vi "AlliGator Settings Window.vi"() -> ()   [LabVIEW 2021, in "AlliGator Settings.lvlib"]
doc: "GUI providing access to settings parameters for all aspect of AlliGator's functions."
uses:
  AlliGator Settings.lvlib
  AlliGator Phasor Plot Size.ctl
  AlliGator Gates to Skip.ctl
  Graphs/XY Graph/XY Graph Plot Shift Parameters.ctl
  Graphs/XY Graph/XY Graph Plot Shift Method.ctl
  Image/Image Save File Format.ctl
  AlliGator Low Count Pixels Rejection Options.ctl
  Phasor/Phasor Ratio Type.ctl
  AlliGator Baseline Subtraction Method.ctl
  Fits/IRF(X)PSED/Decay Fit Options v2.ctl
  Fits/Decay Convolution/Decay Model.ctl
  Fits/Residual Type.ctl
  Fits/IRF(X)PSED/Fit Weights Type.ctl
  Fits/Non-linear Fitting Method v2.ctl
  Fits/Fit Calculation Method.ctl
  Fits/Non-linear Fitting Algorithm.ctl
  Fits/IRF(X)PSED/Decay Fit Parameters & Derived Quantities List.ctl
  AlliGator Decay Fit Parameter Constraints 2.ctl
  Fits/IRF(X)PSED/Decay Fit Parameters In List.ctl
  AlliGator IRF Optimization Controls.ctl
  AlliGator IRF Deconvolution Metrics.ctl
  Math/Advanced Signal Processing Toolkit/Wavelet Analysis Options.ctl
  AlliGator High Count Pixels Rejection Options.ctl
  AlliGator Image Smoothing Options.ctl
  Arrays/Kernel Type.ctl
  Arrays/Smoothing Algorithm.ctl
  Fits/Square Pulse/Square Pulse Options.ctl
  Fits/Square Pulse/Square Pulse Levels Type.ctl
  AlliGator Image Binning Options.ctl
  AlliGator Phasor Plot Smoothing Options.ctl
  AlliGator Phasor Plot Graphics Options.ctl
  AlliGator Exported Image Settings.ctl
  Fits/IRF(X)PSED/IRF(X)PSED Extraction Options.ctl
  Fits/IRF(X)PSED/Fourier Series Smoothing Option.ctl
  Fits/IRF(X)PSED/Fourier Series Truncation.ctl
  Fits/IRF(X)PSED/IRF Extraction Method.ctl
  Phasor/Phasor Explorer Display Parameters.ctl
  Phasor/Phasor Type of Series.ctl
  Phasor/Phasor Explorer Decay Parameters.ctl
  Phasor/Phasor IRF Model.ctl
  Phasor/Phasor Explorer Phasor Parameters.ctl
  Phasor/Phasor Calculation Type.ctl
  Phasor/Phasor SEPL Type.ctl
  Phasor/Phasor Explorer Gate Parameters.ctl
  Phasor/Phasor Gate Type.ctl
  Phasor/Phasor Type of User-defined Function.ctl
  Phasor/Phasor Explorer Gate Parameter to Adjust.ctl
  AlliGator Define Gates to.ctl
  AlliGator Gates to Keep.ctl
  AlliGator Phasor Ratio Color-Coded Quantity.ctl
  Phasor/Phasor Calibration Type.ctl
  Histograms/Linear Histogram Options.ctl
  Histograms/Histogram Bin Option.ctl
  Histograms/Histogram Bin Position.ctl
  AlliGator Gate Arithmetic.ctl
  AlliGator Phasor Reference Associated with Shortest Lifetime.ctl
  AlliGator Python Settings.ctl
  SwissSPAD/SwissSPAD Live_Image Display Options.ctl
  AlliGator Average Lifetime Options.ctl
  AlliGator Calibration Map Algorithm.ctl
  AlliGator Guess Parameters Options.ctl
  Phasor/Phasor Standard Deviation Options.ctl
  AlliGator Source Image Scale Bar Options.ctl
  Fits/IRF(X)PSED/MLE Baseline Offset Type.ctl
  Image/Flatfield Correction Options.ctl
  AlliGator Settings Q Element.ctl
  AlliGator Settings Q Action.ctl
  AlliGator Refnums List.ctl
  AlliGator Settings List.ctl
  AlliGator Variables List.ctl
  Image/Image Hot Pixel Map Target.ctl
  AlliGator Q Element.ctl
  AlliGator Q Event.ctl
  Palette/Image Palette Information.ctl
  Image/Image Display Palette Type.ctl
  Notebook/Notebook Parameters List.ctl
  AlliGator Skippable Windows Status.ctl
  AlliGator Quantities.ctl
  f3e5a785-d283-42c9-a630-fb32b7f70655.vi
  c46dad3f-f40e-47bf-8043-7fc63249f95d.vi
  Variant/Variant to Data/Variant to [String].vi
  Variant/Variant to Data/Variant to I32.vi
  Variant/Variant to Data/Variant to Boolean.vi
  Formula/Aliases Definition Window.vi
  Variant/Variant to Data/Variant to U16.vi
  Variant/Variant to Data/Variant to String.vi
  Variant/Variant to Data/Variant to Path.vi
  AlliGator Action Engine.lvlib
  AlliGator Globals, Variables & Constants.lvlib
  Variant/Variant to Data/Variant to Data.lvlib
  Palette/Palette.lvlib
  Image/Image.lvlib
  AlliGator GUI.lvlib
  AlliGator Phasor Plot.lvlib
  AlliGator Phasor Graph.lvlib
  Error/Error.lvlib
  Graphs/Plot Editor/Plot Editor.lvlib
  Phasor/Phasor Explorer.lvlib
  AlliGator Phasor Ratio.lvlib
  Utilities/Utilities.lvlib
  <vilib>/vision/NI_Vision_Development_Module.lvlib
  AlliGator Python Plugins.lvlib
  Notebook/Notebook.lvlib
  SwissSPAD/SwissSPAD Live.lvlib
  Formula/Formula.lvlib
  Fits/Fits.lvlib
  Phasor/Phasor.lvlib
  AlliGator Decay Analysis.lvlib
  Graphs/XY Graph/XY Graph Add-Ons.lvlib
  AlliGator Decay Fit.lvlib
  AlliGator IRF.lvlib
  Math/Math.lvlib
  Arrays/Arrays.lvlib
  AlliGator Source Image.lvlib
  Histograms/Histogram Window.lvlib
  AlliGator Phasor Calibration.lvlib
  AlliGator Decay Preprocessing.lvlib
panel:
  in  "Flatfield Correction":T1={"Flatfield Estimation Options"={"Sampling Grid Size X"=256, "Sampling Grid Size Y"=256, "Polynomial Degree"=5}, "Background Options"={"Estimate Background"=TRUE, "Background Estimation Size"=32, "Niblack Deviation Factor [0. 1]"=0.2}, "Correction Factor"=1.1} {"Background Options"."Niblack Deviation Factor [0. 1]" min=0.0 max=1.0}
  in  "Settings Tabs":T2(tab)
  in  "Source Image Tabs":T3(tab)
  in  "Hot Pixel Removal":T4 caption="Hot Pixel Removal (*)" {"Percentile" min=0 max=100}
  in  "Use Image Histogram for Contrast":bool=TRUE
  in  "Low Count Pixels Rejection Options":T5={"Background Low Threshold Factor"=0.0, "Fixed Low Background Threshold"=20000.0, "Reject Low Count Pixels"=FALSE, "Low Percentile"=0.0} {"Low Percentile" min=0.0 max=100.0}
  in  "High Count Pixels Rejection Options":T6={"Background High Threshold Factor"=0.0, "Fixed High Background Threshold"=1.0, "Reject High Count Pixels"=FALSE, "High Percentile"=100.0} {"High Percentile" min=0.0 max=100.0}
  in  "ROI Creation":string="ROI Creation"
  in  "Image Pre-Processing Operations Order":u16(ring) items=["Remove Screamers", "Pile-up Correction", "Binning", "Smoothing", "Rescaling"]
  in  "Dead Left Columns Correction":bool
  in  "ROI Diameter":i32=12
  in  "Use Fixed ROI Diameter":bool
  in  "ROI Center Color":u32(colorbox)=16711680
  in  "Peak Threshold":dbl=500.0
  in  "Image Smoothing Options":T7={"Use Image Smoothing"=FALSE, "Kernel Type"=enum."Bilinear", "Bin"=1, "Algorithm"=enum."Rapid"} caption="Image Smoothing Options (*)" {"Bin" min=1}
  in  "Image Binning Options":T10={"Use Image Binning"=FALSE, "X Bin"=1, "Y Bin"=1} caption="Image Binning Options (*)" {"Y Bin" min=1; "X Bin" min=1}
  in  "Invert Binary Mask":bool
  in  "Intensity Threshold":dbl=500.0
  in  "Overlay Analyzed ROI Center":bool
  in  "Save Source Image":bool caption="Save Image"
  in  "Use Image Brightness":bool=TRUE
  in  "Blend Overlay with Image Background":bool=TRUE
  in  "Scale Bar Options":T11 caption="Scale Bar Options (*)"
  in  "Image Resolution (Pixel Size)":dbl[unit]
  in  "Dataset Scaling Factor":dbl=1.0 caption="Scaling Factor" min=0.0
  in  "Gate Image Integration":dbl[unit]=3e-10 min=0.0 format="%#.3g"
  in  "Gate Image Exposure":dbl[unit]=3e-10 min=0.0 format="%#.3g"
  in  "Available Channel Names":string[](array[string])
  in  "Background File Subtraction":bool
  in  "Background Scaling Factor":dbl=1.0 caption="Scaling Factor" min=0.0
  in  "Background File":path caption="Background Dataset"
  in  "Background Pile-up Correction":bool caption="Pile-up Correction"
  in  "Background Pixel Well Capacity":u32=1 caption="Max Value" min=1 step=1
  in  "Pixel Well Capacity":u32=1 caption="Max Value" min=1 step=1
  in  "Pile-up Correction":bool
  in  "Channel Arithmetic":T12 caption="Channel Arithmetic (*)"
  in  "Channel Name":u16(ring) items=["Gate"]
  in  "Gates to Keep":T13={"First"=0, "Last"=4294967295} caption="Gates to Keep (*)"
  in  "Define Gates to":T14 caption="Define Gates to (*)"
  in  "SYNC Period":dbl[unit] min=0.0 format="%#.3g"
  out "Natural Frequency":dbl[unit] min=0.0 format="%#.3g"
  in  "# Gates":u32=1 min=1 step=1
  in  "Gate Step":u32=1 caption="Gate Step (*)" min=1 step=1
  in  "Gate Width":dbl[unit]=3e-10 min=0.0 format="%#.3g"
  in  "Nanotime Gate Separation":dbl[unit]=4e-11 caption="Gate Separation" min=0.0 format="%#.3g"
  in  "Gates to Skip":T15 caption="Gates to Skip (*)"
  in  "Laser Period":dbl[unit] min=0.0 format="%#.3g"
  in  "Fluorescence Decay Tabs":T16(tab) caption="Fluorescence Decay Tab"
  in  "[0-1]-Normalize Decay":bool caption="1- Normalize Decay"
  in  "# Folds":u32=1 min=1
  in  "Fold Decay":bool caption="Straighten Decay"
  in  "Use Decay Pre-Processing":bool=TRUE
  in  "Head Fraction":dbl min=0.0 max=1.0 format="%.4g"
  in  "Use Cursors":bool
  in  "Use Periodicity":bool
  in  "Pixel-Normalize Decay":bool
  in  "Constant Background":dbl=1.0
  in  "Verbose Decay Pre-Processing":bool=TRUE
  in  "Decay Pre-Processing Operations Order":u16(ring) items=["Background subtraction", "Revert", "Smoothen", "Straighten", "Shift", "Extrapolate", "Normalize", "Fold"]
  in  "Straighten Decay":bool
  in  "Background Subtraction":bool=TRUE
  in  "Baseline Subtraction Method":T17=enum."Min"
  in  "Background Definition Range":T18={"Min Gate"=0.0, "Max Gate"=8e-10} {"Max Gate" min=0.0 format="%#_5g"; "Min Gate" min=0.0 format="%#_5g"}
  in  "Additional Points":u32
  in  "Tail Fraction":dbl min=0.0 max=1.0 format="%.4g"
  in  "Extrapolate Decay":bool
  in  "Shift Decay":bool
  in  "Smoothen Decay":bool
  in  "Smoothing Parameter":dbl=-1.0 min=0.0 max=1.0
  in  "1-Normalize Decay":bool caption="1- Normalize Decay"
  in  "Decay Shift Parameters":T19
  in  "Reverse Gates":bool
  in  "Average Lifetime Options":T21={"Use Local IRF "=TRUE, "Use IRF Offset"=TRUE, "Use Fixed Offset"=TRUE, "Fixed Offset"=0.0, "Baseline %"=0.0} caption="Use Local IRF" {"Baseline %" min=0.0 max=100.0}
  in  "IRF Extraction Options":T22={"Time Constant for IRF Extraction"=1e-18, "IRF Order"=1, "Fourier Series Smoothing"=enum."None", "Noise Threshold"=0.0, "Smoothing Width"=0.0, "Fourier Series Truncation"=enum."Automatic", "Truncation Order"=0, "Save Power Spectrum"=FALSE, "Smoothing"=FALSE, "Smoothing Parameter"=0.0, "Smoothing Order"=1, "Method"=enum."Direct"} {"Smoothing Order" min=1 max=100; "Smoothing Parameter" min=-1.0 max=1.0; "Time Constant for IRF Extraction" min=0.0 format="%#_5g"}
  in  "IRF Optimization Options":T26={"Search Range"=1e-18, "Search Step"=1e-09, "Tail Threshold (%)"=1e-09, "Regularized IRF"=FALSE, "Export Plot"=FALSE, "Export Data"=FALSE, "Smooth Metrics"=FALSE, "S-G Side Points"=1, "S-G Polynomial Order"=3, "Metrics"=enum."Average"} {"S-G Polynomial Order" min=3 max=10; "S-G Side Points" min=1; "Tail Threshold (%)" min=0.0 max=100.0; "Search Step" min=0.0; "Search Range" min=0.0}
  in  "Square Pulse Options":T28={"Method"=enum."Mode", "# Bins"=0, "Threshold %"=10.0, "Center on Midpoint"=FALSE, "Smoothen Plot"=FALSE} {"Threshold %" min=0.0 max=100.0}
  in  "Wavelet Analysis Options":T30={"Wavelet"=enum."db02", "Option for Approximate Coefficients"=enum."None", "# Levels"=1, "Threshold Settings"={"Thresholding Rule"=enum."Universal", "Rescaling Method"=enum."Single level", "Soft Threshold?"=TRUE}, "Wavelet Transform Type"=enum."Discrete"}
  in  "Extract IRF instead of Decay":bool
  in  "Use Data Information Laser Period":bool
  in  "Use Legacy Fitting Approach":bool
  in  "Fit Options":T31={"Show Fit Residuals"=TRUE, "Fit Model"=enum."1-Exponential", "Residual Type"=enum."Standard", "Max Decay Percentile"=1.0, "Min Decay Percentile"=0.0, "Show Full Decay"=TRUE, "Weights"=enum."1/Variance", "Fitting Method"=enum."Least Square", "Compute Parameter Uncertainties"=TRUE, "Periodic Boundaries"=FALSE, "Model Calculation"=enum."Simulation", "Period"=1.2500000000000001e-08, "Termination Criteria"={"Max Iterations"=1000, "Max Function Calls"=0, "Max Time"=1000.0, "Function Tolerance"=1e-06, "Parameter Tolerance"=1e-06, "Gradient Tolerance"=0.0, "Min Lambda"=1e-06, "Max Lambda"=1e-06, "Initial Tick Count"=0}, "Offset Resolution"=4e-11, "Use Local IRF"=TRUE, "Fitting Algorithm"=enum."Levenberg-Marquardt"} {"Offset Resolution" min=0.0; "Period" min=0.0; "Min Decay Percentile" min=0.0 max=100.0; "Max Decay Percentile" min=0.0 max=100.0}
  in  "MLE Baseline Offset Type":T38
  in  "MLE Baseline Offset":dbl
  in  "Guess Parameters Options":T39 caption="Options"
  in  "Use Last Fitted Parameters":bool
  in  "Guess Parameter Names":T40[](array[typedef]) caption="Names"
  in  "Use Guess Parameters":bool
  in  "Guess Parameter Values":dbl[](array[numeric]) caption="Values"
  in  "Fit Parameter Constraints":T41[](array[typedef]) {"Max Value" format="%#.3g"; "Min Value" format="%#.3g"}
  in  "Displayed Fit Parameters":T42[](array[typedef])
  in  "Export Tabulated Results":bool=TRUE
  in  "Fluorescence Decay Graph Default Plot Style":cluster{"X":dbl, "Y":dbl}[](graph) caption="Phasor Graph Default Plot Style"
  in  "Decay Graph Color Array":u32[](array[colorbox])
  in  "Show Last Decay Only":bool caption="Show Last Decay only"
  in  "Max Peak Value":dbl
  in  "Reject High Decay Peak Pixels":bool
  in  "Min Peak Value":dbl
  in  "Reject Low Decay Peak Pixels":bool
  in  "Intensity Correction File":path
  in  "Use Intensity Correction File":bool
  in  "Use File Timestamp":bool
  in  "Time Step":dbl[unit]=1.0
  in  "Phasor Plot Tabs":T43(tab)
  in  "Phasor Plot Smoothing Options":T44={"Use Phasor Plot Smoothing"=FALSE, "Kernel Type"=enum."Uniform", "Bin"=1, "Algorithm"=enum."Rapid"} {"Bin" min=1 step=2}
  in  "Phasor Plot Frequency":dbl[unit]=80000000.0 caption="Phasor Frequency"
  in  "Selected Image ROI(s)":bool
  in  "All Image ROIs":bool
  in  "Selected Phasor Plot ROI(s)":bool
  in  "All Phasor Plot ROIs":bool
  in  "Cumulative Phasor Plot":bool
  in  "Store Phasor Harmonics":bool
  in  "Phasor Ratio Decay Range":dbl=1.0 caption="Decay Range"
  in  "Phasor Ratio Reference Colors":T45={"Reference 1"=3381759, "Reference 2"=3381759, "Boundary"=3381759} caption="Reference Colors"
  in  "Exponential Fading":bool
  in  "Phasor Ratio Color Map Type":T46(radio) caption="Color Map Type"
  out "Phasor Ratio Color Map":string caption="Average Lifetime Color Map"
  in  "Phasor Ratio Color Scale":dbl(ramp) caption="Average Lifetime Color Scale"
  out "Ref 2 Label":string="Ref 1"
  out "Ref 1 Label":string="Ref 2"
  in  "Phasor Ratio Display Range":cluster{dbl, dbl}(slide)={0.0, 454.0} caption="Average Lifetime Display Range" scale=0.5..1.5 scale format="%#.3g"
  in  "Reference Radius":i32=512 min=1
  in  "Phasor Ratio Color-Coded Quantity":T47 caption="Displayed Quantity"
  in  "Draw Reference Segment":bool
  in  "User-Defined Quantity":string
  in  "Blend Overlay with Phasor Background":bool=TRUE
  in  "Use Phasor Brightness":bool
  in  "Phasor Plot Size":T48={"H"=512, "V"=512, "Margin"=0.2} {"Margin" min=0.0}
  in  "Phasor Plot Graphics Options":T49={"UC Color"=3381759, "Show UC Tau Ticks"=FALSE, "SEPL Color"=3381759, "Show SEPL Tau Ticks"=FALSE, "Axes Color"=16776960, "Show (g,s) Ticks"=FALSE, "Show UC"=FALSE, "Show SEPL"=FALSE, "Show Axes"=FALSE, "Show UC Tau Labels"=FALSE, "Show SEPL Tau Labels"=FALSE, "Show (g,s) Labels"=FALSE, "UC Label Size"=18, "UC Label Distance"=0.0, "SEPL Label Size"=18, "SEPL Label Distance"=0.0, "Axes Label Size"=18, "Axes Label Distance"=0.0}
  in  "Define Shortest Lifetime as":T50
  in  "Save Phasor Graph Image":bool
  in  "Phasor Graph Frequency":dbl[unit]=80000000.0 caption="Phasor Frequency"
  in  "Phasor Ratio Type":T51
  in  "Pixel-level Phasor Computation":bool
  in  "Phasor SDV Options":T52={"Compute Estimated SDV"=FALSE, "# Replicas"=100, "Use Estimated Average Phasor"=FALSE}
  in  "SEPL Tabs":enum32{"Display", "Phasor", "IRF", "Gates"}(tab)
  in  "Display Parameters":T53={"# Points"=1000, "Ramp Type"=enum."Logarithmic", "Type of Series"=enum."1-Exp Decays", "Min tau"=1.0000000000000002e-12, "Max tau"=1.0000000000000001e-07, "Include 0"=FALSE, "Include Infinity"=FALSE} {"Min tau" min=0.0; "Max tau" min=0.0; "# Points" min=1 step=1}
  in  "Phasor Parameters":T55={"Harmonic Frequency"=0.0, "Use f* = 1/D Frequency"=FALSE, "Calibrated Phasor"=FALSE, "Calibration Lifetime"=1e-09, "Phasor Calculation"=enum."Direct Sum", "SEPL Type"=enum."UC", "# Gates"=1.0, "Square Gate Width"=1e-09, "Show Ticks"=FALSE} {"Square Gate Width" min=0.0; "# Gates" min=0.0; "Calibration Lifetime" min=0.0; "Harmonic Frequency" min=0.0}
  in  "Decay & IRF Parameters":T58={"Lifetime"=3.0000000000000004e-09, "IRF Offset"=0.0, "IRF Period"=1.2500000000000001e-08, "Normalized Decays"=FALSE, "IRF Model"=enum."Dirac", "IRF Parameter 1"=0.0} caption="IRF Parameters" {"Lifetime" min=0.0; "IRF Period" min=0.0}
  in  "Edit User-defined Function":bool caption="Edit User-defined Gate"
  in  "Gate Parameter to Adjust":T60 caption="Adjust"
  in  "Match Laser Period":bool=TRUE
  in  "Gate Parameters":T61={"First Gate Start"=0.0, "Use Gate Center"=FALSE, "Gate Width"=0.0, "Gate Step"=0.0, "# Gates"=1.0, "Gate Type"=enum."Square", "Edge Width"=0.0, "Top Slope"=0.0, "Reversed Sawtooth?"=FALSE, "Analytical Computation"=FALSE, "Integration"=enum."Item 0", "Tolerance"=1.0, "# Steps"=1.0, "Type of User-defined Function"=enum."Gate", "Use Gate Step"=FALSE} {"# Steps" min=0.0; "Tolerance" min=0.0; "Top Slope" min=0.0; "Edge Width" min=0.0; "Gate Step" min=0.0; "# Gates" min=1.0 step=1.0; "Gate Width" min=0.0}
  in  "Use Current Dataset Parameters":bool
  in  "Calibration Map Algorithm":T64
  in  "Calibration Type":T65=enum."Single Phasor"
  in  "Backup Calibration Type":T66(ring) caption="Backup Calibration"
  in  "Use Backup Calibration if needed":bool=TRUE
  in  "Calibration Lifetime":dbl[unit]=1e-09
  in  "Lifetime Analysis Graph Default Plot Style":cluster{"X":dbl, "Y":dbl}[](graph) caption="Phasor Graph Default Plot Style"
  in  "Decay Analysis Parameters":T19
  in  "Plugins Folder":bool
  in  "Parameter Names only":bool
  in  "Send JSON to Clipboard":bool
  in  "Reset Python Session":bool
  out "Valid Python Session":bool
  in  "Python Settings":T67
  in  "Transparent Mask Color":u32(colorbox)
  in  "ROI Description Max Characters":i32=256
  in  "Beep on Error":bool caption="Verbose Error Mode"
  in  "# Logical Processors Used":i32 caption="Used" min=1 max=16
  out "# Logical Processors":i32
  in  "Histogram Options":T68={"Bin Size"=0.0, "Bin Number"=0, "Bin Option"=enum."Bin Number", "Min Value"=-inf, "Max Value"=inf, "Filter NaN & Infinite Values"=TRUE, "Frequency Plot"=FALSE, "Align Bins"=FALSE, "Bin Location"=enum."Left", "Project Outside Values"=FALSE, "Max Histogram Size"=100000} {"Max Histogram Size" format="%.0e"}
  in  "Exported Gate Image Settings":T71
  in  "Restore Skipped Dialogs":bool
  in  "Verbose Error Mode":bool
  in  "Verbose Settings Mode":bool
  in  "Beep after Script":bool
  in  "Include Loading in Timing":bool
  in  "Verbose Mode":bool
  in  "Saved Displayed Image File Format":T72
  # "Image ROI"
  # "Gates Characteristics"
  # "Dataset Pile-up Correction (*)"
  # "Background File Subtraction (*)"
  # "Guess Parameters"
  # "Limit Phasor Plot Calculation  to:"
  # "Limit Phasor Plot Analysis  to:"
  # "Phasor Ratio/Average Lifetime Style Options"
  # "Phasor Plot Size & Style"
  # "Calibration Options"
  # "Image Saving Options"
  # "UI Options"
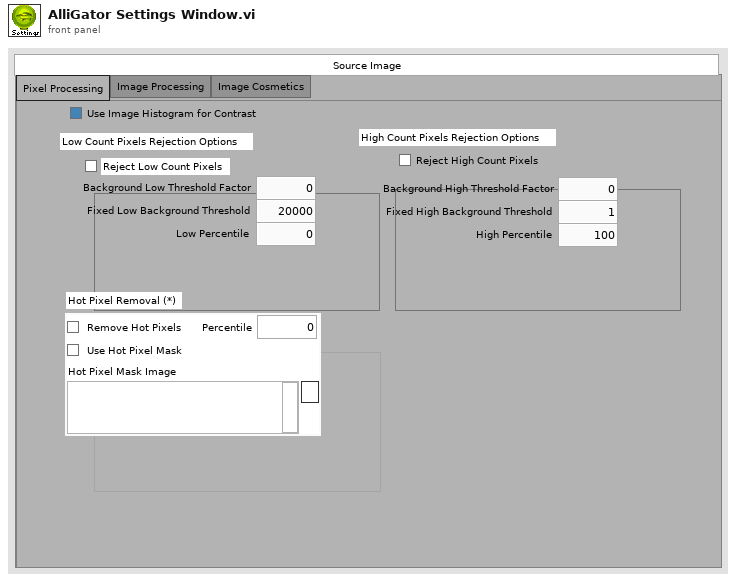
[diagram p1: front panel]
types:
  T1 = typedef "Image.lvlib/Flatfield Correction Options.ctl" = cluster{"Flatfield Estimation Options":cluster{"Sampling Grid Size X":i32, "Sampling Grid Size Y":i32, "Polynomial Degree":i32}, "Background Options":cluster{"Estimate Background":bool, "Background Estimation Size":i32, "Niblack Deviation Factor [0. 1]":dbl}, "Correction Factor":sgl}
  T2 = enum32{"Source Image", "Data Information", "Fluorescence Decay", "Fluorescence Decay Statistics", "Intensity Time Trace", "Phasor Plot", "Phasor Graph", "Single-Exponential Phasor Locus (SEPL)", "Phasor Calibration", "Lifetime Analysis", "Plugins", "Miscellaneous"}
  T3 = enum32{"Pixel Processing", "Image Processing", "Image Cosmetics"}
  T4 = typedef "SwissSPAD Live.lvlib/SwissSPAD Live_Image Display Options.ctl" = cluster{"Remove Screamers":bool, "Delta":sgl, "Equalize Histogram":bool, "Percentile":sgl, "Hot Pixel Mask Image":path, "Use Hot Pixel Mask":bool}
  T5 = typedef "AlliGator Settings.lvlib/AlliGator Low Count Pixels Rejection Options.ctl" = cluster{"Background Low Threshold Factor":dbl, "Fixed Low Background Threshold":dbl, "Reject Low Count Pixels":bool, "Low Percentile":dbl}
  T6 = typedef "AlliGator Settings.lvlib/AlliGator High Count Pixels Rejection Options.ctl" = cluster{"Background High Threshold Factor":dbl, "Fixed High Background Threshold":dbl, "Reject High Count Pixels":bool, "High Percentile":dbl}
  T7 = typedef "AlliGator Settings.lvlib/AlliGator Image Smoothing Options.ctl" = cluster{"Use Image Smoothing":bool, "Kernel Type":T8, "Bin":i32, "Algorithm":T9}
  T8 = typedef "Arrays.lvlib/Kernel Type.ctl" = enum16{"Uniform", "Bilinear", "Gaussian"}
  T9 = typedef "Arrays.lvlib/Smoothing Algorithm.ctl" = enum16{"Rapid", "Thorough"}
  T10 = typedef "AlliGator Source Image.lvlib/AlliGator Image Binning Options.ctl" = cluster{"Use Image Binning":bool, "X Bin":i32, "Y Bin":i32}
  T11 = typedef "AlliGator Source Image.lvlib/AlliGator Source Image Scale Bar Options.ctl" = cluster{"Show Scale Bar Overlay":bool, "Scale Bar Length":dbl[unit], "Scale Bar Color":u32, "Scale Bar X":u32, "Scale Bar Y":u32, "Scale Bar Height":dbl[unit]}
  T12 = typedef "AlliGator Settings.lvlib/AlliGator Gate Arithmetic.ctl" = enum16{"None", "INT-G2", "G2/INT*<INT>", "(1 - G2/INT)*<INT>"}
  T13 = typedef "AlliGator Settings.lvlib/AlliGator Gates to Keep.ctl" = cluster{"First":u32, "Last":u32}
  T14 = typedef "AlliGator Settings.lvlib/AlliGator Define Gates to.ctl" = enum32{"Skip", "Keep"}
  T15 = typedef "AlliGator Decay Analysis.lvlib/AlliGator Gates to Skip.ctl" = cluster{"Start":u32, "End":u32}
  T16 = enum32{"Decay Pre-Processing", "Advanced Analysis", "Fit Options", "Fit Parameters", "Styles"}
  T17 = typedef "AlliGator Decay Analysis.lvlib/AlliGator Decay Preprocessing.lvlib/AlliGator Baseline Subtraction Method.ctl" = enum16{"Mean", "Min", "Square Gated Single-Exponential", "File", "Constant"}
  T18 = cluster{"Min Gate":dbl[unit], "Max Gate":dbl[unit]}
  T19 = typedef "XY Graph Add-Ons.lvlib/XY Graph Plot Shift Parameters.ctl" = cluster{"Type":T20, "Shift":dbl[unit], "Threshold":dbl, "Rotate":bool}
  T20 = typedef "XY Graph Add-Ons.lvlib/XY Graph Plot Shift Method.ctl" = enum16{"Default", "CFD", "Threshold", "Cross-Correlation"}
  T21 = typedef "AlliGator Settings.lvlib/AlliGator Average Lifetime Options.ctl" = cluster{"Use Local IRF ":bool, "Use IRF Offset":bool, "Use Fixed Offset":bool, "Fixed Offset":dbl[unit], "Baseline %":dbl}
  T22 = typedef "Fits.lvlib/IRF(X)PSED Extraction Options.ctl" = cluster{"Time Constant for IRF Extraction":dbl[unit], "IRF Order":i32, "Fourier Series Smoothing":T23, "Noise Threshold":dbl, "Smoothing Width":dbl, "Fourier Series Truncation":T24, "Truncation Order":i32, "Save Power Spectrum":bool, "Smoothing":bool, "Smoothing Parameter":dbl, "Smoothing Order":u32, "Method":T25}
  T23 = typedef "Fits.lvlib/Fourier Series Smoothing Option.ctl" = enum16{"None", "Lanczos Factors", "Fejer Summation"}
  T24 = typedef "Fits.lvlib/Fourier Series Truncation.ctl" = enum16{"Automatic", "Fixed"}
  T25 = typedef "Fits.lvlib/IRF Extraction Method.ctl" = enum16{"Direct", "Topless", "Toeplitz"}
  T26 = typedef "AlliGator Decay Analysis.lvlib/AlliGator IRF.lvlib/AlliGator IRF Optimization Controls.ctl" = cluster{"Search Range":dbl[unit], "Search Step":dbl[unit], "Tail Threshold (%)":dbl, "Regularized IRF":bool, "Export Plot":bool, "Export Data":bool, "Smooth Metrics":bool, "S-G Side Points":i32, "S-G Polynomial Order":i32, "Metrics":T27}
  T27 = typedef "AlliGator Decay Analysis.lvlib/AlliGator IRF.lvlib/AlliGator IRF Deconvolution Metrics.ctl" = enum16{"Average", "SDV", "Max", "Average * SDV", "Slope"}
  T28 = typedef "Fits.lvlib/Square Pulse Options.ctl" = cluster{"Method":T29, "# Bins":i32, "Threshold %":dbl, "Center on Midpoint":bool, "Smoothen Plot":bool}
  T29 = typedef "Fits.lvlib/Square Pulse Levels Type.ctl" = enum16{"Mode", "Mean"}
  T30 = typedef "Math.lvlib/Wavelet Analysis Options.ctl" = cluster{"Wavelet":enum16{"db02", "db03", "db04", "db05", "db06", "db07", "db08", "db09", "db10", "db11", "db12", "db13", "db14", "Haar", "bior1_3", "bior1_5", "bior2_2", "bior2_4", "bior2_6", "bior2_8", "bior3_1", "bior3_3", "bior3_5", "bior3_7", "bior3_9", "bior4_4 (FBI)", "bior5_5", "bior6_8", "coif1", "coif2", "coif3", "coif4", "coif5", "sym2", "sym3", "sym4", "sym5", "sym6", "sym7", "sym8"}, "Option for Approximate Coefficients":enum16{"None", "Threshold", "Detrend"}, "# Levels":i32, "Threshold Settings":cluster{"Thresholding Rule":enum16{"SURE", "Hybrid", "Universal", "Minimax"}, "Rescaling Method":enum16{"One", "Single level", "Multiple levels"}, "Soft Threshold?":bool}, "Wavelet Transform Type":enum16{"Discrete", "Undecimated"}}
  T31 = typedef "Fits.lvlib/Decay Fit Options v2.ctl" = cluster{"Show Fit Residuals":bool, "Fit Model":T32, "Residual Type":T33, "Max Decay Percentile":dbl, "Min Decay Percentile":dbl, "Show Full Decay":bool, "Weights":T34, "Fitting Method":T35, "Compute Parameter Uncertainties":bool, "Periodic Boundaries":bool, "Model Calculation":T36, "Period":dbl[unit], "Termination Criteria":cluster{"Max Iterations":i32, "Max Function Calls":i32, "Max Time":dbl[unit], "Function Tolerance":dbl, "Parameter Tolerance":dbl, "Gradient Tolerance":dbl, "Min Lambda":dbl, "Max Lambda":dbl, "Initial Tick Count":u32}, "Offset Resolution":dbl[unit], "Use Local IRF":bool, "Fitting Algorithm":T37}
  T32 = typedef "Fits.lvlib/Decay Model.ctl" = enum16{"1-Exponential", "2-Exponentials"}
  T33 = typedef "Fits.lvlib/Residual Type.ctl" = enum16{"Standard", "Normalized", "Reduced"}
  T34 = typedef "Fits.lvlib/Fit Weights Type.ctl" = enum16{"Unweighted", "1/Variance", "Best of All"}
  T35 = typedef "Fits.lvlib/Non-linear Fitting Method v2.ctl" = enum16{"Least Square", "Least Absolute Residual", "Bisquare", "MLE", "-", "Best of All"}
  T36 = typedef "Fits.lvlib/Fit Calculation Method.ctl" = enum16{"Simulation", "Convolution", "Integration"}
  T37 = typedef "Fits.lvlib/Non-linear Fitting Algorithm.ctl" = enum16{"Levenberg-Marquardt", "Trust-Region Dogleg"}
  T38 = typedef "Fits.lvlib/MLE Baseline Offset Type.ctl" = enum32{"Absolute", "Percentage"}
  T39 = typedef "AlliGator Decay Analysis.lvlib/AlliGator Decay Fit.lvlib/AlliGator Guess Parameters Options.ctl" = enum16{"Numerically estimated", "User-provided", "User-provided (normalized)", "Last valid fitted parameters"}
  T40 = typedef "Fits.lvlib/Decay Fit Parameters In List.ctl" = enum16{"Offset", "Baseline", "A_1", "tau_1", "A_2", "tau_2"}
  T41 = typedef "AlliGator Decay Analysis.lvlib/AlliGator Decay Fit.lvlib/AlliGator Decay Fit Parameter Constraints 2.ctl" = cluster{"Fit Parameter":T40, "Min Value":dbl, "Max Value":dbl, "Global":bool, "Used":bool}
  T42 = typedef "Fits.lvlib/Decay Fit Parameters & Derived Quantities List.ctl" = enum16{"Offset", "Baseline", "A_1", "tau_1", "A_2", "tau_2", "<tau>_a", "f1_a", "f2_a", "<tau>_i", "f1_i", "f2_i", "-", "R^2", "Chi^2"}
  T43 = enum32{"Phasor Plot Calculation", "Phasor Plot Information Overlay", "Phasor Plot Appearance"}
  T44 = typedef "AlliGator Phasor Plot.lvlib/AlliGator Phasor Plot Smoothing Options.ctl" = cluster{"Use Phasor Plot Smoothing":bool, "Kernel Type":T8, "Bin":i32, "Algorithm":T9}
  T45 = cluster{"Reference 1":u32, "Reference 2":u32, "Boundary":u32}
  T46 = enum32{"Interpolate Reference Colors", "Use Custom Map"}
  T47 = typedef "AlliGator Phasor Ratio.lvlib/AlliGator Phasor Ratio Color-Coded Quantity.ctl" = enum16{"Phasor Ratio (f1 or a1)", "Average Lifetime (<tau>_i or <tau>_a))", "User-Defined Quantity"}
  T48 = typedef "AlliGator Phasor Plot.lvlib/AlliGator Phasor Plot Size.ctl" = cluster{"H":i32, "V":i32, "Margin":dbl}
  T49 = typedef "AlliGator Settings.lvlib/AlliGator Phasor Plot Graphics Options.ctl" = cluster{"UC Color":u32, "Show UC Tau Ticks":bool, "SEPL Color":u32, "Show SEPL Tau Ticks":bool, "Axes Color":u32, "Show (g,s) Ticks":bool, "Show UC":bool, "Show SEPL":bool, "Show Axes":bool, "Show UC Tau Labels":bool, "Show SEPL Tau Labels":bool, "Show (g,s) Labels":bool, "UC Label Size":i16, "UC Label Distance":dbl, "SEPL Label Size":i16, "SEPL Label Distance":dbl, "Axes Label Size":i16, "Axes Label Distance":dbl}
  T50 = typedef "AlliGator Phasor Ratio.lvlib/AlliGator Phasor Reference Associated with Shortest Lifetime.ctl" = enum32{"Reference 1", "Reference 2"}
  T51 = typedef "Phasor.lvlib/Phasor Ratio Type.ctl" = enum32{"Intensity-weighted", "Amplitude-weighted"}
  T52 = typedef "Phasor.lvlib/Phasor Standard Deviation Options.ctl" = cluster{"Compute Estimated SDV":bool, "# Replicas":u32, "Use Estimated Average Phasor":bool}
  T53 = typedef "Phasor Explorer.lvlib/Phasor Explorer Display Parameters.ctl" = cluster{"# Points":i32, "Ramp Type":enum16{"Linear", "Logarithmic"}, "Type of Series":T54, "Min tau":dbl[unit], "Max tau":dbl[unit], "Include 0":bool, "Include Infinity":bool}
  T54 = typedef "Phasor.lvlib/Phasor Type of Series.ctl" = enum16{"1-Exp Decays", "Linear Combination of 1-Exp"}
  T55 = typedef "Phasor Explorer.lvlib/Phasor Explorer Phasor Parameters.ctl" = cluster{"Harmonic Frequency":dbl[unit], "Use f* = 1/D Frequency":bool, "Calibrated Phasor":bool, "Calibration Lifetime":dbl[unit], "Phasor Calculation":T56, "SEPL Type":T57, "# Gates":dbl, "Square Gate Width":dbl[unit], "Show Ticks":bool}
  T56 = typedef "Phasor.lvlib/Phasor Calculation Type.ctl" = enum16{"Direct Sum", "Analytical Formula"}
  T57 = typedef "Phasor.lvlib/Phasor SEPL Type.ctl" = enum16{"UC", "L_N", "L_N[W]", "L_X"}
  T58 = typedef "Phasor Explorer.lvlib/Phasor Explorer Decay Parameters.ctl" = cluster{"Lifetime":dbl[unit], "IRF Offset":dbl[unit], "IRF Period":dbl[unit], "Normalized Decays":bool, "IRF Model":T59, "IRF Parameter 1":dbl[unit]}
  T59 = typedef "Phasor.lvlib/Phasor IRF Model.ctl" = enum16{"Dirac", "Exponential"}
  T60 = typedef "Phasor Explorer.lvlib/Phasor Explorer Gate Parameter to Adjust.ctl" = enum16{"Gate Step", "# Gates"}
  T61 = typedef "Phasor Explorer.lvlib/Phasor Explorer Gate Parameters.ctl" = cluster{"First Gate Start":dbl[unit], "Use Gate Center":bool, "Gate Width":dbl[unit], "Gate Step":dbl[unit], "# Gates":dbl, "Gate Type":T62, "Edge Width":dbl[unit], "Top Slope":dbl[unit], "Reversed Sawtooth?":bool, "Analytical Computation":bool, "Integration":enum32{"Item 0", "Item 1"}, "Tolerance":dbl, "# Steps":dbl, "Type of User-defined Function":T63, "Use Gate Step":bool}
  T62 = typedef "Phasor.lvlib/Phasor Gate Type.ctl" = enum16{"Square", "Finite Edge Square", "Finite Edge, Tilted Top Square", "Triangle", "Sawtooth", "User-defined"}
  T63 = typedef "Phasor.lvlib/Phasor Type of User-defined Function.ctl" = enum16{"Gate", "IRF"}
  T64 = typedef "AlliGator Phasor Calibration.lvlib/AlliGator Calibration Map Algorithm.ctl" = enum16{"Simple Search", "Min Distance"}
  T65 = typedef "Phasor.lvlib/Phasor Calibration Type.ctl" = enum16{"None", "Single Phasor", "Phasor Series", "Phasor Map"}
  T66 = enum16{"Single Calibration", "Nearest Valid Calibration"}
  T67 = typedef "AlliGator Settings.lvlib/AlliGator Python Settings.ctl" = cluster{"Python Version":string, "Use PATH definition":bool, "Python.exe Path":path, "Include Example Plugins":bool}
  T68 = typedef "Histogram Window.lvlib/Linear Histogram Options.ctl" = cluster{"Bin Size":dbl, "Bin Number":i32, "Bin Option":T69, "Min Value":dbl, "Max Value":dbl, "Filter NaN & Infinite Values":bool, "Frequency Plot":bool, "Align Bins":bool, "Bin Location":T70, "Project Outside Values":bool, "Max Histogram Size":i32}
  T69 = typedef "Histogram Window.lvlib/Histogram Bin Option.ctl" = enum32{"Bin Number", "Bin Size"}
  T70 = typedef "Histogram Window.lvlib/Histogram Bin Position.ctl" = enum16{"Left", "Center", "Right"}
  T71 = typedef "AlliGator Settings.lvlib/AlliGator Exported Image Settings.ctl" = cluster{"bitness":bool, " Min Value":sgl, " Max Value":sgl}
  T72 = typedef "Image.lvlib/Image Save File Format.ctl" = enum16{"PNG", "JPEG", "BMP"}
  T73 = typedef "AlliGator Settings.lvlib/AlliGator Settings List.ctl" = enum16{"GUI:Visible Settings Tab", "GUI:Last Run Version", "Source Image:Use Image Histogram for Contrast", "Source Image:Low Count Pixels Rejection Options", "Source Image:High Count Pixels Rejection Options", "Source Image:Use Image Brightness", "Source Image:Blend Overlay with Image Background", "Source Image:Use Fixed ROI Diameter", "Source Image:ROI Diameter", "Source Image:ROI Center Color", "Source Image:Peak Threshold", "Source Image:Intensity Threshold", "Source Image:Image Binning Options", "Source Image:Image Smoothing Options", "Source Image:Image Histogram Active", "Source Image:Invert Binary Mask", "Source Image:Hot Pixel Removal", "Source Image:Overlay Analyzed ROI Center", "Source Image:Auto-Adjust Contrast", "Source Image:Histogram Lower Percentile", "Source Image:Histogram Upper Percentile", "Source Image:Save Source Image", "Source Image:Scale Bar Options", "Source Image:Image Resolution (Pixel Size)", "Source Image:Flatfield Correction", "Source Image:Show Dead Left Columns Correction", "Source Image:Dead Left Columns Correction", "Source Image:Image Pre-Processing Operations Order", "Data Information:Gate Width", "Data Information:Nanotime Gate Separation", "Data Information:Macrotime Gate Separation", "Data Information:Gate Step", "Data Information:# Gates", "Data Information:Gate Image Exposure", "Data Information:Gate Image Integration", "Data Information:Gates to Skip", "Data Information:Gates to Keep", "Data Information:Define Gates to", "Data Information:Channel Name", "Data Information:Available Channel Names", "Data Information:Channel Arithmetic", "Data Information:Background File Subtraction", "Data Information:Background File", "Data Information:Background Scaling Factor", "Data Information:Background Pile-up Correction", "Data Information:Background Pixel Well Capacity", "Data Information:Laser Period", "Data Information:SYNC Period", "Data Information:Pile-up Correction", "Data Information:Pixel Well Capacity", "Data Information:Dataset Scaling Factor", "Fluorescence Decay_Decay Pre-Processing:Reverse Gates", "Fluorescence Decay_Decay Pre-Processing:Verbose Decay Pre-Processing", "Fluorescence Decay_Decay Pre-Processing:Use Decay Pre-Processing", "Fluorescence Decay_Decay Pre-Processing:Background Subtraction", "Fluorescence Decay_Decay Pre-Processing:Background Definition Range", "Fluorescence Decay_Decay Pre-Processing:Baseline Subtraction Method", "Fluorescence Decay_Decay Pre-Processing:Decay Pre-Processing Operations Order", "Fluorescence Decay_Decay Pre-Processing:Smoothing Parameter", "Fluorescence Decay_Decay Pre-Processing:Shift Decay", "Fluorescence Decay_Decay Pre-Processing:Decay Shift Parameters", "Fluorescence Decay_Decay Pre-Processing:Fold Decay", "Fluorescence Decay_Decay Pre-Processing:# Folds", "Fluorescence Decay_Decay Pre-Processing:1-Normalize Decay", "Fluorescence Decay_Decay Pre-Processing:[0-1]-Normalize Decay", "Fluorescence Decay_Decay Pre-Processing:Smoothen Decay", "Fluorescence Decay_Decay Pre-Processing:Extrapolate Decay", "Fluorescence Decay_Decay Pre-Processing:Use Periodicity", "Fluorescence Decay_Decay Pre-Processing:Use Cursors", "Fluorescence Decay_Decay Pre-Processing:Tail Fraction", "Fluorescence Decay_Decay Pre-Processing:Head Fraction", "Fluorescence Decay_Decay Pre-Processing:Additional Points", "Fluorescence Decay_Decay Pre-Processing:Straighten Decay", "Fluorescence Decay_Decay Pre-Processing:Constant Background", "Fluorescence Decay_Decay Pre-Processing:Pixel-Normalize Decay", "Fluorescence Decay_Advanced Analysis:Extract IRF instead of Decay", "Fluorescence Decay_Advanced Analysis:IRF Extraction Options", "Fluorescence Decay_Advanced Analysis:IRF Optimization Options", "Fluorescence Decay_Advanced Analysis:Square Pulse Options", "Fluorescence Decay_Advanced Analysis:IRF Order", "Fluorescence Decay_Advanced Analysis:IRF Time Constants", "Fluorescence Decay_Advanced Analysis:Wavelet Analysis Options", "Fluorescence Decay_Advanced Analysis:Average Lifetime Options", "Fluorescence Decay_Fit Options:Fit Options", "Fluorescence Decay_Fit Options:Use Legacy Fitting Approach", "Fluorescence Decay_Fit Options:Use Data Information Laser Period", "Fluorescence Decay_Fit Parameters:Displayed Fit Parameters", "Fluorescence Decay_Fit Parameters:Fit Parameter Constraints", "Fluorescence Decay_Fit Parameters:Export Tabulated Results", "Fluorescence Decay_Fit Parameters:MLE Baseline Offset Type", "Fluorescence Decay_Fit Parameters:MLE Baseline Offset", "Fluorescence Decay_Fit Parameters:Guess Parameter Names", "Fluorescence Decay_Fit Parameters:Guess Parameter Values", "Fluorescence Decay_Fit Parameters:Guess Parameters Options", "Fluorescence Decay_Styles:Show Last Decay Only", "Fluorescence Decay_Styles:Decay Graph Color Array", "Fluorescence Decay:Decay Graph Active", "Fluorescence Decay Statistics:Min Peak Value", "Fluorescence Decay Statistics:Reject Low Decay Peak Pixels", "Fluorescence Decay Statistics:Reject High Decay Peak Pixels", "Fluorescence Decay Statistics:Max Peak Value", "Time Traces:Use File Timestamp", "Time Traces:Time Step", "Time Traces:Use Intensity Correction File", "Time Traces:Intensity Correction File", "Phasor Plot:Phasor Plot Smoothing Options", "Phasor Plot:Phasor Plot Size", "Phasor Plot:Phasor Plot Graphics Options", "Phasor Plot:Cumulative Phasor Plot", "Phasor Plot:Use Phasor Brightness", "Phasor Plot:Blend Overlay with Phasor Background", "Phasor Plot:Save Phasor Plot", "Phasor Plot:Show References", "Phasor Plot:Phasor Ratio Decay Range", "Phasor Plot:Exponential Fading", "Phasor Plot:Phasor Ratio Reference Colors", "Phasor Plot:Reference Radius", "Phasor Plot:Show Color Map Vertices", "Phasor Plot:Phasor Plot Active", "Phasor Plot:Phasor Ratio Color Map Type", "Phasor Plot:Phasor Ratio Color Map", "Phasor Plot:Phasor Ratio Display Range", "Phasor Plot:Selected Image ROI(s)", "Phasor Plot:All Image ROIs", "Phasor Plot:Selected Phasor Plot ROI(s)", "Phasor Plot:All Phasor Plot ROIs", "Phasor Plot:Phasor Ratio Color-Coded Quantity", "Phasor Plot:Store Phasor Harmonics", "Phasor Plot:Draw Reference Segment", "Phasor Plot:User-Defined Quantity", "Phasor Graph:Phasor Frequency", "Phasor Graph:Phasor Ratio Type", "Phasor Graph:Pixel-level Phasor Computation", "Phasor Graph:Save Phasor Graph", "Phasor Graph:Phasor Graph Active", "Phasor Graph:Phasor SDV Options", "Phasor Calibration:Use Backup Calibration if needed", "Phasor Graph:Define Shortest Lifetime as", "Phasor Calibration:Backup Calibration Type", "Phasor Calibration:Calibration Type", "Phasor Calibration:Calibration Lifetime", "Phasor Calibration:Calibration Map Algorithm", "Single-Exponential Phasor Locus (SEPL):Gate Parameters", "Single-Exponential Phasor Locus (SEPL):User-defined Gate", "Single-Exponential Phasor Locus (SEPL):User-defined IRF", "Single-Exponential Phasor Locus (SEPL):Phasor Parameters", "Single-Exponential Phasor Locus (SEPL):Decay & IRF Parameters", "Single-Exponential Phasor Locus (SEPL):Display Parameters", "Lifetime Analysis:Decay Analysis Parameters", "Lifetime Analysis:Lifetime Map Active", "Plugins:Python Settings", "Miscellaneous:Verbose Mode", "Miscellaneous:Beep after Script", "Miscellaneous:Saved Image File Format", "Miscellaneous:Exported Gate Image Settings", "Miscellaneous:Include Loading in Timing", "Miscellaneous:Verbose Settings Mode", "Miscellaneous:Histogram Options", "Miscellaneous:Beep on Error", "Miscellaneous:# Logical Processors Used", "Miscellaneous:ROI Description Max Characters", "Miscellaneous:Verbose Error Mode", "Miscellaneous:Transparent Mask Color"}
  T74 = typedef "AlliGator Globals, Variables & Constants.lvlib/AlliGator Refnums List.ctl" = enum16{"---------- AlliGator Controls ----------", "AlliGator Tab Control Refnum", "---------- AlliGator Indicators ----------", "Source Image Display Refnum", "Phasor Plot Display Refnum", "Decay Fit Parameter Map Refnum", "---------- AlliGator VIs ----------", "AlliGator Settings Refnum", "AlliGator Launcher Refnum"}
  T75 = enum32{"Invalid", "Standard", "Closed", "Hidden", "Minimized", "Maximized"}
  T76 = typedef "AlliGator Settings.lvlib/AlliGator Settings Q Action.ctl" = enum16{"Idle", "Initialization", "End Initialization", "Refresh All Parameters", "Show Window", "Cumulative Phasor Plot Checkbox", "Shift Decay Checkbox", "Use Cursor (Extrapolate) Checkbox", "Use Periodicity (Extrapolate) Checkbox", "Baseline Subtraction Method", "Extrapolate Decay Checkbox", "Use Fixed ROI Diameter Checkbox", "Use File Timestamp Checkbox", "Use Calibration Phasor Curve Checkbox (deprecated)", "Use Single Phasor Calibration Checkbox (deprecated)", "Use Calibration Phasor Map Checkbox (deprecated)", "Smooth Decay Checkbox", "Phasor Ratio Color Map Type Radio Button", "Set Phasor Ratio Color Map", "Update SEPL Parameters", "Update SEPL Plot", "Define IRF Time Constants", "Set SEPL Parameters to Dataset Ones", "Define Gates to Use", "Fit Options Changed", "Phasor Ratio Color-Coded Quantity Changed", "Update Natural Frequency", "Channel Name Changed", "Send Parameters JSON Strings to Clipboard", "Load Hot Pixel Mask Image", "Quit"}
  T77 = typedef "AlliGator Settings.lvlib/AlliGator Settings Q Element.ctl" = cluster{"Action":T76, "Data":variant}
  T78 = typedef "AlliGator Globals, Variables & Constants.lvlib/AlliGator Variables List.ctl" = enum16{"---- GUI ----", "Initialization Status", "State Indicators Refnum", "Original AlliGator Menu Items", "Current Action Loop State", "Script in progress", "Playback", "Loop Playback", "Search ROI Used", "Search ROI", "Decay Graph Max Legend Size", "Intensity Graph Max Legend Size", "Decay Statistics Graph Max Legend Size", "Phasor Graph Max Legend Size", "Phasor Ratio Graph Max Legend Size", "Lifetime Graph Max Legend Size", "---- Files ----", "Export Dataset Frames as Individual Files", "Show Batch Export Help Balloons", "Frames in Dataset", "ptu File Frame Start Indices", "Current Frame in Dataset", "Current Frame Timestamp", "------ Python Plugins ------", "Python Plugins Information", "Python Session", "Valid Python Session?", "---- Source Image ----", "Dataset Loaded", "Dataset Metadata", "Dataset Channel", "Dataset Data Description", "Background Dataset Metadata", "Background Dataset Channel", "Background Dataset Data Description", "Background File Subtraction", "Background File Path", "Background File Pile-up Correction", "Background File Pixel Well Capacity", "Background File Scaling Factor", "Source Image ROIs", "Current Source Image ROI", "Source Image ROI Event Refnum", "X_Source Image Display Range", "X_Source Image Palette Information", "Source Image Palette List", "Source Image Scale", "Current Dataset Load Settings", "Source Image:ROI Overlay Color", "---- Image Profile Window ----", "Image Profile:Overlay ROI in Source Image", "Image Profile Window Event Refnum", "Image Profile:IntensityType", "Image Profile:Intensity Average Type", "Image Profile:Intensity-weighted SDV", "Image Profile:Box Profile Type", "Image Profile Window Open", "Image Profile:Plotted Fit Parameter", "X_Type of Displayed Image", "X_Time Gate Slider", "Dataset Path", "Source Image Overlay to Erase", "Is Displayed Image Accumulated", "White Light Image Modified", "Mask Image Modified", "Macrotime Gate Separation", "------ Phasor Graph -------", "Phasor Graph:Show Line", "---- Phasor Plot ---", "Phasor Plot Parameters Changed", "FLI Dataset Modified since last Phasor Plot Calculation", "Phasor Harmonics Data", "Selected Phasor Harmonics", "Phasor Harmonic Manager Event Refnum", "Phasor Plot ROIs", "Current Phasor Plot ROI", "Phasor Plot ROI Event Refnum", "Phasor Plot Image Reference Points", "Phasor Plot Computed", "Phasor Plot Palette Information", "Phasor Plot Palette List", "Phasor Ratio Palette Information", "Phasor Ratio Palette List", "Phasor Image Scale", "Phasor Plot Image Overlay to Erase", "Phasor Plot Image Elements to Update", "Current Phasor Plot Calculation Parameters", "Current Phasor Calibration Options", "Reset Cumulated Phasor Plot", "Phasor Ratio Reference 1", "Phasor Ratio Lifetime Reference 1", "Phasor Ratio Reference 1 Frequency", "Phasor Ratio Reference 2", "Phasor Ratio Lifetime Reference 2", "Phasor Ratio Reference 2 Frequency", "---- Decay Analysis ----", "Number of Selected Decays to Fit", "LS Fit Results", "LAR Fit Results", "BS Fit Results", "Last Decay Max - Min", "Best Fit Parameters", "Best Fit Parameter Names", "Actual Size X", "Actual Size Y", "Binning X", "Binning Y", "Actual # Gates", "Dataset Number", "Gates to...", "Gates Skipped", "Gates to keep", "Gate Step", "Gate Separation", "Reversed Gates", "Pile-up Correction", "Pixel Well Capacity", "Background Subtracted", "Background Subtraction Method", "Background Definition Range", "Background File (deprecated)", "Number of Dataset Accumulated", "Array of Accumulated Dataset Paths", "Do Averaged Datasets", "Destination File Path", "Process Plot Target", "Use 1/D as Phasor Frequency", "---- Decay Fit Parameter Map -----", "Decay Fit Parameter Map Palette Information", "Decay Fit Parameter Map Palette List", "Local Decay Graph Window Event Refnum", "------- Local Decay Window ---------", "Use normalized IRF for convolution", "----- Miscellaneous ----", "Skippable Dialog Windows Status"}
  T79 = typedef "Image.lvlib/Image Hot Pixel Map Target.ctl" = enum16{"U8", "U16", "SGL"}
  T80 = typedef "AlliGator Action Engine.lvlib/AlliGator Q Element.ctl" = cluster{"AlliGator Q Event":T81, "Data":variant}
  T81 = typedef "AlliGator Action Engine.lvlib/AlliGator Q Event.ctl" = enum16{"---- Files ----", "Files:Set Batch Export Files To Save", "Files:Set Dataset Loading & Pre-processing Options", "Files:Check #Frames in Dataset", "Files:Increment Frame Index", "Files:Open Mask Image", "Files:Open White Light Image", "Files:Open Single Dataset", "Files:New Folder of Folders Selected", "Files:Load File (all Types)_Scriptable", "Files:Move Flattened Series to Folders Series", "Files:Select Folder", "Files:Load FLI Dataset", "Files:Load Swiss SPAD 1 Dataset", "Files:Load Swiss SPAD 2 Dataset", "Files:Load .sdt FLI Dataset", "Files:Load .ptu FLI Dataset", "Files:Load .bin FLI Dataset", "Files:Load Single Gate Image Folder", "Files:Load I/m/phi Dataset (deprecated)", "Files:Load Single Image", "Files:Subtract Background File", "Files:Export FLI Dataset", "Files:Load HDF5 FLI Dataset", "Files:Set Destination File Path", "Files:Save Mask Image", "Files:Batch Conversion", "Files:New Folder Selected", "Files:Close FLI Dataset", "Files:Close FLI Dataset Series", "Files:Close White Light Image", "Files:Close Mask Image", "---- FLI Dataset ----", "FLI Dataset:Channel Arithmetic", "FLI Dataset:Export Average Lifetime Map as ASCII", "FLI Dataset:Export User-Defined Quantity Map as ASCII", "FLI Dataset:Python Function FLI Dataset Event", "FLI Dataset:ROI Analysis", "FLI Dataset:Tilted Logistic Square Gated IRF Characteristics Map", "FLI Dataset:Logistic Square Gated IRF Characteristics Map", "FLI Dataset:Square Gated IRF Characteristics Map", "FLI Dataset:Multi-ROI Single-Pixel Phasor Analysis", "FLI Dataset:Multi-ROI Single-Pixel NLSF Analysis", "FLI Dataset:All ROIs IRF Extraction", "FLI Dataset:All ROIs Decay Fit Non-Interactive (Fast + Individual IRF)", "FLI Dataset:All ROIs Phasor Analysis", "FLI Dataset:All ROIs Decay Fit", "FLI Dataset:Fluorescence Decay Statistics", "FLI Dataset:Update Decay Statistics Graph", "FLI Dataset:Get Decay from ROI", "FLI Dataset:All ROIs Average Lifetimes", "---- FLI Dataset Series ----", "FLI Dataset Series:Sum All Datasets in Series", "FLI Dataset Series:Add Dataset to Accumulated Dataset", "FLI Dataset Series:Display Accumulated Dataset", "FLI Dataset Series:Clear Dataset Series Sum", "FLI Dataset Series:Time-Series Analysis (NLSF)", "FLI Dataset Series:Time-Series Analysis (Phasor)", "---- Image ----", "Image:Update Image Profile Plots", "Image:Image Histogram Cursor Move", "Image:Image Histogram", "Image:Image Contrast", "Image:Set Image Histogram Cursor Move Flag", "Image:Clear Image Overlay", "Image:Use ROI as Search Area", "Image:Set ROI Diameter", "Image:Save Image Data as TIFF", "Image:Save Displayed Image with Overlay", "Image:Save Image Overlay Only", "Image:Save Image as Hot Pixel Mask", "Image:Change Source Image Color Palette", "Image:Copy Image to Clipboard", "Image:Source Image ROI Selection", "Image:Delete All ROIs", "Image:Delete All Unselected ROIs", "Image:Delete ROI", "Image:Merge All ROIs", "Image:Store ROI", "Image:Source Image ROI Storage", "Image:Export ROI Description to Notebook", "Image:Save ROI", "Image:Load ROI", "Image:Paste ROI Definition", "Image:Clear ROI", "Image:Identify ROIs in Mask Image", "Image:Create Complementary ROI", "Image:Create Contour ROI", "Image:Create ROI(s) from Pixels with Peak above Min_Scriptable", "Image:Create ROI(s) from Pixels with Intensity above Min_Scriptable", "Image:Compute ROI Statistics", "Image:Delete ROI(s) based on ROI Characteristics", "Image:Create ROI Grid", "Image:ROI to Individual Pixel ROIs", "Image:Python Function Source Image Event", "Image:Show Phasor Calibration Map ROI Centers", "Image:Convert ROI to Mask Image", "Image:Mouse Move", "Image:Mouse Up", "Image:Set Source Image Mouse Move Flag", "Image:Add Scale Bar Overlay", "Image:Delete Existing ROIs Option", "---- Decay ----", "Decay:Clear IRF/Reference Plot", "Decay:Clear Local IRFs", "Decay:Add Decay to Graph", "Decay:Smoothen Plot", "Decay:Smoothen Plot Tail", "Decay:Average Selected Plots", "Decay:Extract IRF", "Decay:Optimal IRF Extraction", "Decay:Threshold IRF", "Decay:Fit to Model IRF", "Decay:Fit IRF to Square Gate", "Decay:Fit IRF to Logistic Square Gate", "Decay:Fit IRF to Tilted Logistic Square Gate", "Decay:Create Bounding Cursors Set", "Decay:Export Bounding Cursors Definition to Notebook", "Decay:Denoise Plot", "Decay:Compute Cumulative Function", "Decay:Use as Reference Decay", "Decay:Show Reference Decay/IRF", "Decay:Extrapolate Decay", "Decay:Create Head & Tail Bounding Cursors", "Decay:Store Cursor-defined Head & Tail Fractions", "Decay:Rebin Plot", "Decay:1-Normalize Decay", "Decay:[0-1]-Normalize Plot", "Decay:Straighten Decay", "Decay:Shift Decay", "Decay:Fold Decay", "Decay:Fit Decay", "Decay:Global Fit of Selected Decays", "Decay:Post Global Fit Script", "Decay:Add Global Fit Parameters to Graph", "Decay:Add Decay Parameter(s) to Plot (Graph)", "Decay:Export Decay to Phasor Graph", "Decay:Plot Decay Shifts", "Decay:Compute Average Lifetime", "Decay:Plot Convolution", "Decay:Graph Tip Strip Update", "---- Decay Statistics ----", "Decay Statistics:Tip Strip Update", "---- Intensity Time Trace ----", "Intensity Time Trace:Use File Timestamp", "Intensity Time Trace:Load Intensity Corrections File", "Intensity Time Trace:Clear Intensity Corrections File", "Intensity Time Trace:Tip Strip Update", "---- Phasor Plot ----", "Phasor Plot:Build Phasor Plot", "Phasor Plot:Change Phasor Plot Color Palette", "Phasor Plot:Adjust Phasor Plot Display Range", "Phasor Plot:Highlight Image ROI in Phasor Plot", "Phasor Plot:Save Phasor Plot Image with Overlay", "Phasor Plot:Export Complex Phasor Map", "Phasor Plot:Export Phasor Ratio Map", "Phasor Plot:Export Average Lifetime Map", "Phasor Plot:Compute Phase Lifetime Histogram", "Phasor Plot:Compute Phasor Ratio Histogram", "Phasor Plot:Compute Phase Lifetime vs Intensity Scatter Plot", "Phasor Plot:Weber 2-Component Decomposition", "Phasor Plot:Update Phasor Color Map Vertices", "Phasor Plot:Clear Phasor Overlay", "Phasor Plot:Use Segment Extremities as References", "Phasor Plot:Use UC/Segment Intersections as References", "Phasor Plot:Use UC/Principal Axis Intersections as References", "Phasor Plot:Use UC/Linear Fit Intersections as References", "Phasor Plot:Update Phasor Plot Reference", "Phasor Plot:Show Local Phasor Info in Phasor Plot", "Phasor Plot:Update Phasor Plot State", "Phasor Plot:Phasor Plot ROI Storage", "Phasor Plot:Phasor Plot ROI Selection", "Phasor Plot:Python Function Phasor Plot Event", "Phasor Plot:Overlay Phasor ROI, Ratio or Map in Source Image", "Phasor Plot:Compute Decay of Selected Phasors", "Phasor Plot:Phasor at Image Pixel", "Phasor Plot:Mouse Move", "Phasor Plot:Mouse Up", "Phasor Plot:Display Range Mouse Move", "Phasor Plot:Set Mouse Move Flag", "---- Phasor Graph ----", "Phasor Graph:Calibrated Phasor Map Series", "Phasor Graph:Whole Image Phasor Scatter Plot (Todo)", "Phasor Graph:Get Phasor Value", "Phasor Graph:Create New Phasor Plot Dialog", "Phasor Graph:Update Last Phasor Value", "Phasor Graph:Update Phasor (m, phi)", "Phasor Graph:Remove Single Phasor from Plot", "Phasor Graph:Add Single Phasor to Plot", "Phasor Graph:Remove Phasor Plot", "Phasor Graph:Remove Selected Phasor Plots", "Phasor Graph:Clear Phasor Data", "Phasor Graph:Clear Phasor Graph", "Phasor Graph:Cursor Move", "Phasor Graph:Draw Cursor Connecting Line", "Phasor Graph:Clear Cursor Connecting Line", "Phasor Graph:Find UC Intersection", "Phasor Graph:Use UC/Cursor-Defined Line Intersections", "Phasor Graph:Use Selected Plots Fitted Line/UC Intersections", "Phasor Graph:Use Selected Plots Principal Axis/UC Intersections", "Phasor Graph:Show Single Phasor", "Phasor Graph:Save Single Phasor Plot", "Phasor Graph:Save All Phasor Plots", "Phasor Graph:Load Phasor Plot(s)", "Phasor Graph:Phasor Multiplication", "Phasor Graph:Compute Average Phasor", "Phasor Graph:Compute Multiple Average Phasors (Selected Plots)", "Phasor Graph:Export Single Phasor Plot Phase Lifetimes", "Phasor Graph:Phase Lifetime Trajectory", "Phasor Graph:Phase Lifetime vs Intensity Scatter Plot (deprecated)", "Phasor Graph:Parameter 2 vs Parameter 1 Scatter Plot", "Phasor Graph:Use Cursor n Location", "Phasor Graph:Set Reference n to Current Phase Lifetime Value", "Phasor Graph:Set Reference n to Lifetime Value", "Phasor Graph:Set Cursor n Location", "Phasor Graph:Save Phasor Graph Image", "Phasor Graph:Update SEPL Plot", "Phasor Graph:Export Single Phasor Plot Data", "Phasor Graph:Export Selected Phasor Plots Data", "Phasor Graph:Python Function Phasor Graph Event", "Phasor Graph:Tip Strip Update", "---- Calibration ----", "Calibration:Set Calibration Type", "Calibration:Load/Save Phasor Calibration", "Calibration:Load/Save Phasor Calibration Series", "Calibration:Load/Save Phasor Calibration Map", "Calibration:Use as Calibration", "Calibration:Compute Optimal Calibration from Phasor References", "Calibration:Clear Phasor Calibration", "Calibration:Single Phasor Calibration Information", "Calibration:Use as Calibration Series", "Calibration:Use as Calibration Map", "Calibration:Clear Calibration Series", "Calibration:Phasor Calibration Series Information", "Calibration:Clear Calibration Map", "Calibration:Phasor Calibration Map Information", "Calibration:Apply Phasor Calibration", "Calibration:Update Single Plot Calibration", "Calibration:Update Multiple Plots Calibration", "Calibration:Clear Single Plot Calibration", "Calibration:Clear All Plots Calibrations", "Calibration:Clear Plot(s) Calibration(s)?", "Calibration:Phasor Calibration Maps (# Gates Series)", "---- Phasor Ratio ----", "Phasor Ratio:Clear Reference n", "Phasor Ratio:Toggle Selected Plot(s)  Lock to Reference 1", "Phasor Ratio:Use as Reference n", "Phasor Ratio:Send Reference n to Notebook", "Phasor Ratio:Toggle Selected Plot(s)  Lock to Reference 2", "Phasor Ratio:Compute Phasor Ratio at Mouse Location", "Phasor Ratio:Compute Phasor Plot's Average Phasor Ratio", "Phasor Ratio:Compute Time-Series Phasor Ratios", "Phasor Ratio:Fit Line to Phasor Ratio Plot", "Phasor Ratio:Save References", "Phasor Ratio:Load References", "Phasor Ratio:Update Phasor Reference 1", "Phasor Ratio:Update Phasor Reference 2", "Phasor Ratio:Move Cursor n to Reference n", "Phasor Ratio:Use as Phasor Reference 1 Lifetime", "Phasor Ratio:Use as Phasor Reference 2 Lifetime", "Phasor Ratio:Export Phasor Ratio Map as ASCII", "Phasor Ratio:Tip Strip Update", "---- Lifetime & Other Parameters Graph ----", "Lifetime:Tip Strip Update", "---- Decay Fit Parameter Map ----", "Decay Fit Parameter Map:Export ROI NLSF Data as ASCII", "Decay Fit Parameter Map:Set Decay Fit  Parameter Map Selection", "Decay Fit Parameter Map:Build Decay Fit Parameter Map", "Decay Fit Parameter Map:Change Decay Fit Parameter Map Color Palette", "Decay Fit Parameter Map:Export Decay Fit Parameter Map Data as ASCII", "Decay Fit Parameter Map:Export All Decay Fit Parameter Maps Data as ASCII", "Decay Fit Parameter Map:Send Map Data to Lifetime Graph", "Decay Fit Parameter Map:Save Decay Fit Parameter Map Image", "Decay Fit Parameter Map:Save-Load IRFs & Fit Data", "Decay Fit Parameter Map:Update Local Decay Plots", "Decay Fit Parameter Map:Python Function Decay Fit Parameters Map Event", "Decay Fit Parameter Map:Overlay Decay Fit Parameter Map in Source Image", "Decay Fit Parameter Map:Plot Map Data vs Intensity", "Decay Fit Parameter Map:Mouse Up", "Decay Fit Parameter Map:Display Range Mouse Move", "---- Generic Graph ----", "Generic Graph:Generic XY Graph Event", "Generic Graph:Python Function XY Graph Event", "Generic Graph:New Plot", "Generic Graph:Save Plot", "Generic Graph:XY Plot Histogram", "Generic Graph:Set XY Graph Plot Name", "Generic Graph:Set Last Cursor Style", "Generic Graph:Tip Strip Update", "---- GUI ----", "GUI:Start Script", "GUI:Type of Displayed Image Changed", "GUI:Gate Image Slide Changed", "GUI:Show Busy Icon", "GUI:Show Busy Icon & Abort Button", "GUI:Hide Busy Icon", "GUI:Hide Busy Icon & Abort Button", "GUI:Abort", "GUI:End Script", "GUI:Start Timing", "GUI:End Timing", "GUI:Set State Indicator", "GUI:Send Parameters JSON Strings to Clipboard", "GUI:Set Gate Step", "GUI:Idle", "GUI:Initialization", "GUI:Quit", "GUI:Increment Dataset Index", "GUI:Set Dataset Index to -1", "GUI:Time Series Slider Moved", "GUI:Time Series Slider Changed", "GUI:Toggle Playback or Loop", "GUI:Playback Script", "GUI:Set Phasor Frequency", "GUI:Open Window", "GUI:Start Test Script", "GUI:End Test Script", "DEBUG"}
  T82 = typedef "Palette.lvlib/Image Palette Information.ctl" = cluster{"Palette Name [# Colors,int?,inv?]":string, "Palette Type":T83, "Palette Colors":u32[], "Interpolate?":bool}
  T83 = typedef "Image.lvlib/Image Display Palette Type.ctl" = u32
  T84 = typedef "Palette.lvlib/Interpolated Color Scale Definition.ctl" = cluster{"Color Scale Points":cluster{"Value":dbl, "Color":u32}[], "Color Scale Name":string}
  T85 = typedef "Notebook.lvlib/Notebook Parameters List.ctl" = enum16{"First Opening?", "Saved Notebook?", "Saved Notebook Path", "Beep on Error?"}
  T86 = typedef "AlliGator GUI.lvlib/AlliGator Skippable Windows Status.ctl" = cluster{"Dialog Window Name":string, "Is skipped":bool}
  T87 = typedef "AlliGator Settings.lvlib/AlliGator Quantities.ctl" = string[]
  T88 = typedef "XY Graph Add-Ons.lvlib/XY Plot Data.ctl" = cluster{"X Array":dbl[], "Y Array":dbl[]}
  T89 = typedef "AlliGator Settings Window Messages.ctl" = enum16{"Idle", "Subscribe", "Unsubscribe", "Refresh Parameter", "Refresh All Parameters", "Quit"}
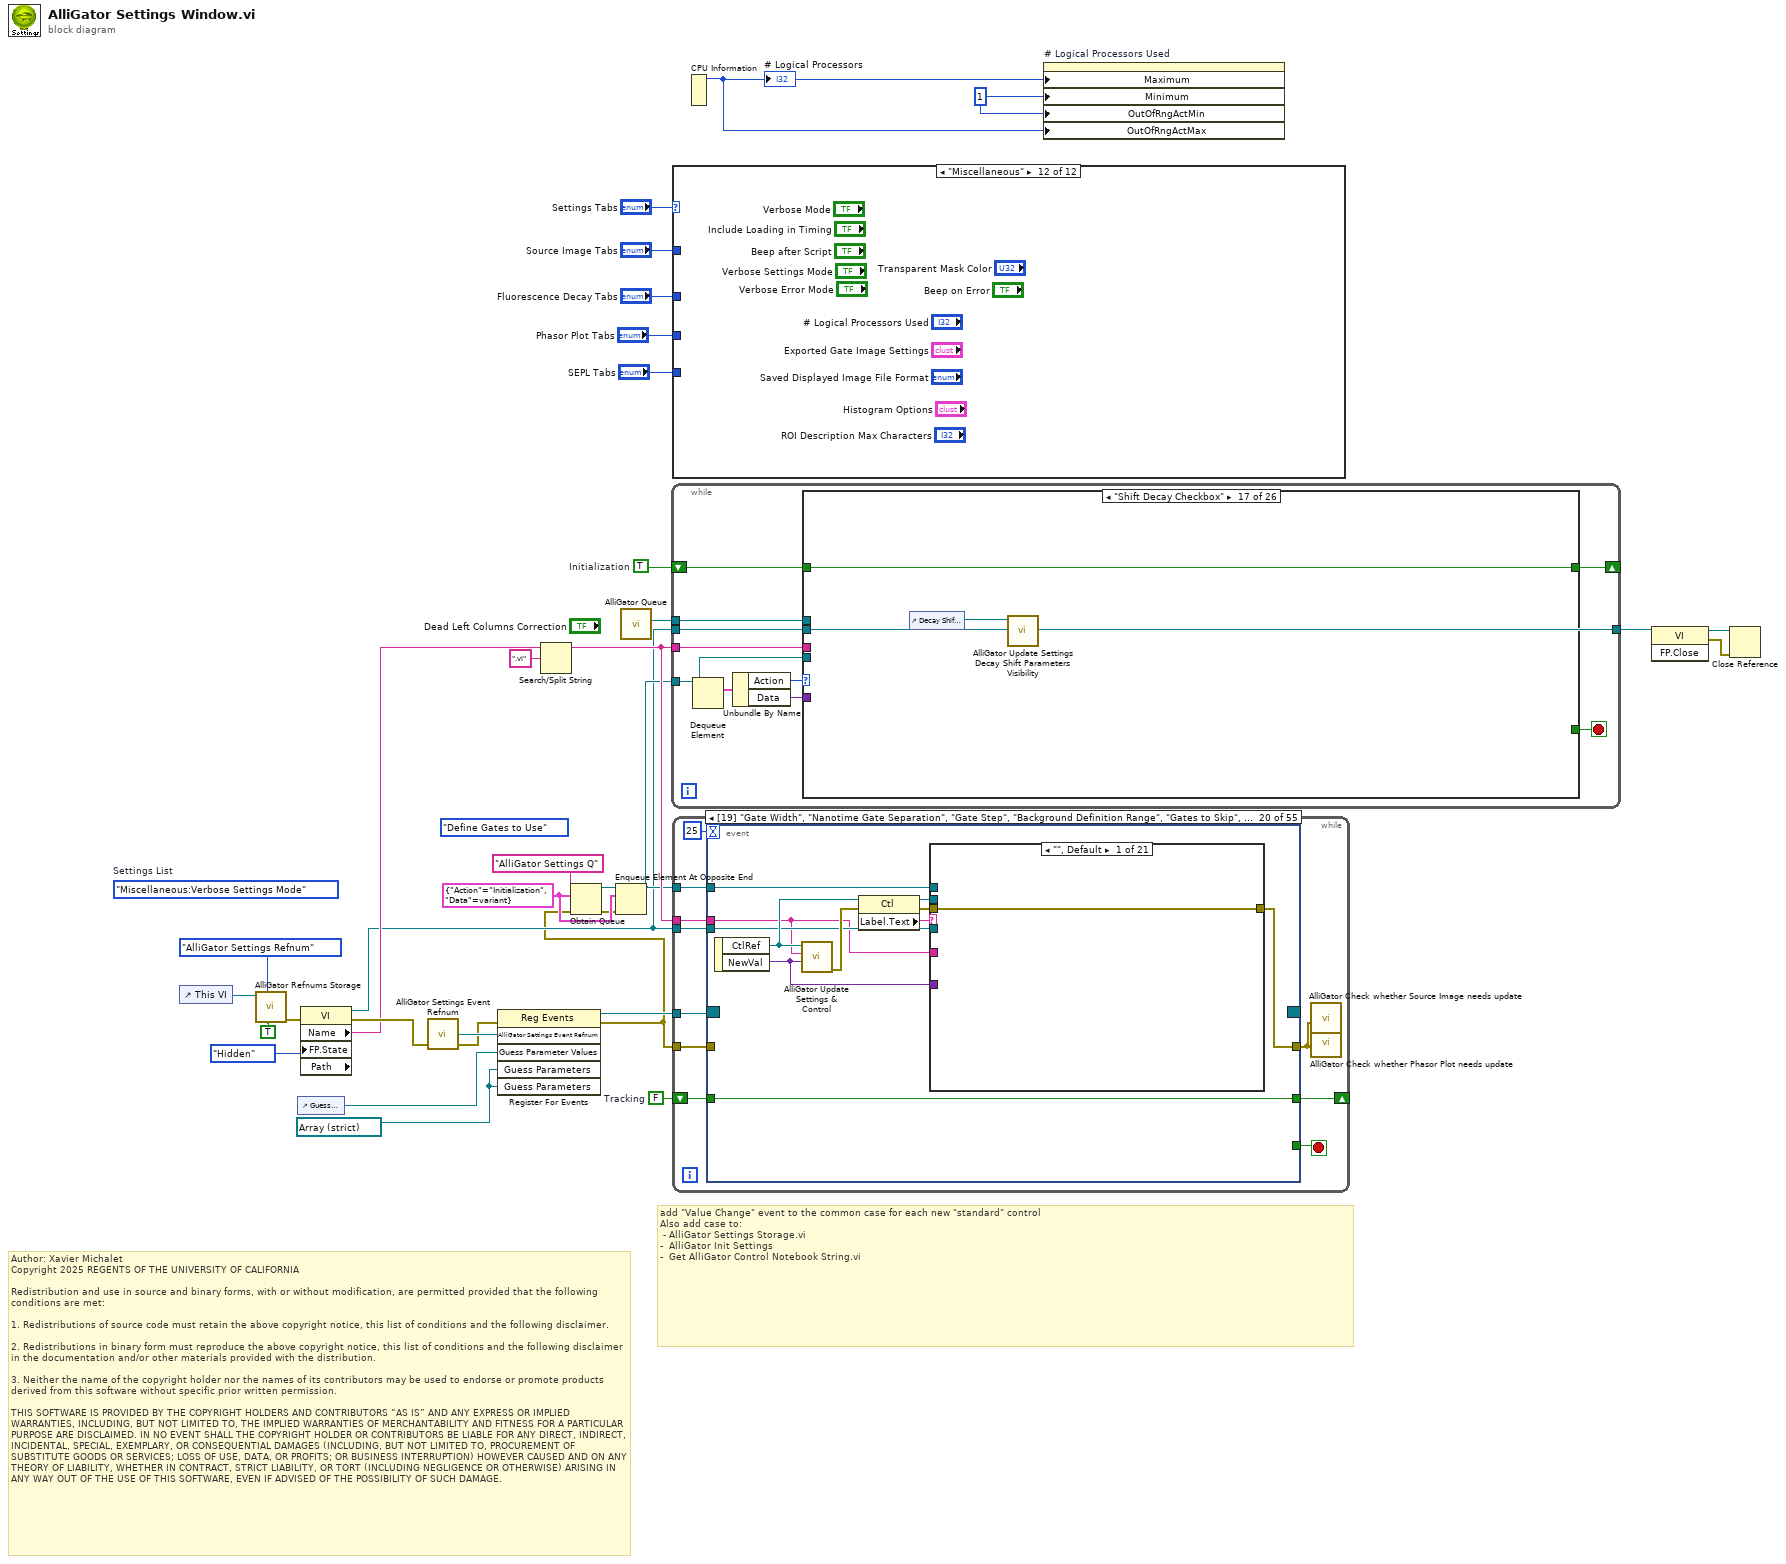
[diagram p0: block diagram]
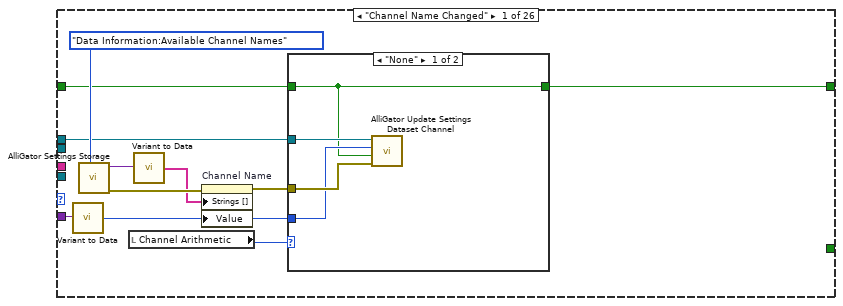
[diagram p2: hidden frame]
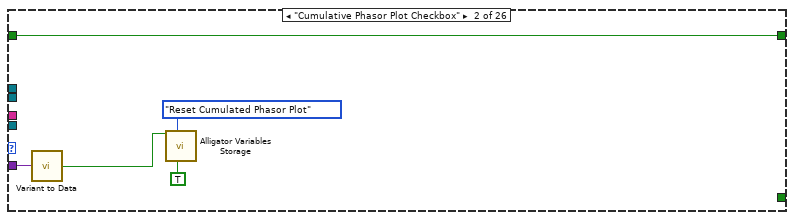
[diagram p4: hidden frame]
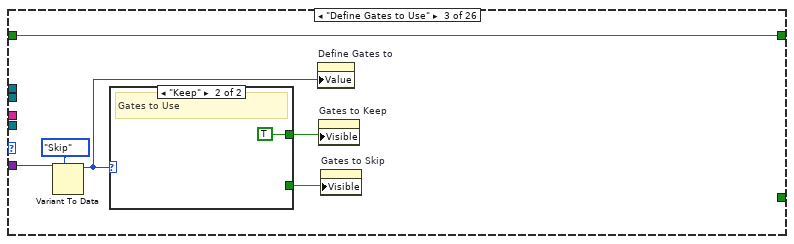
[diagram p5: hidden frame]
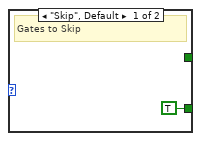
[diagram p6: hidden frame]
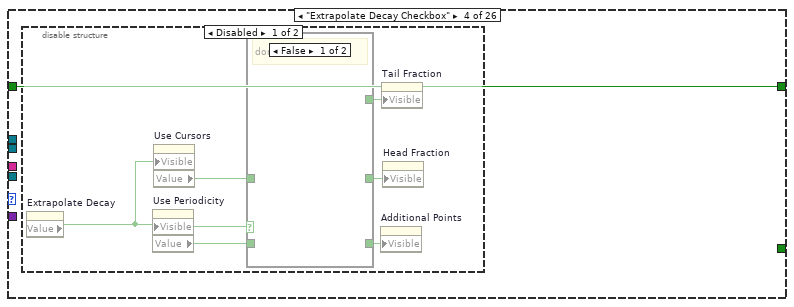
[diagram p7: hidden frame]
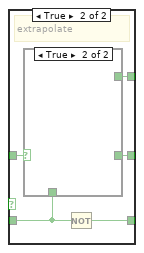
[diagram p8: hidden frame]
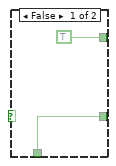
[diagram p9: hidden frame]
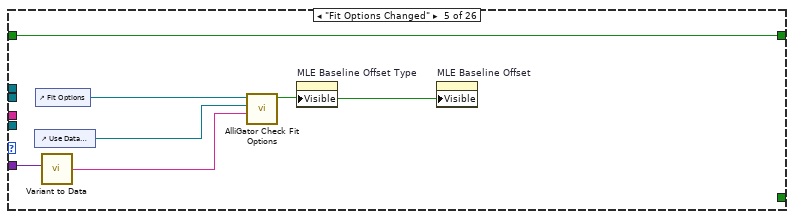
[diagram p11: hidden frame]
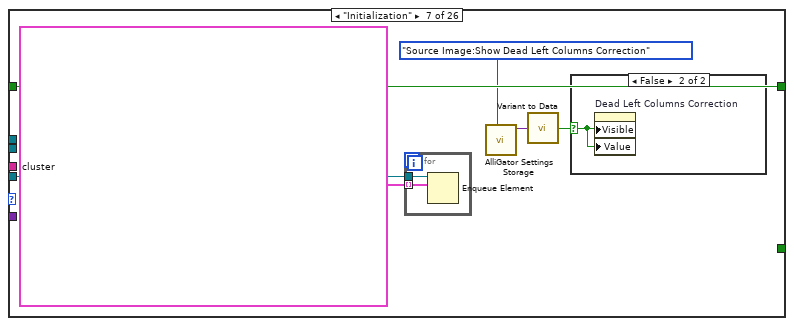
[diagram p13: hidden frame]
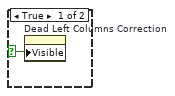
[diagram p14: hidden frame]
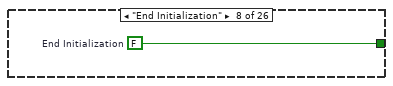
[diagram p15: hidden frame]
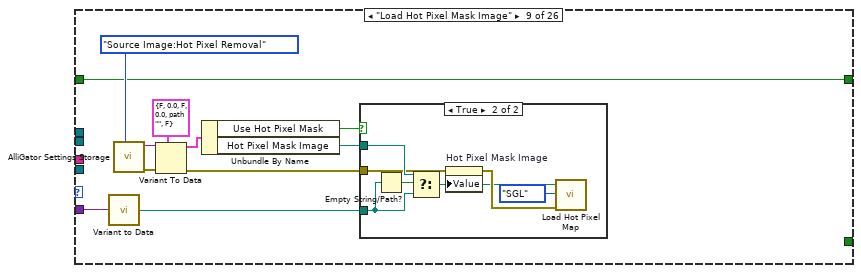
[diagram p16: hidden frame]
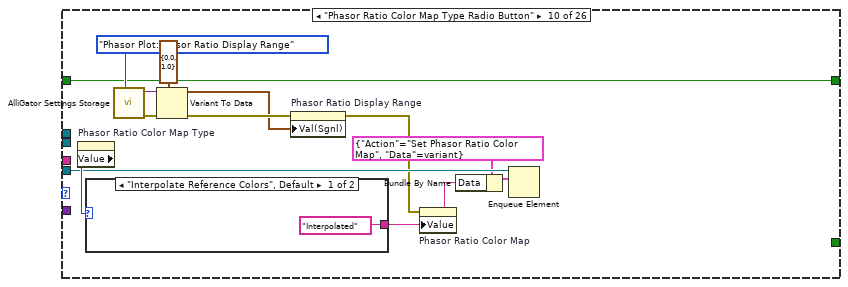
[diagram p18: hidden frame]
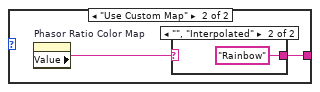
[diagram p19: hidden frame]
diagram:
  w3 = TRUE  # Initialization
  (unwired) AlliGator_Settings_List."Miscellaneous:Verbose Settings Mode"  # Settings List
  w9 = 1 ("Data Entry Limits:Minimum")
  (unwired) AlliGator_Settings_Q_Action."Define Gates to Use" ("Action")
  w16 = T77 {"Action"=enum."Initialization", "Data"=variant} ("AlliGator Settings Q Element")
  w24 = FALSE  # Tracking
  w25 = refnum<vi> refnum ("Guess Parameters")
  # "Author: Xavier Michalet\nCopyright 2025 REGENTS OF THE UNIVERSITY OF CALIFORNIA\n\nRedistribution and use in source and binary forms, with or without modification, are permitted provided that the following conditions are met:\n\n1. Redistributions of source code must retain the above copyright notice, this list of conditions and the following disclaimer.\n\n2. Redistributions in binary form must reproduce the above copyright notice, this list of conditions and the following disclaimer in the documentation and/or other materials provided with the distribution.\n\n3. Neither the name of the copyright holder nor the names of its contributors may be used to endorse or promote products derived from this software without specific prior written permission.\n\nTHIS SOFTWARE IS PROVIDED BY THE COPYRIGHT HOLDERS AND CONTRIBUTORS “AS IS” AND ANY EXPRESS OR IMPLIED WARRANTIES, INCLUDING, BUT NOT LIMITED TO, THE IMPLIED WARRANTIES OF MERCHANTABILITY AND FITNESS FOR A PARTICULAR PURPOSE ARE DISCLAIMED. IN NO EVENT SHALL THE COPYRIGHT HOLDER OR CONTRIBUTORS BE LIABLE FOR ANY DIRECT, INDIRECT, INCIDENTAL, SPECIAL, EXEMPLARY, OR CONSEQUENTIAL DAMAGES (INCLUDING, BUT NOT LIMITED TO, PROCUREMENT OF SUBSTITUTE GOODS OR SERVICES; LOSS OF USE, DATA, OR PROFITS; OR BUSINESS INTERRUPTION) HOWEVER CAUSED AND ON ANY THEORY OF LIABILITY, WHETHER IN CONTRACT, STRICT LIABILITY, OR TORT (INCLUDING NEGLIGENCE OR OTHERWISE) ARISING IN ANY WAY OUT OF THE USE OF THIS SOFTWARE, EVEN IF ADVISED OF THE POSSIBILITY OF SUCH DAMAGE."
  # "add \"Value Change\" event to the common case for each new \"standard\" control\nAlso add case to:\n - AlliGator Settings Storage.vi\n-  AlliGator Init Settings\n-  Get AlliGator Control Notebook String.vi"
  n1 = control-ref of="This VI"() -> (w7:refnum<vi>)
  n2 = call "AlliGator Refnums Storage.vi"("Get(F)/Set"=TRUE, "AlliGator Refnum List"=AlliGator_Refnums_List."AlliGator Settings Refnum", "Data in"=w7) -> ("Error Out"=w6:errorcluster)  [unwired: 7 in, 1 out]
  n3 = control-ref of="Guess Parameter Values"() -> (w26:refnum<vi>)
  n4 = property class="VI" props=["Name", "FP.State", "Path"](error in=w6, "FP.State"=T75."Hidden" ("Front Panel Window:State")) -> (reference out=w14:refnum<vi>, error out=w31:errorcluster, "Name"=w30:string)  [unwired: 1 in, 1 out]
  n5 = call "AlliGator Settings Event Refnum.vi"("Error In"=w31) -> ("AlliGator Settings Event Refnum"=w34:refnum<user-event>, "Error Out"=w33:errorcluster)  [unwired: 7 in]
  n6 = register-events(error in=w33, w34, w26, w25, w25) -> (reference out=w32:refnum<event-registration>, error out=w13:errorcluster)  [unwired: 1 in]
  n7 = Search/Split String(string=w30, search string/char (-)=".vi") -> (substring before match=w19:string)  [unwired: 1 in, 2 out]
  n8 = Obtain Queue(name (unnamed)="AlliGator Settings Q", element data type=w16, error in (no error)=w13) -> (queue out=w20:refnum<queue>, error out=w15:errorcluster)  [unwired: 2 in, 1 out]
  n9 = Enqueue Element At Opposite End(queue=w20, element=w16, error in (no error)=w15) -> (queue out=w17:refnum<queue>)  [unwired: 1 in, 2 out]
  n10 = call "AlliGator Queue.vi"() -> ("AlliGator Q"=w18:refnum<queue>)  [unwired: 8 in, 1 out]
  n11 = while {
    tunnel: w17 -> [w39]
    tunnel: w19 -> [w40]
    tunnel: w18 -> [w38]
    tunnel: w14 -> [w37]
    tunnel: [w37] -> w11
    shift-right: [w35] -> _
    shift-left: w3 -> [w36]
    stop <- w42 stop-if-true
    n12 = Dequeue Element(queue=w39) -> (element=w44:T77)  [unwired: 2 in, 3 out]
    n13 = Unbundle By Name(w44) -> ("Action"=w43:T76, "Data"=w41:variant)
    n14 = case shown="\"Shift Decay Checkbox\"" w43 {
      tunnel: [_ _ _ _ _ _ _ _ _ _ _ TRUE _ _ _ _ _ _ _ _ _ _ _ _ _ _] -> w42
      tunnel: w41 -> [w53 w65 w71 _ w92 _ _ _ w116 _ w158 _ _ _ w206 _ _ _ _ _ _ _ w306 _ _ w322]
      tunnel: w40 -> [_ _ _ _ _ _ _ _ _ _ _ _ _ _ _ _ _ _ _ _ w285 _ _ _ _ _]
      tunnel: w39 -> [_ _ _ _ _ _ w100 _ _ w135 _ _ _ _ _ _ _ _ _ _ _ _ _ _ _ _]
      tunnel: w38 -> [w49 _ _ _ _ _ _ _ _ _ _ _ _ w197 _ _ _ _ _ _ _ w303 _ _ w319 _]
      tunnel: w37 -> [_ _ _ _ _ _ _ _ _ _ _ _ w191 _ _ _ _ w271 _ _ w297 _ _ _ _ _]
      tunnel: w36 -> [w46 w61 w66 w74 w88 w94 w98 _ w106 w125 w142 w183 w185 w192 w202 w258 w265 w267 w272 w274 w279 w302 w305 w317 w318 w321]
      tunnel: [w45 w61 w66 w74 w88 w94 w98 w105 w106 w125 w142 w183 w185 w192 w202 w258 w265 w267 w272 w274 w279 w302 w305 w317 w318 w321] -> w35
      frame "Channel Name Changed" {
        n15 = call-poly "Variant to Data.vi"("Variant"=w53) -> ("U16 Value"=w50:u16)  [unwired: 8 in]
        n16 = call "AlliGator Settings Storage.vi"("AlliGator Settings List"=AlliGator_Settings_List."Data Information:Available Channel Names") -> ("Error Out"=w52:errorcluster, "Variant Data out"=w55:variant)  [unwired: 9 in]
        n17 = local read "Channel Arithmetic"() -> (w51:T12)
        n18 = call-poly "Variant to Data.vi"("Variant"=w55) -> ("String Array"=w47:string[])  [unwired: 8 in]
        n19 = property on="Channel Name" class="Ring (strict)"(error in=w52, "Strings []"=w47, "Value"=w50) -> (error out=w48:errorcluster)  [unwired: 1 in, 1 out]
        n20 = case shown="\"None\"" w51 {
          tunnel: w50 -> [w57 _]
          tunnel: w49 -> [w59 _]
          tunnel: w48 -> [w58 _]
          tunnel: w46 -> [w56 w60]
          tunnel: [w56 w60] -> w45
          frame "None" {
            n21 = call "AlliGator Update Settings Dataset Channel.vi"("error in (no error)"=w58, "Initialization?"=w56, "Selected Channel"=w57, "AlliGator Queue"=w59) -> ()  [unwired: 7 in, 1 out]
          }
          frame "INT-G2", Default {
          }
        }
      }
      frame "Cumulative Phasor Plot Checkbox" {
        n22 = call-poly "Variant to Data.vi"("Variant"=w65) -> ("Value"=w64:bool)  [unwired: 8 in]
        n23 = call "Alligator Variables Storage.vi"("Get(F)/Set"=TRUE, "AlliGator Variable"=AlliGator_Variables_List."Reset Cumulated Phasor Plot" ("Alligator Variable"), "Data in"=w64) -> ()  [unwired: 6 in, 3 out]
      }
      frame "Define Gates to Use" {
        n24 = Variant To Data(type=AlliGator_Define_Gates_to."Skip" ("Define Gates to"), Variant=w71) -> (data=w67:T14)  [unwired: 1 in, 1 out]
        n25 = case shown="\"Keep\"" w67 {
          tunnel: [TRUE ("Visible") _] -> w69
          tunnel: [_ TRUE ("Visible")] -> w68
          frame "Skip", Default {
            # "Gates to Skip"
          }
          frame "Keep" {
            # "Gates to Use"
          }
        }
        n26 = property on="Define Gates to" class="RadioBtnsControl (strict)"("Value"=w67) -> ()  [unwired: 2 in, 2 out]
        n27 = property on="Gates to Keep" class="Clust (strict)"("Visible"=w68) -> ()  [unwired: 2 in, 2 out]
        n28 = property on="Gates to Skip" class="Clust (strict)"("Visible"=w69) -> ()  [unwired: 2 in, 2 out]
      }
      frame "Extrapolate Decay Checkbox" {
        n29 = disable-structure shown="Disabled" {
          frame Disabled {
            n30 = property on="Extrapolate Decay" class="Bool (strict)"() -> ("Value"=w78:bool)  [unwired: 2 in, 2 out]
            n31 = property on="Use Periodicity" class="Bool (strict)"("Visible"=w78) -> ("Value"=w80:bool)  [unwired: 2 in, 2 out]
            n32 = property on="Use Cursors" class="Bool (strict)"("Visible"=w78) -> ("Value"=w75:bool)  [unwired: 2 in, 2 out]
            n33 = case shown="False" w78 {
              tunnel: w80 -> [_ w81]
              tunnel: [_ w82] -> w79
              tunnel: w75 -> [_ w85]
              tunnel: [_ w83] -> w77
              tunnel: [_ w84] -> w76
              frame False {
                # "don't extrapolate"
              }
              frame True {
                # "extrapolate"
                n34 = case shown="True" w85 {
                  tunnel: [TRUE ("Use Cursors") _] -> w84
                  tunnel: [w86 _] -> w83
                  tunnel: w81 -> [w86 _]
                  frame False {
                  }
                  frame True {
                  }
                }
                n35 = Not(x=w81) -> (.not. x?=w82:bool)
              }
            }
            n36 = property on="Additional Points" class="DigNum (strict)"("Visible"=w79) -> ()  [unwired: 2 in, 2 out]
            n37 = property on="Tail Fraction" class="DigNum (strict)"("Visible"=w76) -> ()  [unwired: 2 in, 2 out]
            n38 = property on="Head Fraction" class="DigNum (strict)"("Visible"=w77) -> ()  [unwired: 2 in, 2 out]
          }
          frame Enabled {
          }
        }
      }
      frame "Fit Options Changed" {
        n39 = control-ref of="Use Data Information Laser Period"() -> (w91:refnum<vi>)
        n40 = control-ref of="Fit Options"() -> (w93:refnum<vi>)
        n41 = call-poly "Variant to Data.vi"("Variant"=w92) -> ("String"=w90:string)  [unwired: 8 in]
        n42 = call "AlliGator Check Fit Options.vi"("Modified Option"=w90, "Use Data Information Period Refnum"=w91, "Fit Options Refnum"=w93) -> ("MLE Options Visible?"=w89:bool)  [unwired: 7 in, 1 out]
        n43 = property on="MLE Baseline Offset Type" class="RadioBtnsControl (strict)"("Visible"=w89) -> ()  [unwired: 2 in, 2 out]
        n44 = property on="MLE Baseline Offset" class="DigNum (strict)"("Visible"=w89) -> ()  [unwired: 2 in, 2 out]
      }
      frame "Idle", Default {
      }
      frame "Initialization" {
        n45 = for {
          tunnel: w100 -> [w104]
          tunnel: T77[] [{"Action"=enum."Refresh All Parameters", "Data"=variant}, {"Action"=enum."Extrapolate Decay Checkbox", "Data"=variant}, {"Action"=enum."Phasor Ratio Color Map Type Radio Button", "Data"=variant}, {"Action"=enum."Shift Decay Checkbox", "Data"=variant}, {"Action"=enum."Use Cursor (Extrapolate) Checkbox", "Data"=variant}, {"Action"=enum."Baseline Subtraction Method", "Data"=variant}, {"Action"=enum."Show Window", "Data"=variant}, {"Action"=enum."Define Gates to Use", "Data"=variant}, {"Action"=enum."Update Natural Frequency", "Data"=variant}, {"Action"=enum."Load Hot Pixel Mask Image", "Data"=variant}, {"Action"=enum."Fit Options Changed", "Data"=variant}, {"Action"=enum."Phasor Ratio Color-Coded Quantity Changed", "Data"=variant}, {"Action"=enum."End Initialization", "Data"=variant}] ("element") -> [w103] mode=indexing
          n46 = Enqueue Element(queue=w104, element=w103) -> ()  [unwired: 2 in, 3 out]
        }
        n47 = call "AlliGator Settings Storage.vi"("AlliGator Settings List"=AlliGator_Settings_List."Source Image:Show Dead Left Columns Correction") -> ("Variant Data out"=w96:variant)  [unwired: 9 in, 1 out]
        n48 = call-poly "Variant to Data.vi"("Variant"=w96) -> ("Value"=w95:bool)  [unwired: 8 in]
        n49 = case shown="False" w95 {
          selector: w95 -> [w101 w102]
          frame True {
            n50 = property on="Dead Left Columns Correction" class="Bool (strict)"("Visible"=w101) -> ()  [unwired: 2 in, 2 out]
          }
          frame False {
            n51 = property on="Dead Left Columns Correction" class="Bool (strict)"("Visible"=w102, "Value"=w102) -> ()  [unwired: 2 in, 2 out]
          }
        }
      }
      frame "End Initialization" {
        w105 = FALSE  # End Initialization
      }
      frame "Load Hot Pixel Mask Image" {
        n52 = call-poly "Variant to Data.vi"("Variant"=w116) -> ("Path"=w115:path)  [unwired: 8 in]
        n53 = call "AlliGator Settings Storage.vi"("AlliGator Settings List"=AlliGator_Settings_List."Source Image:Hot Pixel Removal") -> ("Error Out"=w112:errorcluster, "Variant Data out"=w113:variant)  [unwired: 9 in]
        n54 = Variant To Data(error in=w112, type=T4 {"Remove Screamers"=FALSE, "Delta"=0.0, "Equalize Histogram"=FALSE, "Percentile"=0.0, "Hot Pixel Mask Image"=path "", "Use Hot Pixel Mask"=FALSE} ("Image Display Options"), Variant=w113) -> (data=w110:T4, error out=w108:errorcluster)
        n55 = Unbundle By Name(w110) -> ("Use Hot Pixel Mask"=w107:bool, "Hot Pixel Mask Image"=w109:path)
        n56 = case shown="True" w107 {
          tunnel: w115 -> [_ w123]
          tunnel: w109 -> [_ w122]
          tunnel: w108 -> [_ w120]
          frame False {
          }
          frame True {
            n57 = Empty String/Path?(string/path=w123) -> (empty?=w121:bool)
            n58 = Select(t=w122, s=w121, f=w123) -> (s? t:f=w118:path)
            n59 = property on="Hot Pixel Mask Image" class="Path"(error in=w120, "Value"=w118) -> (error out=w119:errorcluster)  [unwired: 1 in, 1 out]
            n60 = call "Load Hot Pixel Map.vi"("Error In"=w119, "Hot Pixel Map Target"=Image_Hot_Pixel_Map_Target."SGL", "Hot Pixel Mask Image Path"=w118) -> ()  [unwired: 7 in, 2 out]
          }
        }
      }
      frame "Phasor Ratio Color Map Type Radio Button" {
        n61 = property on="Phasor Ratio Color Map Type" class="RadioBtnsControl (strict)"() -> ("Value"=w136:T46)  [unwired: 2 in, 2 out]
        n62 = case shown="\"Interpolate Reference Colors\", Default" w136 {
          tunnel: ["Interpolated" w138] -> w132
          frame "Interpolate Reference Colors", Default {
          }
          frame "Use Custom Map" {
            n63 = property on="Phasor Ratio Color Map" class="Str"() -> ("Value"=w139:string)  [unwired: 2 in, 2 out]
            n64 = case shown="\"\", \"Interpolated\"" w139 {
              selector: w139 -> [w140 _]
              tunnel: [w140 "Rainbow"] -> w138
              frame Default {
              }
              frame "", "Interpolated" {
              }
            }
          }
        }
        n65 = call "AlliGator Settings Storage.vi"("AlliGator Settings List"=AlliGator_Settings_List."Phasor Plot:Phasor Ratio Display Range") -> ("Error Out"=w130:errorcluster, "Variant Data out"=w128:variant)  [unwired: 9 in]
        n66 = Variant To Data(error in=w130, type=cluster{dbl, dbl} {0.0, 1.0} ("Phasor Ratio Display Range 2"), Variant=w128) -> (data=w124:cluster{dbl, dbl}, error out=w127:errorcluster)
        n67 = property on="Phasor Ratio Display Range" class="Slide (strict)"(error in=w127, "Val(Sgnl)"=w124) -> (error out=w126:errorcluster)  [unwired: 1 in, 1 out]
        n68 = property on="Phasor Ratio Color Map" class="Str"(error in=w126, "Value"=w132) -> ()  [unwired: 1 in, 2 out]
        n69 = Bundle By Name(cluster=T77 {"Action"=enum."Set Phasor Ratio Color Map", "Data"=variant} ("element"), "Data"=w132) -> (w133:T77)
        n70 = Enqueue Element(queue=w135, element=w133) -> ()  [unwired: 2 in, 3 out]
      }
      frame "Phasor Ratio Color-Coded Quantity Changed" {
        n71 = Variant To Data(type=AlliGator_Phasor_Ratio_Color-Coded_Quantity."Phasor Ratio (f1 or a1)" ("Fit Options"), Variant=w158) -> (data=w156:T47, error out=w150:errorcluster)  [unwired: 1 in]
        n72 = control-ref of="Phasor Ratio Display Range"() -> (w149:refnum<vi>)
        n73 = case shown="\"User-Defined Quantity\"" w156 {
          tunnel: ["Phasor Ratio Color Scale" ("Caption.Text") "Average Lifetime Color Scale" ("Caption.Text") w181] -> w155
          tunnel: ["Phasor Ratio Color Map" ("Caption.Text") "Average Lifetime Color Map" ("Caption.Text") w179] -> w154
          tunnel: ["Phasor Ratio Display Range" ("Caption.Text") "Average Lifetime Display Range" ("Caption.Text") w176] -> w148
          tunnel: [0.0 ("Scale.Range:Minimum") w168 w174] -> w147
          tunnel: [1.0 ("Scale.Range:Maximum") w167 w174] -> w146
          tunnel: [w159 w166 w175] -> w145
          tunnel: w150 -> [w159 w165 w175]
          frame "Phasor Ratio (f1 or a1)", Default {
          }
          frame "Average Lifetime (<tau>_i or <tau>_a))" {
            n74 = call "AlliGator Get-Set Phasor Ratio References.vi"("error in (no error)"=w165) -> ("Reference Lifetime 1"=w170:dbl[unit], "Reference Lifetime 2"=w169:dbl[unit], "error out"=w166:errorcluster)  [unwired: 7 in, 5 out]
            n75 = node(w170) -> (w168:dbl)
            n76 = node(w169) -> (w167:dbl)
          }
          frame "User-Defined Quantity" {
            w174 = nan ("Scale.Range:Minimum")
            n77 = local read "User-Defined Quantity"() -> (w178:string)
            n78 = Concatenate Strings(w178, " Color Scale" ("Caption.Text")) -> (w181:string)
            n79 = Concatenate Strings(w178, " Color Map" ("Caption.Text")) -> (w179:string)
            n80 = Concatenate Strings(w178, " Display Range" ("Caption.Text")) -> (w176:string)
          }
        }
        n81 = property on="Phasor Ratio Color Scale" class="ColRmp (strict)"(error in=w145, "Caption.Text"=w155) -> (error out=w152:errorcluster)  [unwired: 1 in, 1 out]
        n82 = property on="Phasor Ratio Color Map" class="Str"(error in=w145, "Caption.Text"=w154) -> (error out=w151:errorcluster)  [unwired: 1 in, 1 out]
        n83 = property class="Slide (strict)"(reference=w149, error in=w145, "Caption.Text"=w148, "Scale.Minimum"=w147, "Scale.Maximum"=w146) -> (reference out=w143:refnum<vi>, error out=w144:errorcluster)
        n84 = Merge Errors(w152, w151, w144) -> (w153:errorcluster)
        n85 = call "AlliGator Set Phasor Ratio Display Range.vi"("error in (no error)"=w153, "Phasor Ratio Display Range"=w143) -> ()  [unwired: 9 in, 1 out]
      }
      frame "Quit" {
      }
      frame "Refresh All Parameters" {
        n86 = call "AlliGator Settings Storage.vi"("AlliGator Settings List"=AlliGator_Settings_List."Miscellaneous:Verbose Settings Mode") -> ("Error Out"=w187:errorcluster, "Variant Data out"=w189:variant)  [unwired: 9 in]
        n87 = call-poly "Variant to Data.vi"("Variant"=w189) -> ("Value"=w188:bool)  [unwired: 8 in]
        n88 = call "AlliGator Refresh All Settings.vi"("Error In"=w187, "Verbose (T)"=w188, "VI Refnum in"=w191) -> ("Error Out"=w186:errorcluster)  [unwired: 8 in]
        n89 = call "Clear Error.vi"("Error In"=w186) -> ()  [unwired: 8 in, 1 out]
      }
      frame "Send Parameters JSON Strings to Clipboard" {
        n90 = Bundle By Name(cluster=T80 {"AlliGator Q Event"=enum."GUI:Send Parameters JSON Strings to Clipboard", "Data"=variant} ("element"), "Data"="Parameter Names only") -> (w194:T80)
        n91 = Build Array(w194) -> (w195:T80[])
        n92 = Enqueue Element(queue=w197, element=w195) -> ()  [unwired: 2 in, 3 out]
      }
      frame "Set Phasor Ratio Color Map" {
        w199 = AlliGator_Variables_List."Phasor Ratio Palette List" ("Alligator Variable")
        n93 = local read "Phasor Ratio Color Map Type"() -> (w204:T46)
        n94 = call "Alligator Variables Storage.vi"("Get(F)/Set"=FALSE, "AlliGator Variable"=w199) -> ("Data out"=w201:variant)  [unwired: 7 in, 2 out]
        n95 = call-poly "Variant to Data.vi"("Variant"=w201) -> ("String Array"=w200:string[])  [unwired: 8 in]
        n96 = call-poly "Variant to Data.vi"("Variant"=w206) -> ("String"=w205:string)  [unwired: 8 in]
        n97 = control-ref of="Phasor Ratio Color Scale"() -> (w203:refnum<vi>)
        n98 = case shown="\"Interpolate Reference Colors\"" w204 {
          tunnel: w205 -> [w210 _]
          tunnel: w203 -> [w209 w240]
          tunnel: w200 -> [w208 _]
          tunnel: w199 -> [w207 _]
          frame "Use Custom Map" {
            n99 = case shown="Default" w210 {
              selector: w210 -> [_ w221]
              tunnel: w209 -> [_ w220]
              tunnel: w208 -> [w212 w218]
              tunnel: w207 -> [w211 w216]
              frame "Edit Palette List..." {
                n100 = call "Edit Image Palette List Dialog.vi"("Palette List (in)"=w212) -> ("Palette List (out)"=w214:string[])  [unwired: 10 in]
                n101 = call "Alligator Variables Storage.vi"("Get(F)/Set"=TRUE, "AlliGator Variable"=w211, "Data in"=w214) -> ()  [unwired: 6 in, 3 out]
              }
              frame Default {
                w225 = TRUE ("Get(F)/Set")
                n102 = call "Get User Palette Choice.vi"("Palette"=w221) -> ("Error Out"=w228:errorcluster, "Palette Colors"=w231:u32[], "Palette Type"=w232:T83, "Palette Name (# Colors)"=w217:string, "Interpolate?"=w227:bool, "Built-in Palette?"=w215:bool)  [unwired: 3 in, 2 out]
                n103 = Bundle(cluster=T82 {"Palette Name [# Colors,int?,inv?]"="", "Palette Type"=0, "Palette Colors"=[], "Interpolate?"=FALSE} ("Image Display Palette Information"), "Palette Name [# Colors,int?,inv?]"=w217, "Palette Type"=w232, "Palette Colors"=w231, "Interpolate?"=w227) -> (w223:T82)
                n104 = call "Alligator Variables Storage.vi"("Get(F)/Set"=w225, "AlliGator Variable"=AlliGator_Variables_List."Phasor Ratio Palette Information" ("Alligator Variable"), "Error In"=w228, "Data in"=w223) -> ("Error Out"=w224:errorcluster)  [unwired: 5 in, 2 out]
                n105 = local write "Phasor Ratio Color Map"(w217) -> ()
                n106 = call "AlliGator Settings Storage.vi"("Get(F)/Set"=w225, "AlliGator Settings List"=AlliGator_Settings_List."Phasor Plot:Phasor Ratio Color Map", "Error In"=w224, "Variant Data in"=w217) -> ("Error Out"=w222:errorcluster)  [unwired: 6 in, 1 out]
                n107 = call "Set Color Ramp Palette v3.vi"("error in (no error)"=w222, "Image Display Palette Information"=w223, "ColorRamp in"=w220) -> ("Error Out"=w219:errorcluster)  [unwired: 6 in, 2 out]
                n108 = case shown="False" w215 {
                  tunnel: w219 -> [w239 _]
                  tunnel: w217 -> [w238 _]
                  tunnel: w218 -> [w237 _]
                  tunnel: w216 -> [w235 _]
                  frame False {
                    n109 = Build Array (concatenate)(w237, w238) -> (w236:string[])
                    n110 = call "Remove Duplicates From 1D Array.vim"("array"=w236) -> ("array with duplicates removed"=w234:string[])  [unwired: 10 in]
                    n111 = call "Alligator Variables Storage.vi"("Get(F)/Set"=TRUE, "AlliGator Variable"=w235, "Error In"=w239, "Data in"=w234) -> ()  [unwired: 5 in, 3 out]
                  }
                  frame True {
                  }
                }
              }
            }
          }
          frame "Interpolate Reference Colors" {
            w249 = TRUE ("Get(F)/Set")
            n112 = property on="Reference 1" class="ColBox"() -> ("Value"=w243:u32)  [unwired: 2 in, 2 out]
            n113 = property on="Reference 2" class="ColBox"() -> ("Value"=w242:u32)  [unwired: 2 in, 2 out]
            n114 = call "AlliGator Get Phasor Ratio Interpolated Color Scale.vi"("Reference 2 Color"=w242, "Reference 1 Color"=w243) -> ("Error Out"=w244:errorcluster, "Interpolated Color Scale Definition"=w245:T84)  [unwired: 8 in]
            n115 = call "Get User Palette Choice.vi"("Error In"=w244, "Interpolated Color Scale Definition"=w245, "Palette"="Interpolated") -> ("Error Out"=w253:errorcluster, "Palette Colors"=w256:u32[], "Palette Type"=w257:T83, "Palette Name (# Colors)"=w251:string, "Interpolate?"=w252:bool)  [unwired: 1 in, 3 out]
            n116 = Bundle(cluster=T82 {"Palette Name [# Colors,int?,inv?]"="", "Palette Type"=0, "Palette Colors"=[], "Interpolate?"=FALSE} ("Image Display Palette Information"), "Palette Name [# Colors,int?,inv?]"=w251, "Palette Type"=w257, "Palette Colors"=w256, "Interpolate?"=w252) -> (w247:T82)
            n117 = call "Alligator Variables Storage.vi"("Get(F)/Set"=w249, "AlliGator Variable"=AlliGator_Variables_List."Phasor Ratio Palette Information" ("Alligator Variable"), "Error In"=w253, "Data in"=w247) -> ("Error Out"=w248:errorcluster)  [unwired: 5 in, 2 out]
            n118 = call "AlliGator Settings Storage.vi"("Get(F)/Set"=w249, "AlliGator Settings List"=AlliGator_Settings_List."Phasor Plot:Phasor Ratio Color Map", "Error In"=w248, "Variant Data in"=w251) -> ("Error Out"=w246:errorcluster)  [unwired: 6 in, 1 out]
            n119 = call "Set Color Ramp Palette v3.vi"("error in (no error)"=w246, "Image Display Palette Information"=w247, "ColorRamp in"=w240) -> ()  [unwired: 6 in, 3 out]
            n120 = local write "Phasor Ratio Color Map"(w251) -> ()
          }
        }
      }
      frame "Set SEPL Parameters to Dataset Ones" {
        n121 = local read "Nanotime Gate Separation"() -> (w263:dbl[unit])
        n122 = local read "# Gates"() -> (w262:u32)
        n123 = control-ref of="Gate Parameters"() -> (w261:refnum<vi>)
        n124 = local read "Gate Width"() -> (w264:dbl[unit])
        n125 = property on="Match Laser Period" class="Bool (strict)"("Value"=FALSE ("Match Laser Period")) -> (error out=w259:errorcluster)  [unwired: 2 in, 1 out]
        n126 = call "AlliGator Update Settings SEPL Parameters.vi"("Gate Duration"=w264, "Error In"=w259, "Gate Separation"=w263, "# Gates"=w262, "Gate Parameters Refnum"=w261) -> ()  [unwired: 6 in, 1 out]
      }
      frame "Shift Decay Checkbox" {
        n127 = control-ref of="Decay Shift Parameters"() -> (w266:refnum<vi>)
        n128 = call "AlliGator Update Settings Decay Shift Parameters Visibility.vi"("Shift Parameters Refnum"=w266) -> ()  [unwired: 9 in, 2 out]
      }
      frame "Show Window" {
        # "This updates the Natural Frequency"
        n129 = local read "Extrapolate Decay"() -> (w270:bool)
        n130 = property on="Extrapolate Decay" class="Bool (strict)"("Val(Sgnl)"=w270) -> (error out=w268:errorcluster)  [unwired: 2 in, 1 out]
        n131 = property class="VI"(reference=w271, error in=w268, "FP.State"=T75."Standard" ("Front Panel Window:State")) -> ()  [unwired: 2 out]
      }
      frame "Smooth Decay Checkbox" {
        n132 = disable-structure shown="Enabled" {
          frame Disabled {
            n133 = property on="Smoothen Decay" class="Bool (strict)"() -> ("Value"=w273:bool)  [unwired: 2 in, 2 out]
            n134 = property on="Smoothing Parameter" class="DigNum (strict)"("Visible"=w273) -> ()  [unwired: 2 in, 2 out]
          }
          frame Enabled {
          }
        }
      }
      frame "Update Natural Frequency" {
        n135 = call "AlliGator Compute Natural Frequency.vi"() -> ("Natural Frequency"=w275:dbl[unit])  [unwired: 10 in, 1 out]
        n136 = local write "Natural Frequency"(w275) -> ()
      }
      frame "Update SEPL Parameters" {
        n137 = property on="Gate Type" class="Enum (strict)"() -> ("Value"=w277:T62)  [unwired: 2 in, 2 out]
        n138 = control-ref of="Decay & IRF Parameters"() -> (w284:refnum<vi>)
        n139 = control-ref of="Phasor Parameters"() -> (w281:refnum<vi>)
        n140 = control-ref of="Gate Parameters"() -> (w282:refnum<vi>)
        n141 = control-ref of="Display Parameters"() -> (w283:refnum<vi>)
        n142 = call "Phasor Explorer Update Parameters.vi"("VI in"=w297) -> ("error out"=w296:errorcluster, "Display Parameters"=w287:T53, "Decay & IRF Parameters"=w288:T58, "Gate Parameters"=w289:T61, "Phasor Parameters"=w290:T55)  [unwired: 3 in, 3 out]
        n143 = Build Array(w281, w282, w284, w283) -> (w280:refnum<vi>[])
        n144 = To Variant(anything=w290) -> (Variant=w292:variant)
        n145 = To Variant(anything=w289) -> (Variant=w293:variant)
        n146 = To Variant(anything=w288) -> (Variant=w294:variant)
        n147 = To Variant(anything=w287) -> (Variant=w291:variant)
        n148 = Equal?(x=Phasor_Gate_Type."User-defined" ("Value"), y=w277) -> (x = y?=w276:bool)
        n149 = call <vilib>:"Clear Errors.vi"("error in (no error)"=w296) -> ("error out"=w295:errorcluster)  [unwired: 5 in, 1 out]
        n150 = Build Array(w292, w293, w294, w291) -> (w286:variant[])
        n151 = property on="Edit User-defined Function" class="Bool"("Visible"=w276) -> ()  [unwired: 2 in, 2 out]
        n152 = for {
          tunnel: w295 -> [w301]
          tunnel: w286 -> [w300] mode=indexing
          tunnel: w285 -> [w299]
          tunnel: w280 -> [w298] mode=indexing
          n153 = call "AlliGator Update Settings & Control.vi"("Error In"=w301, "Value"=w300, "Sender"=w299, "CtlRef"=w298) -> ()  [unwired: 7 in, 1 out]
        }
      }
      frame "Update SEPL Plot" {
        n154 = Enqueue Element(queue=w303, element=T80[] [{"AlliGator Q Event"=enum."Phasor Graph:Update SEPL Plot", "Data"=variant}]) -> ()  [unwired: 2 in, 3 out]
      }
      frame "Use Cursor (Extrapolate) Checkbox" {
        n155 = disable-structure shown="Enabled" {
          disable-tunnel: w306 -> [w312 _]
          frame Disabled {
            n156 = call-poly "Variant to Data.vi"("Variant"=w312) -> ("Value"=w310:bool)  [unwired: 8 in]
            n157 = property on="Use Periodicity" class="Bool (strict)"() -> ("Value"=w309:bool)  [unwired: 2 in, 2 out]
            n158 = Not(x=w310) -> (.not. x?=w311:bool)
            n159 = case shown="True" w310 {
              tunnel: w309 -> [w314 w316]
              tunnel: [w314 _] -> w308
              tunnel: [w313 w315] -> w307
              frame False {
                # "No Cursor: show Head Fraction/Add'l Points if Use Periodicity"
                n160 = Not(x=w314) -> (.not. x?=w313:bool)
              }
              frame True {
                # "Use Cursor: don't show Head Fraction/Add'l Points"
                n161 = Not(x=w316) -> (.not. x?=w315:bool)
              }
            }
            n162 = property on="Head Fraction" class="DigNum (strict)"("Visible"=w308) -> ()  [unwired: 2 in, 2 out]
            n163 = property on="Additional Points" class="DigNum (strict)"("Visible"=w307) -> ()  [unwired: 2 in, 2 out]
            n164 = property on="Tail Fraction" class="DigNum (strict)"("Visible"=w311) -> ()  [unwired: 2 in, 2 out]
          }
          frame Enabled {
          }
        }
      }
      frame "Use File Timestamp Checkbox" {
        # "deprecated"
      }
      frame "Use Fixed ROI Diameter Checkbox" {
        n165 = Enqueue Element(queue=w319, element=T80[] [{"AlliGator Q Event"=enum."Image:Set ROI Diameter", "Data"=variant}]) -> ()  [unwired: 2 in, 3 out]
      }
      frame "Use Periodicity (Extrapolate) Checkbox" {
        n166 = disable-structure shown="Disabled" {
          disable-tunnel: w322 -> [w327 _]
          frame Disabled {
            n167 = call-poly "Variant to Data.vi"("Variant"=w327) -> ("Value"=w324:bool)  [unwired: 8 in]
            n168 = property on="Use Cursors" class="Bool (strict)"() -> ("Value"=w325:bool)  [unwired: 2 in, 2 out]
            n169 = Not(x=w324) -> (.not. x?=w326:bool)
            n170 = case shown="False" w325 {
              tunnel: w324 -> [w328 _]
              tunnel: [w328 _] -> w323
              frame False {
              }
              frame True {
              }
            }
            n171 = property on="Additional Points" class="DigNum (strict)"("Visible"=w326) -> ()  [unwired: 2 in, 2 out]
            n172 = property on="Head Fraction" class="DigNum (strict)"("Visible"=w323) -> ()  [unwired: 2 in, 2 out]
          }
          frame Enabled {
          }
        }
      }
    }
  }
  n173 = case shown="\"Miscellaneous\"" "Settings Tabs" {
    tunnel: "Fluorescence Decay Tabs" -> [_ _ w330 _ _ _ _ _ _ _ _ _]
    tunnel: "SEPL Tabs" -> [_ _ _ _ _ _ _ w332 _ _ _ _]
    tunnel: "Source Image Tabs" -> [w329 _ _ _ _ _ _ _ _ _ _ _]
    tunnel: "Phasor Plot Tabs" -> [_ _ _ _ _ w331 _ _ _ _ _ _]
    frame "Source Image", Default {
      n174 = case shown="\"Image Processing\"" w329 {
        frame "Pixel Processing", Default {
        }
        frame "Image Processing" {
        }
        frame "Image Cosmetics" {
        }
      }
    }
    frame "Data Information" {
    }
    frame "Fluorescence Decay" {
      n175 = case shown="\"Styles\"" w330 {
        frame "Decay Pre-Processing", Default {
        }
        frame "Advanced Analysis" {
        }
        frame "Fit Options" {
        }
        frame "Fit Parameters" {
        }
        frame "Styles" {
        }
      }
    }
    frame "Fluorescence Decay Statistics" {
    }
    frame "Intensity Time Trace" {
    }
    frame "Phasor Plot" {
      n176 = case shown="\"Phasor Plot Calculation\", Default" w331 {
        frame "Phasor Plot Calculation", Default {
        }
        frame "Phasor Plot Information Overlay" {
        }
        frame "Phasor Plot Appearance" {
        }
      }
    }
    frame "Phasor Graph" {
    }
    frame "Single-Exponential Phasor Locus (SEPL)" {
      n177 = case shown="\"IRF\"" w332 {
        frame "Display", Default {
        }
        frame "Phasor" {
        }
        frame "IRF" {
        }
        frame "Gates" {
        }
      }
    }
    frame "Phasor Calibration" {
    }
    frame "Lifetime Analysis" {
    }
    frame "Plugins" {
    }
    frame "Miscellaneous" {
    }
  }
  n178 = while {
    tunnel: w14 -> [w340]
    tunnel: w32 -> [w341]
    tunnel: w19 -> [w339]
    tunnel: w13 -> [w335]
    shift-right: [w337] -> _
    shift-left: w24 -> [w338]
    tunnel: w17 -> [w336]
    stop <- w342 stop-if-true
    n179 = event shown="[19] \"Gate Width\", \"Nanotime Gate Separation\", \"Gate Step\", \"Background Definition Range\", \"Gates to Skip\", \"Reject Low Decay Peak Pixels\", \"Min Peak Value\", \"Time Step\", \"Phasor Plot Size\", \"Phasor Plot Graphics Options\", \"Use Phasor Brightness\", \"Calibration Lifetime\", \"Verbose Mode\", \"Saved Displayed Image File Format\", \"Phasor Ratio Decay Range\", \"Phasor Ratio Reference Colors\", \"Exponential Fading\", \"Include Loading in Timing\", \"1-Normalize Decay\", \"Smoothing Parameter\", \"Beep after Script\", \"Use Backup Calibration if needed\", \"Backup Calibration Type\", \"Reject High Decay Peak Pixels\", \"Max Peak Value\", \"Use Intensity Correction File\", \"Phasor Ratio Type\", \"Fit Options\", \"Pixel-level Phasor Computation\", \"Show Last Decay Only\", \"Decay Graph Color Array\", \"Save Phasor Graph Image\", \"Export Tabulated Results\", \"Peak Threshold\", \"IRF Optimization Options\", \"Wavelet Analysis Options\", \"Tail Fraction\", \"Additional Points\", \"Verbose Settings Mode\", \"Extract IRF instead of Decay\", \"High Count Pixels Rejection Options\", \"Reverse Gates\", \"Laser Period\", \"Pixel Well Capacity\", \"Low Count Pixels Rejection Options\", \"Use Image Brightness\", \"Phasor Plot Smoothing Options\", \"Use Image Histogram for Contrast\", \"ROI Diameter\", \"ROI Center Color\", \"Verbose Error Mode\", \"Straighten Decay\", \"Verbose Decay Pre-Processing\", \"Square Pulse Options\", \"# Gates\", \"Exported Gate Image Settings\", \"Constant Background\", \"Pixel-Normalize Decay\", \"Phasor Ratio Display Range\", \"IRF Extraction Options\", \"Phasor Graph Frequency\", \"SYNC Period\", \"Pile-up Correction\", \"Head Fraction\", \"Invert Binary Mask\", \"Use Decay Pre-Processing\", \"Intensity Threshold\", \"Reference Radius\", \"Gates to Keep\", \"Selected Image ROI(s)\", \"All Image ROIs\", \"All Phasor Plot ROIs\", \"Selected Phasor Plot ROI(s)\", \"Calibration Type\", \"Fold Decay\", \"# Folds\", \"Histogram Options\", \"# Logical Processors Used\", \"Channel Name\", \"Channel Arithmetic\", \"Background File Subtraction\", \"Background Scaling Factor\", \"Background Pile-up Correction\", \"Background Pixel Well Capacity\", \"Define Shortest Lifetime as\", \"Python Settings\", \"Beep on Error\", \"Hot Pixel Removal\", \"Average Lifetime Options\", \"[0-1]-Normalize Decay\", \"Calibration Map Algorithm\", \"Gate Image Exposure\", \"Gate Image Integration\", \"Use Legacy Fitting Approach\", \"ROI Description Max Characters\", \"Available Channel Names\", \"Guess Parameters Options\", \"Transparent Mask Color\", \"Use Data Information Laser Period\", \"Phasor SDV Options\", \"Save Source Image\", \"Draw Reference Segment\", \"Dataset Scaling Factor\", \"Blend Overlay with Image Background\", \"Blend Overlay with Phasor Background\", \"Overlay Analyzed ROI Center\", \"User-Defined Quantity\", \"Scale Bar Options\", \"Image Resolution (Pixel Size)\", \"MLE Baseline Offset Type\", \"MLE Baseline Offset\", \"Flatfield Correction\", \"Dead Left Columns Correction\": Value Change" {
      selector: w341 -> [_ _ _ _ _ _ _ _ _ _ _ _ _ _ _ _ _ _ _ _ _ _ _ _ _ _ _ _ _ _ _ _ _ _ _ _ _ _ _ _ _ _ _ _ _ _ _ _ _ w977 w1033 _ w1044 w1049 _]
      dyn-events: [_ _ _ _ _ _ _ _ _ _ _ _ _ _ _ _ _ _ _ _ _ _ _ _ _ _ _ _ _ _ _ _ _ _ _ _ _ _ _ _ _ _ _ _ _ _ _ _ _ _ w1032 _ w1043 _ _] -> _
      timeout: 25 -> [_ _ _ _ _ _ _ _ _ _ _ _ _ _ _ _ _ _ _ _ _ _ _ _ _ _ _ _ _ _ _ _ _ _ _ _ _ _ _ _ _ _ _ _ _ _ _ _ _ _ _ _ _ _ _]
      tunnel: [_ _ _ _ _ _ _ _ _ _ _ _ _ _ _ _ _ _ _ _ _ _ _ _ _ _ _ _ _ _ _ _ _ _ _ _ _ _ _ _ _ _ _ _ _ _ _ _ _ w980 _ _ _ w1045 _] -> w342
      tunnel: w340 -> [_ _ _ _ _ _ _ _ _ _ _ _ _ _ _ _ _ _ _ w509 _ _ _ _ _ _ _ _ _ _ _ _ _ _ _ _ _ _ w873 _ _ _ _ _ _ _ _ _ _ w983 _ _ _ _ _]
      tunnel: w339 -> [w348 w357 w366 w376 _ _ w394 _ _ w416 w423 w435 w443 _ w478 _ w494 _ _ w508 _ w705 w720 w732 _ _ _ _ w780 _ _ _ _ w836 _ _ _ _ _ _ w912 w920 _ _ w938 w946 w954 w963 _ w981 _ _ _ _ _]
      tunnel: w338 -> [w350 w358 w365 w375 w379 w383 w395 w401 w409 w420 w427 w434 w444 w466 w477 w482 w495 w497 w503 w518 w699 w714 w719 w731 w742 w750 w770 w773 w779 w784 w808 w821 w824 w835 w844 w853 w864 w870 w875 w900 w911 w919 w924 w930 w937 w945 w952 w962 w966 w979 _ w1039 _ w1048 w1050]
      tunnel: [w350 w358 w365 w375 w379 w383 w395 w401 w409 w420 w427 w434 w444 w466 w477 w482 w495 w497 w503 w518 w699 w714 w719 w731 w742 w750 w770 w773 w779 w784 w808 w821 w824 w835 w844 w853 w864 w870 w875 w900 w911 w919 w924 w930 w937 w945 w952 w962 w966 w979 w1029 w1039 w1042 w1048 w1050] -> w337
      tunnel: w336 -> [_ w354 w364 w374 w378 _ _ _ _ _ _ w433 _ w447 w476 _ _ _ _ w515 _ _ _ _ w741 _ _ _ w778 _ w807 _ _ w834 _ _ _ w868 _ _ w910 w918 _ w929 w936 w944 w951 w961 _ w978 _ _ _ w1047 _]
      tunnel: w335 -> [_ _ _ _ _ _ _ _ _ _ _ _ _ _ _ _ _ _ _ _ _ _ _ _ _ _ _ _ _ _ _ _ _ _ _ _ _ _ _ _ _ _ _ _ _ _ _ _ _ w976 _ _ _ _ _]
      tunnel: [w349 w351 w359 w368 _ w380 w393 w398 w406 w415 w422 w430 w442 w445 w472 _ w493 _ _ w511 _ w702 w715 w727 w739 w746 _ _ w774 w782 w805 w816 _ w831 _ _ w854 _ w871 w899 w906 w914 _ _ w933 w940 w948 w958 _ w976 _ w1034 _ _ _] -> w334
      event "Background File", "Intensity Correction File": Value Change {
        # "Fixes a LabVIEW bug in 2021 SP1"
        n180 = event-data() -> ("CtlRef"=w345:refnum<vi>, "NewVal"=w347:path)  [unwired: 1 in]
        n181 = property class="Path"(reference=w345, "Value"=w347) -> (reference out=w344:refnum<vi>, error out=w346:errorcluster, "Label.Text"=w343:string)  [unwired: 1 in]
        n182 = call "AlliGator Update Settings & Control.vi"("Control Label"=w343, "Error In"=w346, "Value"=w347, "Sender"=w348, "CtlRef"=w344) -> ("Error Out"=w349:errorcluster)  [unwired: 6 in]
      }
      event "Background Subtraction": Value Change {
        n183 = event-data() -> ("CtlRef"=w356:refnum<vi>, "NewVal"=w355:bool)  [unwired: 1 in]
        n184 = call "AlliGator Update Settings & Control.vi"("Value"=w355, "Sender"=w357, "CtlRef"=w356) -> ("Error Out"=w353:errorcluster)  [unwired: 8 in]
        n185 = Enqueue Element(queue=w354, element=T77 {"Action"=enum."Baseline Subtraction Method", "Data"=variant}, error in (no error)=w353) -> (error out=w351:errorcluster)  [unwired: 1 in, 2 out]
      }
      event Value Change {
        n186 = event-data() -> ("CtlRef"=w367:refnum<vi>, "NewVal"=w360:T17)  [unwired: 1 in]
        n187 = call "AlliGator Update Settings & Control.vi"("Value"=w360, "Sender"=w366, "CtlRef"=w367) -> ("Error Out"=w363:errorcluster)  [unwired: 8 in]
        n188 = Bundle By Name(cluster=T77 {"Action"=enum."Baseline Subtraction Method", "Data"=variant} ("element"), "Data"=w360) -> (w361:T77)
        n189 = Enqueue Element(queue=w364, element=w361, error in (no error)=w363) -> (error out=w359:errorcluster)  [unwired: 1 in, 2 out]
      }
      event "Cumulative Phasor Plot": Value Change {
        n190 = event-data() -> ("CtlRef"=w372:refnum<vi>, "NewVal"=w369:bool)  [unwired: 1 in]
        n191 = call "AlliGator Update Settings & Control.vi"("Value"=w369, "Sender"=w376, "CtlRef"=w372) -> ("Error Out"=w373:errorcluster)  [unwired: 8 in]
        n192 = Bundle By Name(cluster=T77 {"Action"=enum."Cumulative Phasor Plot Checkbox", "Data"=variant} ("element"), "Data"=w369) -> (w370:T77)
        n193 = Enqueue Element(queue=w374, element=w370, error in (no error)=w373) -> (error out=w368:errorcluster)  [unwired: 1 in, 2 out]
      }
      event "Match Laser Period": Value Change {
        n194 = event-data() -> ()  [unwired: 1 in, 1 out]
        n195 = Enqueue Element(queue=w378, element=T77 {"Action"=enum."Update SEPL Parameters", "Data"=variant}) -> ()  [unwired: 2 in, 3 out]
      }
      event Shortcut Menu Selection (User) {
        n196 = event-data() -> ("ItemTag"=w382:string, "CtlRef"=w381:refnum<vi>)  [unwired: 1 in]
        n197 = case shown="\"Use Dataset Period\"" w382 {
          tunnel: w381 -> [_ w384]
          tunnel: [_ w385] -> w380
          frame "", Default {
          }
          frame "Use Dataset Period" {
            n198 = control-ref of="Laser Period"() -> (w389:refnum<vi>)
            n199 = To More Specific Class(target class=w389, reference=w384) -> (specific class reference=w390:refnum<vi>, error out=w388:errorcluster)  [unwired: 1 in]
            n200 = property class="DigNum (strict)"(reference=w389, error in=w388) -> (error out=w386:errorcluster, "Value"=w387:dbl[unit])  [unwired: 1 out]
            n201 = property class="DigNum (strict)"(reference=w390, error in=w386, "Val(Sgnl)"=w387) -> (error out=w385:errorcluster)  [unwired: 1 out]
          }
        }
      }
      event Value Change {
        n202 = event-data() -> ("CtlRef"=w397:refnum<vi>, "NewVal"=w391:T19)  [unwired: 1 in]
        n203 = call "AlliGator Update Settings Decay Shift Parameters Visibility.vi"("Shift Parameters Refnum"=w397) -> ("error out"=w392:errorcluster, "Shift Parameters Refnum"=w396:refnum<vi>)  [unwired: 9 in]
        n204 = call "AlliGator Update Settings & Control.vi"("Error In"=w392, "Value"=w391, "Sender"=w394, "CtlRef"=w396) -> ("Error Out"=w393:errorcluster)  [unwired: 7 in]
      }
      event "Decay Pre-Processing Operations Order": Shortcut Menu Selection (User) {
        n205 = event-data() -> ("CtlRef"=w400:refnum<vi>, "ItemTag"=w399:string)  [unwired: 1 in]
        n206 = case shown="\"Reorder Operations\"" w399 {
          tunnel: w400 -> [_ w403 w405]
          tunnel: [_ w402 w404] -> w398
          frame "", Default {
          }
          frame "Reorder Operations" {
            n207 = call "AlliGator Reorder Decay Pre-processing Operations.vi"("Ring in"=w403) -> ("Error Out"=w402:errorcluster)  [unwired: 10 in]
          }
          frame "Export JSON String to Clipboard" {
            n208 = call "AlliGator Export Settings Parameter JSON String to Clipboard.vi"("Control Refnum"=w405) -> ("Error Out"=w404:errorcluster)  [unwired: 9 in, 1 out]
          }
        }
      }
      event "Image Pre-Processing Operations Order": Shortcut Menu Selection (User) {
        n209 = event-data() -> ("CtlRef"=w408:refnum<vi>, "ItemTag"=w407:string)  [unwired: 1 in]
        n210 = case shown="\"\", Default" w407 {
          tunnel: w408 -> [_ w411 w413]
          tunnel: [_ w410 w412] -> w406
          frame "", Default {
          }
          frame "Reorder Operations" {
            n211 = call "AlliGator Reorder Decay Pre-processing Operations.vi"("Ring in"=w411) -> ("Error Out"=w410:errorcluster)  [unwired: 10 in]
          }
          frame "Export JSON String to Clipboard" {
            n212 = call "AlliGator Export Settings Parameter JSON String to Clipboard.vi"("Control Refnum"=w413) -> ("Error Out"=w412:errorcluster)  [unwired: 9 in, 1 out]
          }
        }
      }
      event "Decay Pre-Processing Operations Order": Value Change {
        n213 = event-data() -> ("CtlRef"=w419:refnum<vi>)  [unwired: 1 in]
        n214 = property class="Ring (strict)"(reference=w419) -> (reference out=w417:refnum<vi>, error out=w414:errorcluster, "Strings []"=w418:string[])  [unwired: 1 in]
        n215 = call "AlliGator Update Settings & Control.vi"("Error In"=w414, "Value"=w418, "Sender"=w416, "CtlRef"=w417) -> ("Error Out"=w415:errorcluster)  [unwired: 7 in]
      }
      event "Image Pre-Processing Operations Order": Value Change {
        n216 = event-data() -> ("CtlRef"=w426:refnum<vi>)  [unwired: 1 in]
        n217 = property class="Ring (strict)"(reference=w426) -> (reference out=w424:refnum<vi>, error out=w421:errorcluster, "Strings []"=w425:string[])  [unwired: 1 in]
        n218 = call "AlliGator Update Settings & Control.vi"("Error In"=w421, "Value"=w425, "Sender"=w423, "CtlRef"=w424) -> ("Error Out"=w422:errorcluster)  [unwired: 7 in]
      }
      event Value Change {
        n219 = event-data() -> ("CtlRef"=w436:refnum<vi>, "NewVal"=w428:T14)  [unwired: 1 in]
        n220 = call "AlliGator Update Settings & Control.vi"("Value"=w428, "Sender"=w435, "CtlRef"=w436) -> ("Error Out"=w431:errorcluster)  [unwired: 8 in]
        n221 = Bundle By Name(cluster=T77 {"Action"=enum."Define Gates to Use", "Data"=variant} ("element"), "Data"=w428) -> (w429:T77)
        n222 = Enqueue Element(queue=w433, element=w429, error in (no error)=w431) -> (error out=w430:errorcluster)  [unwired: 1 in, 2 out]
      }
      event "Displayed Fit Parameters": Value Change {
        n223 = event-data() -> ("CtlRef"=w441:refnum<vi>, "NewVal"=w440:T42[])  [unwired: 1 in]
        n224 = call "Remove Duplicates From 1D Array.vim"("array"=w440) -> ("array with duplicates removed"=w437:T42[])  [unwired: 10 in]
        n225 = property class="Arr (strict)"(reference=w441, "Value"=w437) -> (reference out=w439:refnum<vi>, error out=w438:errorcluster)  [unwired: 1 in]
        n226 = call "AlliGator Update Settings & Control.vi"("Error In"=w438, "Value"=w437, "Sender"=w443, "CtlRef"=w439) -> ("Error Out"=w442:errorcluster)  [unwired: 7 in]
      }
      event "Edit User-defined Function": Value Change {
        n227 = event-data() -> ("CtlRef"=w463:refnum<vi>)  [unwired: 1 in]
        n228 = property class="Bool"(reference=w463) -> (error out=w461:errorcluster, "BoolText.Text"=w456:string)  [unwired: 1 in, 1 out]
        n229 = Equal?(x="Gate", y=w456) -> (x = y?=w454:bool)
        n230 = Select(t=AlliGator_Settings_List."Single-Exponential Phasor Locus (SEPL):User-defined Gate" ("AlliGator Settings List"), s=w454, f=AlliGator_Settings_List."Single-Exponential Phasor Locus (SEPL):User-defined IRF" ("AlliGator Settings List")) -> (s? t:f=w449:T73)
        n231 = call "AlliGator Settings Storage.vi"("AlliGator Settings List"=w449, "Error In"=w461) -> ("Error Out"=w460:errorcluster, "Variant Data out"=w459:variant)  [unwired: 8 in]
        n232 = Variant To Data(error in=w460, Variant=w459) -> (data=w457:T88, error out=w458:errorcluster)  [unwired: 1 in]
        n233 = Format Into String(format string="User-defined %s Plot" ("Original Graph Name"), error in=w458, w456) -> (resulting string=w465:string, error out=w462:errorcluster)  [unwired: 1 in]
        n234 = call "Plot Editor.vi"("Original Graph Name"=w465, "Error In"=w462, "Plot in"=w457) -> ("Error Out"=w451:errorcluster, "Plot out"=w450:T88)  [unwired: 6 in, 1 out]
        n235 = call "AlliGator Settings Storage.vi"("Get(F)/Set"=TRUE, "AlliGator Settings List"=w449, "Error In"=w451, "Variant Data in"=w450) -> ("Error Out"=w446:errorcluster)  [unwired: 6 in, 1 out]
        n236 = disable-structure shown="Disabled" {
          disable-tunnel: w447 -> [w469 _]
          disable-tunnel: w446 -> [w468 w471]
          disable-tunnel: [w467 w471] -> w445
          frame Disabled {
            n237 = Enqueue Element(queue=w469, element=T77 {"Action"=enum."Update SEPL Plot", "Data"=variant}, error in (no error)=w468) -> (error out=w467:errorcluster)  [unwired: 1 in, 2 out]
          }
          frame Enabled {
          }
        }
      }
      event "Extrapolate Decay": Value Change {
        n238 = event-data() -> ("CtlRef"=w479:refnum<vi>, "NewVal"=w475:bool)  [unwired: 1 in]
        n239 = call "AlliGator Update Settings & Control.vi"("Value"=w475, "Sender"=w478, "CtlRef"=w479) -> ("Error Out"=w474:errorcluster)  [unwired: 8 in]
        n240 = Enqueue Element(queue=w476, element=T77 {"Action"=enum."Extrapolate Decay Checkbox", "Data"=variant}, error in (no error)=w474) -> (error out=w472:errorcluster)  [unwired: 1 in, 2 out]
      }
      event Shortcut Menu Selection (User) {
        n241 = event-data() -> ("CtlRef"=w480:refnum<vi>, "ItemTag"=w481:string)  [unwired: 1 in]
        n242 = case shown="\"Export JSON String to Clipboard\"" w481 {
          tunnel: w480 -> [_ w483 w485]
          frame "", Default {
          }
          frame "Use Data Information >> Laser Period" {
            n243 = property on="Laser Period" class="DigNum (strict)"() -> ("Value"=w484:dbl[unit])  [unwired: 2 in, 2 out]
            n244 = property class="DigNum (strict)"(reference=w483, "Val(Sgnl)"=w484) -> ()  [unwired: 1 in, 2 out]
          }
          frame "Export JSON String to Clipboard" {
            n245 = call "AlliGator Export Settings Parameter JSON String to Clipboard.vi"("Control Refnum"=w485) -> ()  [unwired: 9 in, 2 out]
          }
        }
      }
      event "Fit Parameter Constraints": Value Change {
        n246 = event-data() -> ("CtlRef"=w492:refnum<vi>, "OldVal"=w491:T41[], "NewVal"=w490:T41[])  [unwired: 1 in]
        n247 = call "AlliGator Remove Duplicated Fit Parameter Constraints.vi"("New Constraints in"=w490, "Old Constraints"=w491) -> ("Error Out"=w487:errorcluster, "New Constraints out"=w488:T41[])  [unwired: 8 in]
        n248 = property class="Arr (strict)"(reference=w492, error in=w487, "Value"=w488) -> (reference out=w489:refnum<vi>, error out=w486:errorcluster)
        n249 = call "AlliGator Update Settings & Control.vi"("Error In"=w486, "Value"=w488, "Sender"=w494, "CtlRef"=w489) -> ("Error Out"=w493:errorcluster)  [unwired: 7 in]
      }
      event "Fluorescence Decay Tabs": Value Change {
        n250 = event-data() -> ("NewVal"=w496:T16)  [unwired: 1 in]
        n251 = case shown="\"Decay Pre-Processing\"" w496 {
          frame "Decay Pre-Processing" {
            n252 = call "AlliGator Settings Storage.vi"("AlliGator Settings List"=AlliGator_Settings_List."Fluorescence Decay_Decay Pre-Processing:Decay Pre-Processing Operations Order") -> ("Error Out"=w498:errorcluster, "Variant Data out"=w500:variant)  [unwired: 9 in]
            n253 = call-poly "Variant to Data.vi"("Variant"=w500) -> ("String Array"=w499:string[])  [unwired: 8 in]
            n254 = property on="Decay Pre-Processing Operations Order" class="Ring (strict)"(error in=w498, "Strings []"=w499) -> ()  [unwired: 1 in, 2 out]
          }
          frame "Advanced Analysis", Default {
          }
        }
      }
      event "Source Image Tabs": Value Change {
        n255 = event-data() -> ("NewVal"=w502:T3)  [unwired: 1 in]
        n256 = case shown="\"Image Processing\"" w502 {
          frame "Pixel Processing", Default {
          }
          frame "Image Processing" {
            n257 = call "AlliGator Settings Storage.vi"("AlliGator Settings List"=AlliGator_Settings_List."Source Image:Image Pre-Processing Operations Order") -> ("Error Out"=w504:errorcluster, "Variant Data out"=w506:variant)  [unwired: 9 in]
            n258 = call-poly "Variant to Data.vi"("Variant"=w506) -> ("String Array"=w505:string[])  [unwired: 8 in]
            n259 = property on="Image Pre-Processing Operations Order" class="Ring (strict)"(error in=w504, "Strings []"=w505) -> ()  [unwired: 1 in, 2 out]
          }
        }
      }
      event "Gate Width", "Nanotime Gate Separation", "Gate Step", "Background Definition Range", "Reject Low Decay Peak Pixels", "Min Peak Value", "Time Step", "Use Phasor Brightness", "Calibration Lifetime", "Verbose Mode", "Phasor Ratio Decay Range", "Phasor Ratio Reference Colors", "Exponential Fading", "Include Loading in Timing", "1-Normalize Decay", "Smoothing Parameter", "Beep after Script", "Use Backup Calibration if needed", "Backup Calibration Type", "Reject High Decay Peak Pixels", "Max Peak Value", "Use Intensity Correction File", "Pixel-level Phasor Computation", "Show Last Decay Only", "Decay Graph Color Array", "Save Phasor Graph Image", "Export Tabulated Results", "Peak Threshold", "Tail Fraction", "Additional Points", "Verbose Settings Mode", "Extract IRF instead of Decay", "Reverse Gates", "Laser Period", "Pixel Well Capacity", "Use Image Brightness", "Use Image Histogram for Contrast", "ROI Diameter", "ROI Center Color", "Verbose Error Mode", "Straighten Decay", "Verbose Decay Pre-Processing", "# Gates", "Constant Background", "Pixel-Normalize Decay", "Phasor Ratio Display Range", "Phasor Graph Frequency", "SYNC Period", "Pile-up Correction", "Head Fraction", "Invert Binary Mask", "Use Decay Pre-Processing", "Intensity Threshold", "Reference Radius", "Selected Image ROI(s)", "All Image ROIs", "All Phasor Plot ROIs", "Selected Phasor Plot ROI(s)", "Fold Decay", "# Folds", "# Logical Processors Used", "Channel Name", "Background File Subtraction", "Background Scaling Factor", "Background Pile-up Correction", "Background Pixel Well Capacity", "Beep on Error", "[0-1]-Normalize Decay", "Gate Image Exposure", "Gate Image Integration", "Use Legacy Fitting Approach", "ROI Description Max Characters", "Available Channel Names", "Transparent Mask Color", "Use Data Information Laser Period", "Save Source Image", "Draw Reference Segment", "Dataset Scaling Factor", "Blend Overlay with Image Background", "Blend Overlay with Phasor Background", "Overlay Analyzed ROI Center", "User-Defined Quantity", "Image Resolution (Pixel Size)", "MLE Baseline Offset", "Dead Left Columns Correction": Value Change {
        n260 = event-data() -> ("CtlRef"=w517:refnum<vi>, "NewVal"=w514:variant)  [unwired: 1 in]
        n261 = call "AlliGator Update Settings & Control.vi"("Value"=w514, "Sender"=w508, "CtlRef"=w517) -> ("Error Out"=w512:errorcluster)  [unwired: 8 in]
        n262 = property class="Ctl"(reference=w517, error in=w512) -> (reference out=w510:refnum<vi>, error out=w513:errorcluster, "Label.Text"=w516:string)
        n263 = case shown="\"\", Default" w516 {
          selector: w516 -> [_ _ _ _ _ _ _ _ _ _ w596 _ _ _ _ _ _ _ _ _ _]
          tunnel: w515 -> [_ w523 _ _ _ _ _ _ _ w595 w600 _ w612 w622 w636 w642 _ _ _ _ _]
          tunnel: w514 -> [_ _ w528 w532 w545 w553 _ w579 _ w590 _ w603 w609 _ w634 w641 w656 _ w672 w680 w692]
          tunnel: w513 -> [w519 w521 w524 w531 w543 w551 w562 w574 w581 w594 _ w604 w611 w621 w633 w640 w655 w667 w670 w678 w691]
          tunnel: [w519 w520 w525 w530 w542 w550 w561 w575 w580 w593 w599 w601 w610 w620 w632 w639 w654 w668 w669 w677 w685] -> w511
          tunnel: w508 -> [_ _ _ _ _ _ _ _ _ _ _ _ _ _ w627 w638 _ _ _ _ _]
          tunnel: w510 -> [_ _ _ _ _ _ _ _ _ _ _ _ _ _ _ _ _ w666 _ _ _]
          tunnel: w509 -> [_ _ _ _ _ _ _ _ _ _ _ _ _ _ _ _ _ _ _ _ _]
          frame "", Default {
          }
          frame "# Gates", "Additional Points", "Decay Shift Parameters", "Extrapolate Decay", "Gate Separation", "Gate Step", "Gates to Skip", "Shift Decay", "Use Decay Pre-Processing" {
            n264 = Enqueue Element(queue=w523, element=T77 {"Action"=enum."Update Natural Frequency", "Data"=variant}, error in (no error)=w521) -> (error out=w520:errorcluster)  [unwired: 1 in, 2 out]
          }
          frame "# Logical Processors Used" {
            n265 = call-poly "Variant to Data.vi"("Variant"=w528) -> ("Value"=w526:i32)  [unwired: 8 in]
            n266 = call "Logical Processors Used.vi"("Set/Get (F)"=TRUE, "# Logical Processor Used"=w526) -> ()  [unwired: 4 in, 1 out]
            n267 = call "IMAQ Multi-Core Options"("Get/Set Number of Cores (Get)"=enum32{"Get", "Set", "Set Max Available"}."Set", "error in (no error)"=w524, "Specified Number of Cores"=w526) -> ("error out"=w525:errorcluster)  [unwired: 7 in, 1 out]
          }
          frame "1-Normalize Decay" {
            n268 = disable-structure shown="Disabled" {
              disable-tunnel: w532 -> [w536 _]
              disable-tunnel: w531 -> [w534 _]
              disable-tunnel: [w533 _] -> w530
              frame Disabled {
                n269 = call-poly "Variant to Data.vi"("Variant"=w536) -> ("Value"=w535:bool)  [unwired: 8 in]
                n270 = case shown="True" w535 {
                  selector: w535 -> [_ w541]
                  tunnel: w534 -> [w537 w539]
                  tunnel: [w537 w538] -> w533
                  frame False {
                  }
                  frame True {
                    n271 = Not(x=w541) -> (.not. x?=w540:bool)
                    n272 = property on="Pixel-Normalize Decay" class="Bool (strict)"(error in=w539, "Val(Sgnl)"=w540) -> (error out=w538:errorcluster)  [unwired: 1 in, 1 out]
                  }
                }
              }
              frame Enabled {
              }
            }
          }
          frame "All Image ROIs" {
            n273 = call-poly "Variant to Data.vi"("Variant"=w545) -> ("Value"=w544:bool)  [unwired: 8 in]
            n274 = case shown="False" w544 {
              tunnel: w543 -> [w546 w548]
              tunnel: [w546 w547] -> w542
              frame False {
              }
              frame True {
                n275 = property on="Selected Image ROI(s)" class="Bool (strict)"(error in=w548, "Val(Sgnl)"=FALSE ("Value (Signaling)")) -> (error out=w547:errorcluster)  [unwired: 1 in, 1 out]
              }
            }
          }
          frame "All Phasor Plot ROIs" {
            n276 = call-poly "Variant to Data.vi"("Variant"=w553) -> ("Value"=w552:bool)  [unwired: 8 in]
            n277 = case shown="True" w552 {
              tunnel: w551 -> [w554 w556]
              tunnel: [w554 w555] -> w550
              frame False {
              }
              frame True {
                n278 = property on="Selected Phasor Plot ROI(s)" class="Bool (strict)"(error in=w556, "Val(Sgnl)"=FALSE ("Value (Signaling)")) -> (error out=w555:errorcluster)  [unwired: 1 in, 1 out]
              }
            }
          }
          frame "Backup Calibration Type" {
            n279 = call "AlliGator Settings Storage.vi"("AlliGator Settings List"=AlliGator_Settings_List."Phasor Calibration:Use Backup Calibration if needed") -> ("Variant Data out"=w559:variant)  [unwired: 9 in, 1 out]
            n280 = call-poly "Variant to Data.vi"("Variant"=w559) -> ("Value"=w558:bool)  [unwired: 8 in]
            n281 = case shown="True" w558 {
              tunnel: w562 -> [w563 w565]
              tunnel: [w563 w564] -> w561
              frame False {
              }
              frame True {
                n282 = call "Alligator Variables Storage.vi"("AlliGator Variable"=AlliGator_Variables_List."Phasor Plot Computed" ("Alligator Variable"), "Error In"=w565) -> ("Error Out"=w566:errorcluster, "Data out"=w568:variant)  [unwired: 7 in, 1 out]
                n283 = call-poly "Variant to Data.vi"("Variant"=w568) -> ("Value"=w567:bool)  [unwired: 8 in]
                n284 = case shown="True" w567 {
                  tunnel: w566 -> [w570 w573]
                  tunnel: [w570 w571] -> w564
                  frame False {
                  }
                  frame True {
                    n285 = call "AlliGator Set Phasor Plot Update LED.vi"("error in (no error)"=w573, "Off/On"=TRUE) -> ("error out"=w571:errorcluster)  [unwired: 9 in]
                  }
                }
              }
            }
          }
          frame "Beep on Error" {
            n286 = call-poly "Variant to Data.vi"("Variant"=w579) -> ("Value"=w578:bool)  [unwired: 8 in]
            n287 = call "Notebook Parameter Storage.vi"("Get(F)/Set"=TRUE, "Notebook Parameter List"=Notebook_Parameters_List."Beep on Error?", "Error In"=w574, "Data in"=w578) -> ("Error Out"=w575:errorcluster)  [unwired: 6 in, 1 out]
          }
          frame "Calibration Lifetime", "Calibration Map Algorithm", "Calibration Type", "Use Backup Calibration if needed" {
            n288 = call "Alligator Variables Storage.vi"("AlliGator Variable"=AlliGator_Variables_List."Phasor Plot Computed" ("Alligator Variable"), "Error In"=w581) -> ("Error Out"=w582:errorcluster, "Data out"=w584:variant)  [unwired: 7 in, 1 out]
            n289 = call-poly "Variant to Data.vi"("Variant"=w584) -> ("Value"=w583:bool)  [unwired: 8 in]
            n290 = case shown="True" w583 {
              tunnel: w582 -> [w586 w589]
              tunnel: [w586 w587] -> w580
              frame False {
              }
              frame True {
                n291 = call "AlliGator Set Phasor Plot Update LED.vi"("error in (no error)"=w589, "Off/On"=TRUE) -> ("error out"=w587:errorcluster)  [unwired: 9 in]
              }
            }
          }
          frame "Channel Name" {
            n292 = Bundle By Name(cluster=T77 {"Action"=enum."Channel Name Changed", "Data"=variant} ("element"), "Data"=w590) -> (w591:T77)
            n293 = Enqueue Element(queue=w595, element=w591, error in (no error)=w594) -> (error out=w593:errorcluster)  [unwired: 1 in, 2 out]
          }
          frame "Fit Options", "Use Data Information Laser Period" {
            n294 = Bundle By Name(cluster=T77 {"Action"=enum."Fit Options Changed", "Data"=variant} ("element"), "Data"=w596) -> (w597:T77)
            n295 = Enqueue Element(queue=w600, element=w597) -> (error out=w599:errorcluster)  [unwired: 2 in, 2 out]
          }
          frame "Fold Decay" {
            n296 = call-poly "Variant to Data.vi"("Variant"=w603) -> ("Value"=w602:bool)  [unwired: 8 in]
            n297 = property on="# Folds" class="DigNum (strict)"(error in=w604, "Visible"=w602) -> (error out=w601:errorcluster)  [unwired: 1 in, 1 out]
          }
          frame "Hot Pixel Removal" {
            n298 = Variant To Data(type=T4 {"Remove Screamers"=TRUE, "Delta"=inf, "Equalize Histogram"=FALSE, "Percentile"=0.0, "Hot Pixel Mask Image"=path "", "Use Hot Pixel Mask"=TRUE} ("Hot Pixel Removal"), Variant=w609) -> (data=w607:T4)  [unwired: 1 in, 1 out]
            n299 = Unbundle By Name(w607) -> ("Use Hot Pixel Mask"=w605:bool, "Hot Pixel Mask Image"=w606:path)
            n300 = case shown="True" w605 {
              tunnel: w612 -> [_ w619]
              tunnel: w611 -> [w613 w618]
              tunnel: [w613 w617] -> w610
              tunnel: w606 -> [_ w615]
              frame False {
              }
              frame True {
                n301 = Bundle By Name(cluster=T77 {"Action"=enum."Load Hot Pixel Mask Image", "Data"=variant} ("element"), "Data"=w615) -> (w614:T77)
                n302 = Enqueue Element(queue=w619, element=w614, error in (no error)=w618) -> (error out=w617:errorcluster)  [unwired: 1 in, 2 out]
              }
            }
          }
          frame "IRF Order" {
            n303 = disable-structure shown="Disabled" {
              disable-tunnel: w622 -> [w625 _]
              disable-tunnel: w621 -> [w624 _]
              disable-tunnel: [w623 _] -> w620
              frame Disabled {
                # "hidden control: unused"
                n304 = Enqueue Element(queue=w625, element=T77 {"Action"=enum."Define IRF Time Constants", "Data"=variant}, error in (no error)=w624) -> (error out=w623:errorcluster)  [unwired: 1 in, 2 out]
              }
              frame Enabled {
              }
            }
          }
          frame "Phasor Graph Frequency" {
            n305 = Variant To Data(error in=w633, type=dbl[unit] 0.0 ("Phasor Frequency 2"), Variant=w634) -> (data=w631:dbl[unit], error out=w630:errorcluster)
            n306 = local write "Phasor Plot Frequency"(w631) -> ()
            n307 = control-ref of="Phasor Plot Frequency"() -> (w628:refnum<vi>)
            n308 = call "AlliGator Update Settings & Control.vi"("Error In"=w630, "Value"=w631, "Sender"=w627, "CtlRef"=w628) -> ("Error Out"=w629:errorcluster)  [unwired: 7 in]
            n309 = Enqueue Element(queue=w636, element=T77 {"Action"=enum."Update SEPL Plot", "Data"=variant}, error in (no error)=w629) -> (error out=w632:errorcluster)  [unwired: 1 in, 2 out]
          }
          frame "Phasor Plot Frequency" {
            n310 = disable-structure shown="Disabled" {
              disable-tunnel: w642 -> [w652 _]
              disable-tunnel: w641 -> [w650 _]
              disable-tunnel: w640 -> [w649 _]
              disable-tunnel: [w648 _] -> w639
              disable-tunnel: w638 -> [w645 _]
              frame Disabled {
                n311 = Variant To Data(error in=w649, type=dbl[unit] 0.0 ("Phasor Frequency 2"), Variant=w650) -> (data=w643:dbl[unit], error out=w647:errorcluster)
                n312 = local write "Phasor Graph Frequency"(w643) -> ()
                n313 = control-ref of="Phasor Graph Frequency"() -> (w646:refnum<vi>)
                n314 = call "AlliGator Update Settings & Control.vi"("Error In"=w647, "Value"=w643, "Sender"=w645, "CtlRef"=w646) -> ("Error Out"=w644:errorcluster)  [unwired: 7 in]
                n315 = Enqueue Element(queue=w652, element=T77 {"Action"=enum."Update SEPL Plot", "Data"=variant}, error in (no error)=w644) -> (error out=w648:errorcluster)  [unwired: 1 in, 2 out]
              }
              frame Enabled {
              }
            }
          }
          frame "Pixel-Normalize Decay" {
            n316 = disable-structure shown="Disabled" {
              disable-tunnel: w656 -> [w660 _]
              disable-tunnel: w655 -> [w658 _]
              disable-tunnel: [w657 _] -> w654
              frame Disabled {
                n317 = call-poly "Variant to Data.vi"("Variant"=w660) -> ("Value"=w659:bool)  [unwired: 8 in]
                n318 = case shown="True" w659 {
                  selector: w659 -> [_ w665]
                  tunnel: w658 -> [w661 w663]
                  tunnel: [w661 w662] -> w657
                  frame False {
                  }
                  frame True {
                    n319 = Not(x=w665) -> (.not. x?=w664:bool)
                    n320 = property on="1-Normalize Decay" class="Bool (strict)"(error in=w663, "Val(Sgnl)"=w664) -> (error out=w662:errorcluster)  [unwired: 1 in, 1 out]
                  }
                }
              }
              frame Enabled {
              }
            }
          }
          frame "Python Settings" {
            n321 = call "AlliGator Update Settings Python Options.vi"("error in (no error)"=w667, "Python Settings Refnum"=w666) -> ("error out"=w668:errorcluster)  [unwired: 9 in]
          }
          frame "Selected Image ROI(s)" {
            n322 = call-poly "Variant to Data.vi"("Variant"=w672) -> ("Value"=w671:bool)  [unwired: 8 in]
            n323 = case shown="True" w671 {
              tunnel: w670 -> [w673 w675]
              tunnel: [w673 w674] -> w669
              frame False {
              }
              frame True {
                n324 = property on="All Image ROIs" class="Bool (strict)"(error in=w675, "Val(Sgnl)"=FALSE ("Value (Signaling)")) -> (error out=w674:errorcluster)  [unwired: 1 in, 1 out]
              }
            }
          }
          frame "Selected Phasor Plot ROI(s)" {
            n325 = call-poly "Variant to Data.vi"("Variant"=w680) -> ("Value"=w679:bool)  [unwired: 8 in]
            n326 = case shown="True" w679 {
              tunnel: w678 -> [w681 w683]
              tunnel: [w681 w682] -> w677
              frame False {
              }
              frame True {
                n327 = property on="All Phasor Plot ROIs" class="Bool (strict)"(error in=w683, "Val(Sgnl)"=FALSE ("Value (Signaling)")) -> (error out=w682:errorcluster)  [unwired: 1 in, 1 out]
              }
            }
          }
          frame "MLE Baseline Offset Type" {
            n328 = Variant To Data(error in=w691, type=MLE_Baseline_Offset_Type."Absolute" ("MLE Baseline Offset Type"), Variant=w692) -> (data=w689:T38, error out=w686:errorcluster)
            n329 = case shown="\"Absolute\", Default" w689 {
              tunnel: [inf ("Data Entry Limits:Maximum") 100.0 ("Data Entry Limits:Maximum")] -> w688
              tunnel: [-inf ("Data Entry Limits:Minimum") 0.0 ("Data Entry Limits:Minimum")] -> w687
              frame "Absolute", Default {
              }
              frame "Percentage" {
              }
            }
            n330 = property on="MLE Baseline Offset" class="DigNum (strict)"(error in=w686, "Maximum"=w688, "Minimum"=w687) -> (error out=w685:errorcluster)  [unwired: 1 in, 1 out]
          }
        }
      }
      event "Extract IRF instead of Decay", "ROI Diameter", "Use Fixed ROI Diameter", "Verbose Mode", "Use Image Brightness", "Use Phasor Brightness", "ROI Center Color", "Use Image Histogram for Contrast", "Nanotime Gate Separation", "Gate Width", "Gate Step", "Background Subtraction", "Background Definition Range", "Reject Low Decay Peak Pixels", "Time Step", "Use File Timestamp", "Cumulative Phasor Plot", "Calibration Lifetime", "Min Peak Value", "Phasor Ratio Decay Range", "Phasor Ratio Reference Colors", "Exponential Fading", "Include Loading in Timing", "1-Normalize Decay", "Smoothing Parameter", "Smoothen Decay", "Shift Decay", "Use Backup Calibration if needed", "Backup Calibration Type", "Reject High Decay Peak Pixels", "Max Peak Value", "Use Intensity Correction File", "Intensity Correction File", "Show Last Decay Only", "Decay Graph Color Array", "Displayed Fit Parameters", "Fit Parameter Constraints", "Save Phasor Graph Image", "Export Tabulated Results", "Peak Threshold", "Extrapolate Decay", "Tail Fraction", "Additional Points", "Verbose Settings Mode", "Reverse Gates", "Laser Period", "Pile-up Correction", "Pixel Well Capacity", "Guess Parameter Values", "Use Guess Parameters", "Guess Parameter Names", "Verbose Error Mode", "Straighten Decay", "Phasor Ratio Color Map Type", "Restore Skipped Dialogs", "Verbose Decay Pre-Processing", "Fluorescence Decay Graph Default Plot Style", "Lifetime Analysis Graph Default Plot Style", "# Gates", "Ref 2 Label", "Ref 1 Label", "Constant Background", "Pixel-Normalize Decay", "Phasor Ratio Display Range", "Use Current Dataset Parameters", "Use Last Fitted Parameters", "Use Periodicity", "Use Cursors", "Head Fraction", "Invert Binary Mask", "Use Decay Pre-Processing", "Match Laser Period", "Intensity Threshold", "Reference Radius", "Selected Image ROI(s)", "All Image ROIs", "Selected Phasor Plot ROI(s)", "All Phasor Plot ROIs", "Fold Decay", "# Folds", "# Logical Processors", "# Logical Processors Used", "Channel Name", "Background Pixel Well Capacity", "Background Pile-up Correction", "Background File", "Background Scaling Factor", "Background File Subtraction", "Valid Python Session", "[0-1]-Normalize Decay": Shortcut Menu Selection (User) {
        n331 = event-data() -> ("CtlRef"=w698:refnum<vi>, "ItemTag"=w697:string)  [unwired: 1 in]
        n332 = case shown="\"\", Default" w697 {
          tunnel: w698 -> [_ w700]
          frame "", Default {
          }
          frame "Export JSON String to Clipboard" {
            n333 = call "AlliGator Export Settings Parameter JSON String to Clipboard.vi"("Control Refnum"=w700) -> ()  [unwired: 9 in, 2 out]
          }
        }
      }
      event "Guess Parameter Values", "Guess Parameter Names": Value Change {
        n334 = event-data() -> ("CtlRef"=w713:refnum<vi>, "OldVal"=w711:variant)  [unwired: 1 in]
        n335 = property class="Arr"(reference=w713) -> (error out=w710:errorcluster, "Label.Text"=w712:string)  [unwired: 1 in, 1 out]
        n336 = control-ref of="Guess Parameter Values"() -> (w709:refnum<vi>)
        n337 = control-ref of="Guess Parameter Names"() -> (w704:refnum<vi>)
        n338 = call "AlliGator Update Settings Guess Parameter Arrays.vi"("Modified Control"=w712, "Error In"=w710, "Old Value"=w711, "Guess Parameter Names"=w704, "Guess Parameters"=w709) -> ("Error Out"=w707:errorcluster, "Guess Parameter Name Array"=w706:T40[], "Guess Parameter Array"=w708:dbl[])  [unwired: 4 in]
        n339 = call "AlliGator Update Settings & Control.vi"("Error In"=w707, "Value"=w708, "Sender"=w705, "CtlRef"=w709) -> ("Error Out"=w703:errorcluster)  [unwired: 7 in]
        n340 = call "AlliGator Update Settings & Control.vi"("Error In"=w707, "Value"=w706, "Sender"=w705, "CtlRef"=w704) -> ("Error Out"=w701:errorcluster)  [unwired: 7 in]
        n341 = Merge Errors(w703, w701) -> (w702:errorcluster)
      }
      event Value Change {
        n342 = event-data() -> ("CtlRef"=w721:refnum<vi>, "NewVal"=w718:T10)  [unwired: 1 in]
        n343 = Unbundle By Name(w718) -> ("Use Image Binning"=w717:bool)
        n344 = call "AlliGator Update Settings & Control.vi"("Value"=w718, "Sender"=w720, "CtlRef"=w721) -> ("Error Out"=w716:errorcluster)  [unwired: 8 in]
        n345 = case shown="False" w717 {
          selector: w717 -> [_ w726]
          tunnel: w716 -> [w722 w724]
          tunnel: [w722 w723] -> w715
          frame False {
          }
          frame True {
            n346 = Not(x=w726) -> (.not. x?=w725:bool)
            n347 = property on="Use Image Smoothing" class="Bool (strict)"(error in=w724, "Val(Sgnl)"=w725) -> (error out=w723:errorcluster)  [unwired: 1 in, 1 out]
          }
        }
      }
      event Value Change {
        n348 = event-data() -> ("CtlRef"=w733:refnum<vi>, "NewVal"=w730:T7)  [unwired: 1 in]
        n349 = Unbundle By Name(w730) -> ("Use Image Smoothing"=w729:bool)
        n350 = call "AlliGator Update Settings & Control.vi"("Value"=w730, "Sender"=w732, "CtlRef"=w733) -> ("Error Out"=w728:errorcluster)  [unwired: 8 in]
        n351 = case shown="False" w729 {
          selector: w729 -> [_ w738]
          tunnel: w728 -> [w734 w736]
          tunnel: [w734 w735] -> w727
          frame False {
          }
          frame True {
            n352 = Not(x=w738) -> (.not. x?=w737:bool)
            n353 = property on="Use Image Binning" class="Bool (strict)"(error in=w736, "Val(Sgnl)"=w737) -> (error out=w735:errorcluster)  [unwired: 1 in, 1 out]
          }
        }
      }
      event "Natural Frequency": Shortcut Menu Selection (User) {
        n354 = event-data() -> ()  [unwired: 1 in, 1 out]
        n355 = Enqueue Element(queue=w741, element=T77 {"Action"=enum."Update Natural Frequency", "Data"=variant}) -> (error out=w739:errorcluster)  [unwired: 2 in, 2 out]
      }
      event "Phasor Plot Frequency", "Phasor Graph Frequency": Shortcut Menu Selection (User) {
        n356 = event-data() -> ("CtlRef"=w745:refnum<vi>, "ItemTag"=w749:string)  [unwired: 1 in]
        n357 = case shown="\"Use Harmonic of Current Frequency (n > 1)\"" w749 {
          tunnel: [_ 1 ("Harmonic (1)") 1 ("Harmonic (1)") _ _ _ 1 ("Harmonic (1)") _] -> w748
          tunnel: [_ _ TRUE ("Use n/D") _ TRUE ("Use n/D") _ _ _] -> w747
          tunnel: w745 -> [_ _ _ _ _ _ _ w768]
          tunnel: [_ TRUE TRUE TRUE TRUE TRUE w766 _] -> w744
          tunnel: [_ _ _ _ _ TRUE ("Use n/D") w766 _] -> w743
          frame "", Default {
          }
          frame "f = 1/T" {
          }
          frame "f = 1/D" {
          }
          frame "f = n/T (n > 1)" {
          }
          frame "f = n/D (n > 1)" {
          }
          frame "Use Harmonic of Current Frequency (n > 1)" {
          }
          frame "Use Current Frequency" {
            w766 = TRUE
          }
          frame "Export JSON String to Clipboard" {
            n358 = call "AlliGator Export Settings Parameter JSON String to Clipboard.vi"("Control Refnum"=w768) -> ()  [unwired: 9 in, 2 out]
          }
        }
        n359 = case shown="True" w744 {
          tunnel: w748 -> [_ w755]
          tunnel: w747 -> [_ w754]
          tunnel: [_ w753] -> w746
          tunnel: w745 -> [_ w752]
          tunnel: w743 -> [_ w751]
          frame False {
          }
          frame True {
            n360 = call "AlliGator Set Phasor Harmonic.vi"("Use n/D"=w754, "Harmonic (1)"=w755, "Use Current Frequency"=w751, "Phasor Frequency Refnum"=w752) -> ("Error Out"=w753:errorcluster)  [unwired: 7 in]
          }
        }
      }
      event "Phasor Plot Frequency": Value Change {
        n361 = event-data() -> ("NewVal"=w769:dbl[unit])  [unwired: 1 in]
        n362 = property on="Phasor Graph Frequency" class="DigNum (strict)"("Val(Sgnl)"=w769) -> ()  [unwired: 2 in, 2 out]
      }
      event "Extract IRF instead of Decay", "ROI Diameter", "Use Fixed ROI Diameter", "Verbose Mode", "Use Image Brightness", "Use Phasor Brightness", "ROI Center Color", "Use Image Histogram for Contrast", "Nanotime Gate Separation", "Gate Width", "Gate Step", "Background Subtraction", "Background Definition Range", "Reject Low Decay Peak Pixels", "Time Step", "Use File Timestamp", "Cumulative Phasor Plot", "Calibration Lifetime", "Min Peak Value", "Phasor Ratio Decay Range", "Phasor Ratio Reference Colors", "Exponential Fading", "Include Loading in Timing", "1-Normalize Decay", "Smoothing Parameter", "Smoothen Decay", "Shift Decay", "Use Backup Calibration if needed", "Backup Calibration Type", "Reject High Decay Peak Pixels", "Max Peak Value", "Use Intensity Correction File", "Intensity Correction File", "Pixel-level Phasor Computation", "Show Last Decay Only", "Decay Graph Color Array", "Displayed Fit Parameters", "Fit Parameter Constraints", "Save Phasor Graph Image", "Export Tabulated Results", "Peak Threshold", "Extrapolate Decay", "Tail Fraction", "Additional Points", "Verbose Settings Mode", "Reverse Gates", "Laser Period", "Pile-up Correction", "Pixel Well Capacity", "Guess Parameter Values", "Use Guess Parameters", "Guess Parameter Names", "Verbose Error Mode", "Straighten Decay", "Phasor Ratio Color Map Type", "Decay Pre-Processing Operations Order", "Restore Skipped Dialogs", "Verbose Decay Pre-Processing", "Phasor Plot Frequency", "Fluorescence Decay Graph Default Plot Style", "Lifetime Analysis Graph Default Plot Style", "# Gates", "Ref 2 Label", "Ref 1 Label", "Constant Background", "Pixel-Normalize Decay", "Phasor Ratio Display Range", "Phasor Graph Frequency", "Use Current Dataset Parameters", "SYNC Period", "Use Last Fitted Parameters", "Use Periodicity", "Use Cursors", "Head Fraction", "Invert Binary Mask", "Use Decay Pre-Processing", "Match Laser Period", "Intensity Threshold", "Reference Radius", "Selected Image ROI(s)", "All Image ROIs", "All Phasor Plot ROIs", "Fold Decay", "# Folds", "# Logical Processors", "# Logical Processors Used", "Channel Name", "Background Pixel Well Capacity", "Background Pile-up Correction", "Background File", "Background Scaling Factor", "Background File Subtraction", "Available Channel Names", "[0-1]-Normalize Decay": Shortcut Menu Activation? {
        n363 = event-data() -> ("MenuRef"=w772:refnum<k9>)  [unwired: 1 in]
        n364 = Insert Menu Items(8:string[] ["APP_SEPARATOR", "Export JSON String to Clipboard"], 9:w772) -> ()  [unwired: 4 in, 3 out]
        n365 = event-data() -> ()  [unwired: 2 in, 1 out]
      }
      event "Phasor Ratio Color Map Type": Value Change {
        n366 = event-data() -> ("CtlRef"=w781:refnum<vi>, "NewVal"=w777:T46)  [unwired: 1 in]
        n367 = call "AlliGator Update Settings & Control.vi"("Value"=w777, "Sender"=w780, "CtlRef"=w781) -> ("Error Out"=w776:errorcluster)  [unwired: 8 in]
        n368 = Enqueue Element(queue=w778, element=T77 {"Action"=enum."Phasor Ratio Color Map Type Radio Button", "Data"=variant}, error in (no error)=w776) -> (error out=w774:errorcluster)  [unwired: 1 in, 2 out]
      }
      event "Phasor Ratio Color Map": Shortcut Menu Activation? {
        n369 = event-data() -> ("MenuRef"=w783:refnum<k9>)  [unwired: 1 in]
        n370 = flat-sequence {
          tunnel: w783 -> [w789]
          tunnel: [w785] -> w782
          frame #0 {
            w790 = AlliGator_Variables_List."Phasor Ratio Palette List" ("Alligator Variable")
            n371 = call "Alligator Variables Storage.vi"("Get(F)/Set"=FALSE, "AlliGator Variable"=AlliGator_Variables_List."Phasor Ratio Palette Information" ("Alligator Variable")) -> ("Error Out"=w800:errorcluster, "Data out"=w801:variant)  [unwired: 7 in, 1 out]
            n372 = call "Alligator Variables Storage.vi"("Get(F)/Set"=FALSE, "AlliGator Variable"=w790) -> ("Error Out"=w787:errorcluster, "Data out"=w794:variant)  [unwired: 7 in, 1 out]
            n373 = Variant To Data(error in=w800, type=T82 {"Palette Name [# Colors,int?,inv?]"="", "Palette Type"=0, "Palette Colors"=[], "Interpolate?"=FALSE} ("Image Display Palette Information"), Variant=w801) -> (data=w799:T82, error out=w798:errorcluster)
            n374 = call-poly "Variant to Data.vi"("Variant"=w794) -> ("String Array"=w793:string[])  [unwired: 8 in]
            n375 = Unbundle By Name(w799) -> ("Palette Name [# Colors,int?,inv?]"=w796:string)
            n376 = Merge Errors(w798, w787) -> (w788:errorcluster)
            n377 = call "Check Selected Palette in Menu.vi"("Error In"=w788, "Palette List"=w793, "Checked Palette"=w796, "Menu in"=w789) -> ("Error Out"=w786:errorcluster, "Stored Palette List"=w791:string[])  [unwired: 5 in, 1 out]
            n378 = call "Alligator Variables Storage.vi"("Get(F)/Set"=TRUE, "AlliGator Variable"=w790, "Error In"=w786, "Data in"=w791) -> ("Error Out"=w785:errorcluster)  [unwired: 5 in, 2 out]
          }
        }
        n379 = event-data() -> ()  [unwired: 2 in, 1 out]
      }
      event "Phasor Ratio Color Map": Shortcut Menu Selection (User) {
        n380 = event-data() -> ("CtlRef"=w804:refnum<vi>, "ItemTag"=w806:string)  [unwired: 1 in]
        n381 = case shown="\"\", Default" w806 {
          selector: w806 -> [w811 _]
          tunnel: w807 -> [w813 _]
          tunnel: [w809 w814] -> w805
          tunnel: w804 -> [_ w815]
          frame "", Default {
            n382 = Bundle By Name(cluster=T77 {"Action"=enum."Set Phasor Ratio Color Map", "Data"=variant} ("element"), "Data"=w811) -> (w810:T77)
            n383 = Enqueue Element(queue=w813, element=w810) -> (error out=w809:errorcluster)  [unwired: 2 in, 2 out]
          }
          frame "Export JSON String to Clipboard" {
            n384 = call "AlliGator Export Settings Parameter JSON String to Clipboard.vi"("Control Refnum"=w815) -> ("Error Out"=w814:errorcluster)  [unwired: 9 in, 1 out]
          }
        }
      }
      event "Phasor Ratio Color Scale": Shortcut Menu Activation? {
        w819 = string[] ["Copy Color Scale to Clipboard"] ("item names")
        n385 = event-data() -> ("MenuRef"=w818:refnum<k9>)  [unwired: 1 in]
        n386 = Delete Menu Items(9:w818) -> (0:w817:errorcluster, 3:w820:refnum<k9>)  [unwired: 3 in]
        n387 = Insert Menu Items(6:w817, 7:w819, 8:w819, 9:w820) -> (0:w816:errorcluster)  [unwired: 2 in, 2 out]
        n388 = event-data() -> ()  [unwired: 2 in, 1 out]
      }
      event "Phasor Ratio Color Scale": Shortcut Menu Selection (User) {
        n389 = event-data() -> ("CtlRef"=w823:refnum<vi>, "ItemTag"=w822:string)  [unwired: 1 in]
        n390 = case shown="\"Export JSON String to Clipboard\"" w822 {
          tunnel: w823 -> [_ w825 w826]
          frame "", Default {
          }
          frame "Copy Color Scale to Clipboard" {
            n391 = call "Export Color Ramp to Clipboard.vi"("ColorRamp in"=w825) -> ()  [unwired: 11 in]
          }
          frame "Export JSON String to Clipboard" {
            n392 = call "AlliGator Export Settings Parameter JSON String to Clipboard.vi"("Control Refnum"=w826) -> ()  [unwired: 9 in, 2 out]
          }
        }
      }
      event Value Change {
        n393 = event-data() -> ("CtlRef"=w837:refnum<vi>, "NewVal"=w829:T47)  [unwired: 1 in]
        n394 = call "AlliGator Update Settings & Control.vi"("Value"=w829, "Sender"=w836, "CtlRef"=w837) -> ("Error Out"=w832:errorcluster)  [unwired: 8 in]
        n395 = Equal?(x=w829, y=AlliGator_Phasor_Ratio_Color-Coded_Quantity."User-Defined Quantity" ("NewVal")) -> (x = y?=w827:bool)
        n396 = property on="User-Defined Quantity" class="Str"("Visible"=w827) -> ()  [unwired: 2 in, 2 out]
        n397 = Bundle By Name(cluster=T77 {"Action"=enum."Phasor Ratio Color-Coded Quantity Changed", "Data"=variant} ("element"), "Data"=w829) -> (w830:T77)
        n398 = Enqueue Element(queue=w834, element=w830, error in (no error)=w832) -> (error out=w831:errorcluster)  [unwired: 1 in, 2 out]
      }
      event "Plugins Folder": Value Change {
        n399 = event-data() -> ()  [unwired: 1 in, 1 out]
        n400 = call <vilib>:"Application Directory.vi"() -> ("Application Directory"=w843:path)
        n401 = Build Path(base path=w843, name or relative path=path "Python Plugins") -> (appended path=w839:path)
        n402 = Path To String(path=w839) -> (string=w838:string)
        n403 = Concatenate Strings("explorer.exe " ("command line"), w838) -> (w840:string)
        n404 = call <vilib>:"System Exec.vi"("command line"=w840) -> ()  [unwired: 7 in, 4 out]
      }
      event "Reset Python Session": Value Change {
        n405 = event-data() -> ("CtlRef"=w846:refnum<vi>)  [unwired: 1 in]
        n406 = property class="Bool"(reference=w846) -> ("Label.Text"=w845:string)  [unwired: 1 in, 2 out]
        n407 = call "AlliGator Reset Python Session.vi"() -> ("error out"=w850:errorcluster, "Valid Python Session"=w852:bool, "Message"=w851:string)  [unwired: 7 in, 2 out]
        n408 = call "Get Notebook Queue.vi"() -> ("Notebook Queue"=w849:refnum<queue>)  [unwired: 9 in]
        n409 = property on="Valid Python Session" class="Bool (strict)"("Value"=w852) -> ()  [unwired: 2 in, 2 out]
        n410 = call "Send Message to Notebook.vi"("Error In"=w850, "Message"=w851, "Notebook Queue"=w849) -> ("Error Out"=w848:errorcluster, "Notebook Queue"=w847:refnum<queue>)  [unwired: 5 in]
        n411 = call "Send Error to Notebook.vi"("error in (no error)"=w848, "State Machine Case Error Source"=w845, "Notebook Q"=w847) -> ()  [unwired: 8 in, 1 out]
      }
      event "Restore Skipped Dialogs": Value Change {
        w858 = AlliGator_Variables_List."Skippable Dialog Windows Status" ("Alligator Variable")
        n412 = event-data() -> ()  [unwired: 1 in, 1 out]
        n413 = call "Alligator Variables Storage.vi"("AlliGator Variable"=w858) -> ("Error Out"=w862:errorcluster, "Data out"=w863:variant)  [unwired: 8 in, 1 out]
        n414 = Variant To Data(error in=w862, type=T86[] [], Variant=w863) -> (data=w860:T86[], error out=w856:errorcluster)
        n415 = for {
          tunnel: w860 -> [w867] mode=indexing
          tunnel: [w866] -> w859 mode=indexing
          tunnel: FALSE ("NewVal") -> [w865]
          n416 = Bundle By Name(cluster=w867, "Is skipped"=w865) -> (w866:T86)
        }
        n417 = call "Alligator Variables Storage.vi"("Get(F)/Set"=TRUE, "AlliGator Variable"=w858, "Error In"=w856, "Data in"=w859) -> ("Error Out"=w854:errorcluster)  [unwired: 5 in, 2 out]
      }
      event "Send JSON to Clipboard": Value Change {
        n418 = event-data() -> ()  [unwired: 1 in, 1 out]
        n419 = Enqueue Element(queue=w868, element=T77 {"Action"=enum."Send Parameters JSON Strings to Clipboard", "Data"=variant}) -> ()  [unwired: 2 in, 3 out]
      }
      event "Settings Tabs", "Fluorescence Decay Tabs": Shortcut Menu Selection (User) {
        n420 = event-data() -> ("CtlRef"=w872:refnum<vi>, "ItemTag"=w874:string)  [unwired: 1 in]
        n421 = case shown="\"Reset Parameters to Default (this panel only)\"" w874 {
          tunnel: w873 -> [_ _ _]
          tunnel: w872 -> [_ w886 _]
          tunnel: [_ w876 _] -> w871
          frame "", Default {
          }
          frame "Reset Parameters to Default (this panel only)" {
            n422 = property class="TabCtl"(reference=w886) -> (error out=w883:errorcluster, "Pages"=w882:refnum<vi>[], "Value"=w885:variant)  [unwired: 1 in, 1 out]
            n423 = Variant To Data(type=u32 0 ("index"), Variant=w885) -> (data=w880:u32)  [unwired: 1 in, 1 out]
            n424 = Index Array(array=w882, index=w880) -> (element=w884:refnum<vi>)
            n425 = property class="Page"(reference=w884, error in=w883) -> (error out=w881:errorcluster, "PageLabel"=w878:string)  [unwired: 1 out]
            n426 = Close Reference(reference=w882, error in (no error)=w881) -> ()  [unwired: 1 out]
            n427 = call "AlliGator Init Settings v2.vi"("Settings Panel (Empty: All)"=w878) -> ("error out"=w877:errorcluster)  [unwired: 10 in]
            n428 = case shown="\"Decay Pre-Processing\"" w878 {
              tunnel: w877 -> [w887 w889]
              tunnel: [w887 w888] -> w876
              frame "", Default {
              }
              frame "Decay Pre-Processing" {
                # "Special item to handle"
                n429 = call "AlliGator Settings Storage.vi"("AlliGator Settings List"=AlliGator_Settings_List."Fluorescence Decay_Decay Pre-Processing:Decay Pre-Processing Operations Order", "Error In"=w889) -> ("Error Out"=w891:errorcluster, "Variant Data out"=w893:variant)  [unwired: 8 in]
                n430 = call-poly "Variant to Data.vi"("Variant"=w893) -> ("String Array"=w892:string[])  [unwired: 8 in]
                n431 = property on="Decay Pre-Processing Operations Order" class="Ring (strict)"(error in=w891, "Strings []"=w892) -> (error out=w888:errorcluster)  [unwired: 1 in, 1 out]
              }
            }
          }
          frame "Reset All Parameters to Default" {
            n432 = call "AlliGator Init Settings v2.vi"() -> ("error out"=w894:errorcluster)  [unwired: 11 in]
            n433 = call "AlliGator Settings Storage.vi"("AlliGator Settings List"=AlliGator_Settings_List."Fluorescence Decay_Decay Pre-Processing:Decay Pre-Processing Operations Order", "Error In"=w894) -> ("Error Out"=w896:errorcluster, "Variant Data out"=w898:variant)  [unwired: 8 in]
            n434 = call-poly "Variant to Data.vi"("Variant"=w898) -> ("String Array"=w897:string[])  [unwired: 8 in]
            n435 = property on="Decay Pre-Processing Operations Order" class="Ring (strict)"(error in=w896, "Strings []"=w897) -> ()  [unwired: 1 in, 2 out]
          }
        }
      }
      event "Settings Tabs": Value Change {
        n436 = event-data() -> ("NewVal"=w905:T2)  [unwired: 1 in]
        n437 = Format Into String(w905) -> (resulting string=w903:string)  [unwired: 3 in, 1 out]
        n438 = call "AlliGator Settings Storage.vi"("Get(F)/Set"=TRUE, "AlliGator Settings List"=AlliGator_Settings_List."GUI:Visible Settings Tab", "Variant Data in"=w903) -> ("Error Out"=w901:errorcluster)  [unwired: 7 in, 1 out]
        n439 = call "AlliGator Settings Event Refnum.vi"("Error In"=w901) -> ("Error Out"=w899:errorcluster)  [unwired: 7 in, 1 out]
      }
      event "Shift Decay": Value Change {
        n440 = event-data() -> ("CtlRef"=w913:refnum<vi>, "NewVal"=w909:bool)  [unwired: 1 in]
        n441 = call "AlliGator Update Settings & Control.vi"("Value"=w909, "Sender"=w912, "CtlRef"=w913) -> ("Error Out"=w908:errorcluster)  [unwired: 8 in]
        n442 = Enqueue Element(queue=w910, element=T77 {"Action"=enum."Shift Decay Checkbox", "Data"=variant}, error in (no error)=w908) -> (error out=w906:errorcluster)  [unwired: 1 in, 2 out]
      }
      event "Smoothen Decay": Value Change {
        n443 = event-data() -> ("CtlRef"=w921:refnum<vi>, "NewVal"=w917:bool)  [unwired: 1 in]
        n444 = call "AlliGator Update Settings & Control.vi"("Value"=w917, "Sender"=w920, "CtlRef"=w921) -> ("Error Out"=w915:errorcluster)  [unwired: 8 in]
        n445 = Enqueue Element(queue=w918, element=T77 {"Action"=enum."Smooth Decay Checkbox", "Data"=variant}, error in (no error)=w915) -> (error out=w914:errorcluster)  [unwired: 1 in, 2 out]
      }
      event "SYNC Period": Shortcut Menu Selection (User) {
        n446 = event-data() -> ("CtlRef"=w922:refnum<vi>, "ItemTag"=w923:string)  [unwired: 1 in]
        n447 = case shown="\"Export JSON String to Clipboard\"" w923 {
          tunnel: w922 -> [_ w925 w927]
          frame "", Default {
          }
          frame "Same as Laser Period" {
            n448 = property on="Laser Period" class="DigNum (strict)"() -> ("Value"=w926:dbl[unit])  [unwired: 2 in, 2 out]
            n449 = property class="DigNum (strict)"(reference=w925, "Val(Sgnl)"=w926) -> ()  [unwired: 1 in, 2 out]
          }
          frame "Export JSON String to Clipboard" {
            n450 = call "AlliGator Export Settings Parameter JSON String to Clipboard.vi"("Control Refnum"=w927) -> ()  [unwired: 9 in, 2 out]
          }
        }
      }
      event "Use Current Dataset Parameters": Value Change {
        n451 = event-data() -> ()  [unwired: 1 in, 1 out]
        n452 = Enqueue Element(queue=w929, element=T77 {"Action"=enum."Set SEPL Parameters to Dataset Ones", "Data"=variant}) -> ()  [unwired: 2 in, 3 out]
      }
      event "Use Cursors": Value Change {
        n453 = event-data() -> ("CtlRef"=w939:refnum<vi>, "NewVal"=w931:bool)  [unwired: 1 in]
        n454 = call "AlliGator Update Settings & Control.vi"("Value"=w931, "Sender"=w938, "CtlRef"=w939) -> ("Error Out"=w935:errorcluster)  [unwired: 8 in]
        n455 = Bundle By Name(cluster=T77 {"Action"=enum."Use Cursor (Extrapolate) Checkbox", "Data"=variant} ("element"), "Data"=w931) -> (w932:T77)
        n456 = Enqueue Element(queue=w936, element=w932, error in (no error)=w935) -> (error out=w933:errorcluster)  [unwired: 1 in, 2 out]
      }
      event "Use File Timestamp": Value Change {
        n457 = event-data() -> ("CtlRef"=w947:refnum<vi>, "NewVal"=w943:bool)  [unwired: 1 in]
        n458 = call "AlliGator Update Settings & Control.vi"("Value"=w943, "Sender"=w946, "CtlRef"=w947) -> ("Error Out"=w942:errorcluster)  [unwired: 8 in]
        n459 = Enqueue Element(queue=w944, element=T77 {"Action"=enum."Use File Timestamp Checkbox", "Data"=variant}, error in (no error)=w942) -> (error out=w940:errorcluster)  [unwired: 1 in, 2 out]
      }
      event "Use Fixed ROI Diameter": Value Change {
        n460 = event-data() -> ("CtlRef"=w955:refnum<vi>, "NewVal"=w953:bool)  [unwired: 1 in]
        n461 = call "AlliGator Update Settings & Control.vi"("Value"=w953, "Sender"=w954, "CtlRef"=w955) -> ("Error Out"=w949:errorcluster)  [unwired: 8 in]
        n462 = Enqueue Element(queue=w951, element=T77 {"Action"=enum."Use Fixed ROI Diameter Checkbox", "Data"=variant}, error in (no error)=w949) -> (error out=w948:errorcluster)  [unwired: 1 in, 2 out]
      }
      event "Use Periodicity": Value Change {
        n463 = event-data() -> ("CtlRef"=w964:refnum<vi>, "NewVal"=w956:bool)  [unwired: 1 in]
        n464 = call "AlliGator Update Settings & Control.vi"("Value"=w956, "Sender"=w963, "CtlRef"=w964) -> ("Error Out"=w960:errorcluster)  [unwired: 8 in]
        n465 = Bundle By Name(cluster=T77 {"Action"=enum."Use Periodicity (Extrapolate) Checkbox", "Data"=variant} ("element"), "Data"=w956) -> (w957:T77)
        n466 = Enqueue Element(queue=w961, element=w957, error in (no error)=w960) -> (error out=w958:errorcluster)  [unwired: 1 in, 2 out]
      }
      event "User-Defined Quantity": Shortcut Menu Selection (User) {
        n467 = event-data() -> ("ItemTag"=w965:string)  [unwired: 1 in]
        n468 = case shown="\"User-defined Quantities List\"" w965 {
          frame "", Default {
          }
          frame "User-defined Quantities List" {
            n469 = vi-ref "Formula.lvlib:Aliases Definition Window.vi"() -> (w975:refnum<vi>)
            n470 = property class="VI"(reference=w975) -> (reference out=w974:refnum<vi>, error out=w970:errorcluster, "Path"=w968:path)  [unwired: 1 in]
            n471 = call "Get-Set Reserved Keywords.vi"("Get (F)/Set"=TRUE, "Error In"=w970, "Formula Interpreter Path"=w968, "Reserved Keywords"=T87 ["f_1", "a_1", "<tau>_a", "<tau>_i", "tau_1", "tau_2"] ("Basic Burst Statistics Names")) -> ("Error Out"=w969:errorcluster, "Formula Interpreter Path"=w967:path)  [unwired: 5 in, 1 out]
            n472 = call "Run Vi.vi"("VI Path"=w967, "error in (no error)"=w969) -> ("error out"=w973:errorcluster)  [unwired: 6 in, 1 out]
            n473 = Close Reference(reference=w974, error in (no error)=w973) -> ()  [unwired: 1 out]
          }
        }
      }
      event User Event {
        n474 = event-data() -> ("AlliGator Settings Message"=w986:T89, "Control Label"=w985:string, "Data"=w984:variant, "Sender"=w982:string)  [unwired: 1 in]
        n475 = case shown="\"Refresh Parameter\"" w986 {
          tunnel: w985 -> [_ _ w994 _]
          tunnel: w984 -> [_ _ w995 _]
          tunnel: w983 -> [_ _ w996 _]
          tunnel: w982 -> [_ _ w993 _]
          tunnel: w981 -> [_ _ w992 _]
          tunnel: [_ TRUE ("Discard?") _ _] -> w980
          tunnel: w978 -> [_ w989 _ w1028]
          tunnel: w977 -> [_ w987 _ _]
          frame "Idle", Default {
          }
          frame "Quit" {
            n476 = Unregister For Events(event registration refnum=w987) -> ()  [unwired: 1 in, 1 out]
            n477 = Enqueue Element(queue=w989, element=T77 {"Action"=enum."Quit", "Data"=variant}) -> ()  [unwired: 2 in, 3 out]
          }
          frame "Refresh Parameter" {
            n478 = Equal?(x=w993, y=w992) -> (x = y?=w991:bool)
            n479 = case shown="True" w991 {
              tunnel: w996 -> [w1004 _]
              tunnel: w995 -> [w1002 _]
              tunnel: w994 -> [w1003 _]
              frame False {
                n480 = call "AlliGator Settings Storage.vi"("AlliGator Settings List"=AlliGator_Settings_List."Miscellaneous:Verbose Settings Mode") -> ("Error Out"=w999:errorcluster, "Variant Data out"=w1001:variant)  [unwired: 9 in]
                n481 = call-poly "Variant to Data.vi"("Variant"=w1001) -> ("Value"=w1000:bool)  [unwired: 8 in]
                n482 = call "AlliGator Refresh Single Setting.vi"("Verbose (T)"=w1000, "Error In"=w999, "Data"=w1002, "Control Label"=w1003, "VI Ref in"=w1004) -> ("Error Out"=w1006:errorcluster, "VI Ref (dup)"=w997:refnum<vi>)  [unwired: 5 in]
                n483 = case shown="\"Phasor Graph Frequency\"" w1003 {
                  tunnel: w1002 -> [_ w1011 w1016 w1023]
                  tunnel: w1006 -> [w1007 w1010 w1015 w1022]
                  tunnel: [w1007 w1009 w1014 w1021] -> w1005
                  tunnel: w997 -> [_ w1008 w1013 w1019]
                  frame "False", Default {
                  }
                  frame "Phasor Graph Frequency" {
                    n484 = call "AlliGator Refresh Single Setting.vi"("Error In"=w1010, "Data"=w1011, "Control Label"="Phasor Plot Frequency", "VI Ref in"=w1008) -> ("Error Out"=w1009:errorcluster)  [unwired: 6 in, 1 out]
                  }
                  frame "Phasor Plot Frequency" {
                    n485 = call "AlliGator Refresh Single Setting.vi"("Error In"=w1015, "Data"=w1016, "Control Label"="Phasor Graph Frequency", "VI Ref in"=w1013) -> ("Error Out"=w1014:errorcluster)  [unwired: 6 in, 1 out]
                  }
                  frame "Phasor Frequency" {
                    n486 = call "Clear Error.vi"("Error In"=w1022) -> ("no Error Out"=w1018:errorcluster)  [unwired: 8 in]
                    n487 = call "AlliGator Refresh Single Setting.vi"("Error In"=w1018, "Data"=w1023, "Control Label"="Phasor Graph Frequency", "VI Ref in"=w1019) -> ("Error Out"=w1025:errorcluster)  [unwired: 6 in, 1 out]
                    n488 = call "AlliGator Refresh Single Setting.vi"("Error In"=w1018, "Data"=w1023, "Control Label"="Phasor Plot Frequency", "VI Ref in"=w1019) -> ("Error Out"=w1020:errorcluster)  [unwired: 6 in, 1 out]
                    n489 = Merge Errors(w1025, w1020) -> (w1021:errorcluster)
                  }
                }
                n490 = call "Clear Error.vi"("Error In"=w1005) -> ()  [unwired: 8 in, 1 out]
              }
              frame True {
              }
            }
          }
          frame "Refresh All Parameters" {
            n491 = Enqueue Element(queue=w1028, element=T77 {"Action"=enum."Refresh All Parameters", "Data"=variant}) -> ()  [unwired: 2 in, 3 out]
          }
        }
      }
      event Mouse Down {
        w1029 = TRUE  # Tracking
        n492 = event-data() -> ("CtlRef"=w1031:refnum<vi>)  [unwired: 1 in]
        n493 = register-events(reference=w1033, refnum<vi> refnum ("Guess Parameters"), w1031, w1031) -> (reference out=w1032:refnum<event-registration>)  [unwired: 2 in, 1 out]
      }
      event Mouse Move {
        n494 = event-data() -> ("CtlRef"=w1038:refnum<vi>)  [unwired: 1 in]
        n495 = control-ref of="Guess Parameter Names"() -> (w1037:refnum<vi>)
        n496 = property class="Arr (strict)"(reference=w1038) -> (error out=w1036:errorcluster, "Index Values"=w1035:u32[])  [unwired: 1 in, 1 out]
        n497 = property class="Arr (strict)"(reference=w1037, error in=w1036, "Index Values"=w1035) -> (error out=w1034:errorcluster)  [unwired: 1 out]
      }
      event Mouse Up {
        w1042 = FALSE  # Tracking
        w1041 = refnum<vi> refnum ("Guess Parameters")
        n498 = event-data() -> ("CtlRef"=w1040:refnum<vi>)  [unwired: 1 in]
        n499 = register-events(reference=w1044, w1040, w1041, w1041) -> (reference out=w1043:refnum<event-registration>)  [unwired: 2 in, 1 out]
      }
      event Panel Close? {
        w1045 = TRUE ("Discard?")
        n500 = event-data() -> ()  [unwired: 1 in, 1 out]
        n501 = Unregister For Events(event registration refnum=w1049) -> ()  [unwired: 1 in, 1 out]
        n502 = Enqueue Element(queue=w1047, element=T77 {"Action"=enum."Quit", "Data"=variant}) -> ()  [unwired: 2 in, 3 out]
        n503 = event-data("Discard?"=w1045) -> ()  [unwired: 1 in, 1 out]
      }
      event Timeout {
        n504 = event-data() -> ()  [unwired: 1 in, 3 out]
      }
    }
    n505 = call "AlliGator Check whether Source Image needs update.vi"("Error In"=w334) -> ()  [unwired: 10 in, 1 out]
    n506 = call "AlliGator Check whether Phasor Plot needs update.vi"("Error In"=w334) -> ()  [unwired: 10 in, 1 out]
  }
  n507 = CPU Information() -> (4:w4:i32)  [unwired: 3 out]
  "# Logical Processors" <- w4
  n508 = property on="# Logical Processors Used" class="Digital (strict)"("Maximum"=w4, "Minimum"=w9, "OutOfRngActMin"=w9, "OutOfRngActMax"=w4) -> ()  [unwired: 2 in, 2 out]
  n509 = invoke class="VI" method="FP.Close"(reference=w11) -> (reference out=w23:refnum<vi>, error out=w22:errorcluster)  [unwired: 2 in, 1 out]
  n510 = Close Reference(reference=w23, error in (no error)=w22) -> ()  [unwired: 1 out]
